vi "SISE-Analyser100.vi"() -> ()   [LabVIEW 2024]
uses:
  <vilib>/Analysis/NI_AALPro.lvlib
panel:
  out "Buffer Mobilty ch2":dbl
  out "pKs ch2":dbl
  in  "Main Tab Control":T1(tab)
  out "Event marks":string
  in  "Raw data file in":path
  out "Trace length":dbl
  out "# of traces":dbl
  out "Trace #":dbl
  in  "Scroll back":bool
  in  "Step back":bool
  in  "Step forward":bool
  in  "Scroll forward":bool
  in  "Module selection view data":enum16{"Load data", "Scroll data"}(ring)
  out "Load data":bool
  in  "Scroll speed":dbl(slide)=10.000000000000002 scale=1.0..100.0
  out "Scroll data":bool
  out "SISE 1 channel":bool
  out "Voltage 2 channel":bool
  out "Voltage 1 channel":bool
  out "SISE 2 channel":bool
  out "Scan distance, µm":dbl
  out "Scan angle, degrees":dbl
  out "Record period (single track), s s):":dbl
  out "Position probe":cluster{dbl[], dbl[]}[](graph)
  in  "?":T2(tab)
  out "Vprobe SISE 1":cluster{dbl[], dbl[]}[](graph)
  out "Vprobe SISE 2":cluster{dbl[], dbl[]}[](graph)
  out "Vprobe V 1":cluster{dbl[], dbl[]}[](graph)
  out "Vprobe V 2":cluster{dbl[], dbl[]}[](graph)
  in  "?":enum32{"dV SISE 1", "dV SISE 2"}(tab)
  out "deltaV SISE 1":cluster{dbl[], "Best Linear Fit":dbl[]}[](graph)
  out "deltaV SISE 2":cluster{dbl[], "Best Linear Fit":dbl[]}[](graph)
  in  "Start fit (% of rec. period)":dbl(slide)=50.0 scale=0.0..100.0
  in  "TC 3":T3(tab)
  in  "Range limit\nS1.1 (mV)":dbl(slide)=200.0 min=0.0 max=600.0 scale=0.2..600.0
  in  "Base line\nS1.1 (mV)":dbl(slide) scale=-300.0..300.0
  in  "Range limit\nS1.2 mV":dbl(slide)=30.0 scale=0.03..200.0
  in  "Base line \nS1.2 (mV)":dbl(slide) scale=-15.0..15.0
  out "dV-SISE channel 1":cluster{dbl[], dbl[]}[](graph)
  out "V-SISE channel 1":cluster{dbl[], dbl[]}[](graph)
  out "V-SISE channel 2":cluster{dbl[], dbl[]}[](graph)
  out "dV-SISE channel 2":cluster{dbl[], dbl[]}[](graph)
  in  "Range limit\nS2.1 (mV)":dbl(slide)=200.0 min=0.0 max=600.0 scale=0.2..600.0
  in  "Base line\nS2.1 (mV)":dbl(slide) scale=-300.0..300.0
  in  "Base line \nS2.2 (mV)":dbl(slide) scale=-15.0..15.0
  in  "Range limit\nS2.2 (mV)":dbl(slide)=30.0 scale=0.0..30.0
  out "Voltage channel 1":cluster{dbl[], dbl[]}[](graph)
  in  "Base line\nV1 (V)":dbl(slide) scale=-300.0..300.0
  in  "Range limit\nV1 (V)":dbl(slide)=200.0 min=0.0 max=600.0 scale=0.2..600.0
  in  "Base line\nV2 (V)":dbl(slide) scale=-300.0..300.0
  in  "Range limit\nV2 (V)":dbl(slide)=200.0 min=0.0 max=600.0 scale=0.2..600.0
  out "Voltage channel 2":cluster{dbl[], dbl[]}[](graph)
  in  "Zoom from end":dbl(slide)=100.0 scale=0.0..100.0
  in  "Zoom from start":dbl(slide) scale=0.0..100.0
  in  "Calibration-channel SISE1/2":enum32{"SISE channel 1", "SISE channel 2"}(tab)
  out "Update graphs ch1":bool
  in  "Module selection (Calibration window channel 1)":T4(ring)
  in  "Ion conc. ch1 (mM)":dbl
  out "Valency ch1":dbl
  out "Ion species ch1":bool
  out "Ion mobilty ch1":dbl
  in  "Ion Species ch1":u16(ring) items=["none", "H+", "K+", "NH4+", "Na+", "Cl-", "NO3-", "Ca2+", "Mg2+"]
  out "Calibration ch1":bool
  out "Slope ch1":dbl
  out "Intercept ch1":dbl
  out "?":cluster{dbl[], dbl[]}[](graph)
  out "Point #":dbl[](array[numeric])=[1.0, 2.0, 3.0, 4.0, 5.0]
  in  "Array in":dbl[][](array[numeric])
  out "Geometry ch1":bool caption="Geometry"
  out "Corrected \ndistance ch1":dbl caption="Corrected \ndistance"
  in  "Tab Control Geo 1":enum32{"flat surface", "cylinder", "sphere"}(tab)
  in  "Scan Distance  Flat (µm) 1":dbl
  in  "Scan distance cyl. (µm) 1":dbl caption="Scan distance cyl. (µm)"
  in  "Radius of object cyl. (µm) 1":dbl caption="Radius of object cyl. (µm)"
  in  "Minimum distance to object cyl. (µm) 1":dbl caption="Minimum distance to object cyl. (µm)"
  in  "Minimum distance to object sphere (µm) 1":dbl caption="Minimum distance to object sphere (µm)"
  in  "Radius of object sphere (µm) 1":dbl caption="Radius of object sphere (µm)"
  in  "Scan distance sphere (µm) 1":dbl caption="Scan distance sphere (µm)"
  out "Ion conc. SISE channel 1":cluster{dbl[], dbl[]}[](graph)
  in  "Range limit\nS1.3 (mM)":dbl(slide)=200.0 min=0.0 max=600.0 scale=1e-09..100.0
  in  "Base line\nS1.3 (mM)":dbl(slide) scale=-100.0..100.0
  out "Ion flux SISE channel 1":cluster{dbl[], dbl[]}[](graph)
  in  "Base line \nS1.4":dbl(slide) scale=-15.0..15.0
  in  "Range limit\nS1.4":dbl(slide)=1080.8651170969697 scale=0.03..3000.0
  out "?":string
  in  "Bildlaufleiste":i32(c297)
  in  "Zoom from end (Cal. modul) ch1":dbl(slide)=100.0 caption="Zoom from end" scale=0.0..100.0
  in  "Zoom from start (Cal. modul) ch1":dbl(slide) caption="Zoom from start" scale=0.0..100.0
  out "Update graphs ch2":bool
  in  "Ion conc. ch2 (mM)":dbl
  out "Valency ch2":dbl
  out "Ion species ch2":bool
  out "Ion mobilty ch2":dbl
  in  "Ion Species ch2":u16(ring) items=["none", "H+", "K+", "NH4+", "Na+", "Cl-", "NO3-", "Ca2+", "Mg2+"]
  out "Calibration ch2":bool
  out "Slope ch2":dbl
  out "Intercept ch2":dbl
  out "?":cluster{dbl[], dbl[]}[](graph)
  out "Point # 2":dbl[](array[numeric])=[1.0, 2.0, 3.0, 4.0, 5.0]
  in  "Array in 2":dbl[][](array[numeric])
  out "Geometry 2":bool caption="Geometry"
  out "Corrected \ndistance ch2":dbl caption="Corrected\ndistance"
  in  "Tab Control Geo 2":enum32{"flat surface", "cylinder", "sphere"}(tab)
  in  "Scan Distance  Flat (µm) 2":dbl caption="Scan Distance  Flat (µm)"
  in  "Scan distance cyl. (µm) 2":dbl caption="Scan distance cyl. (µm)"
  in  "Radius of object cyl. (µm) 2":dbl caption="Radius of object cyl. (µm)"
  in  "Minimum distance to object cyl. (µm) 2":dbl caption="Minimum distance to object cyl. (µm)"
  in  "Minimum distance to object sphere (µm) 2":dbl caption="Minimum distance to object sphere (µm)"
  in  "Radius of object sphere (µm) 2":dbl caption="Radius of object sphere (µm)"
  in  "Scan distance sphere (µm) 2":dbl caption="Scan distance sphere (µm)"
  in  "Bildlaufleiste 2":i32(c297)
  out "?":string
  out "Ion conc. SISE channel 2":cluster{dbl[], dbl[]}[](graph)
  in  "Range limit\nS2.3 (mM)":dbl(slide)=200.0 min=0.0 max=600.0 scale=1e-09..600.0
  in  "Base line\nS2.3 (mM)":dbl(slide) scale=-100.0..100.0
  out "Ion flux SISE channel 2":cluster{dbl[], dbl[]}[](graph)
  in  "Base line \nS2.4":dbl(slide) scale=-15.0..15.0
  in  "Range limit\nS2.4":dbl(slide)=1021.2709042717592 scale=0.03..3000.0
  in  "Module selection (Calibration window channel 2)":T4(ring)
  in  "Zoom from end (Cal. modul) 2":dbl(slide)=100.0 caption="Zoom from end" scale=0.0..100.0
  in  "Zoom from start (Cal. modul) 2":dbl(slide) caption="Zoom from start" scale=0.0..100.0
  in  "SISE channel selection (buffer corr.)":T5(tab)
  in  "Module selection ch1 (buffer corr.)":T6(ring)
  out "Buffer species ch1":bool
  out "Buffer conc. ch1":bool
  in  "Select buffer ch1":T7(ring)
  out "Buffer Mobilty ch1":dbl
  out "pKs ch1":dbl
  in  "Buffer conc. ch1 (mM)":dbl
  out "?":string
  in  "Bildlaufleiste 3":i32(c297)
  out "Ion flux (buffer corr.) SISE channel 1":cluster{dbl[], dbl[]}[](graph)
  in  "Base line \nS2.4 3":dbl(slide) scale=-15.0..15.0
  in  "Range limit\nS2.4 3":dbl(slide)=30.0 scale=0.03..5000.0
  out "Update graphs (buffer corr.) ch1":bool
  in  "Zoom from end (Buffer corr. modul) ch1":dbl(slide)=100.0 caption="Zoom from end" scale=0.0..100.0
  in  "Zoom from start (Buffer corr. modul) ch1":dbl(slide) caption="Zoom from start" scale=0.0..100.0
  in  "Module selection ch2 (buffer corr.)":T6(ring)
  out "Buffer species ch2":bool
  out "Buffer conc. ch2":bool
  in  "Buffer conc. ch2 (mM)":dbl
  in  "Range limit\nS2.4 2":dbl(slide)=30.0 scale=0.03..300.0
  in  "Base line \nS2.4 2":dbl(slide) scale=-15.0..15.0
  out "Ion flux (buffer corr.) SISE channel 2":cluster{dbl[], dbl[]}[](graph)
  out "Update graphs (buffer corr.) ch2":bool
  out "?":string
  in  "Bildlaufleiste 4":i32(c297)
  in  "Zoom from start (Buffer corr. modul) ch2":dbl(slide) caption="Zoom from start" scale=0.0..100.0
  in  "Zoom from end (Buffer corr. modul) ch2":dbl(slide)=100.0 caption="Zoom from end" scale=0.0..100.0
  in  "Select buffer ch 2":T7(ring)
  out "Next data file/exit program":bool
  in  "Exit program":bool
  out "Create analysis file":bool
  out "Indicate output":bool[](array[boolean])
  in  "Select output":bool[](array[boolean])=[TRUE, TRUE, TRUE, TRUE, TRUE, TRUE, TRUE, TRUE, TRUE, TRUE, TRUE, TRUE, TRUE, TRUE]
  in  "Analysis output file":path
  out "Raw data file":path
  out "Cluster 3":cluster{string[], bool[]}
  in  "Next data file":bool
  in  "Save data":bool
  out "Save analyses file":bool
  in  "Module selection Save Data":T8(ring)
  # "Event marks"
  # "Point (#)       Conc. (mM )      Vm (mV)"
  # "Event marks"
  # "Point (#)       Conc. (mM )      Vm (mV)"
  # "Event marks"
  # "Event marks"
  # "Output signals available                                                               Select output signals"
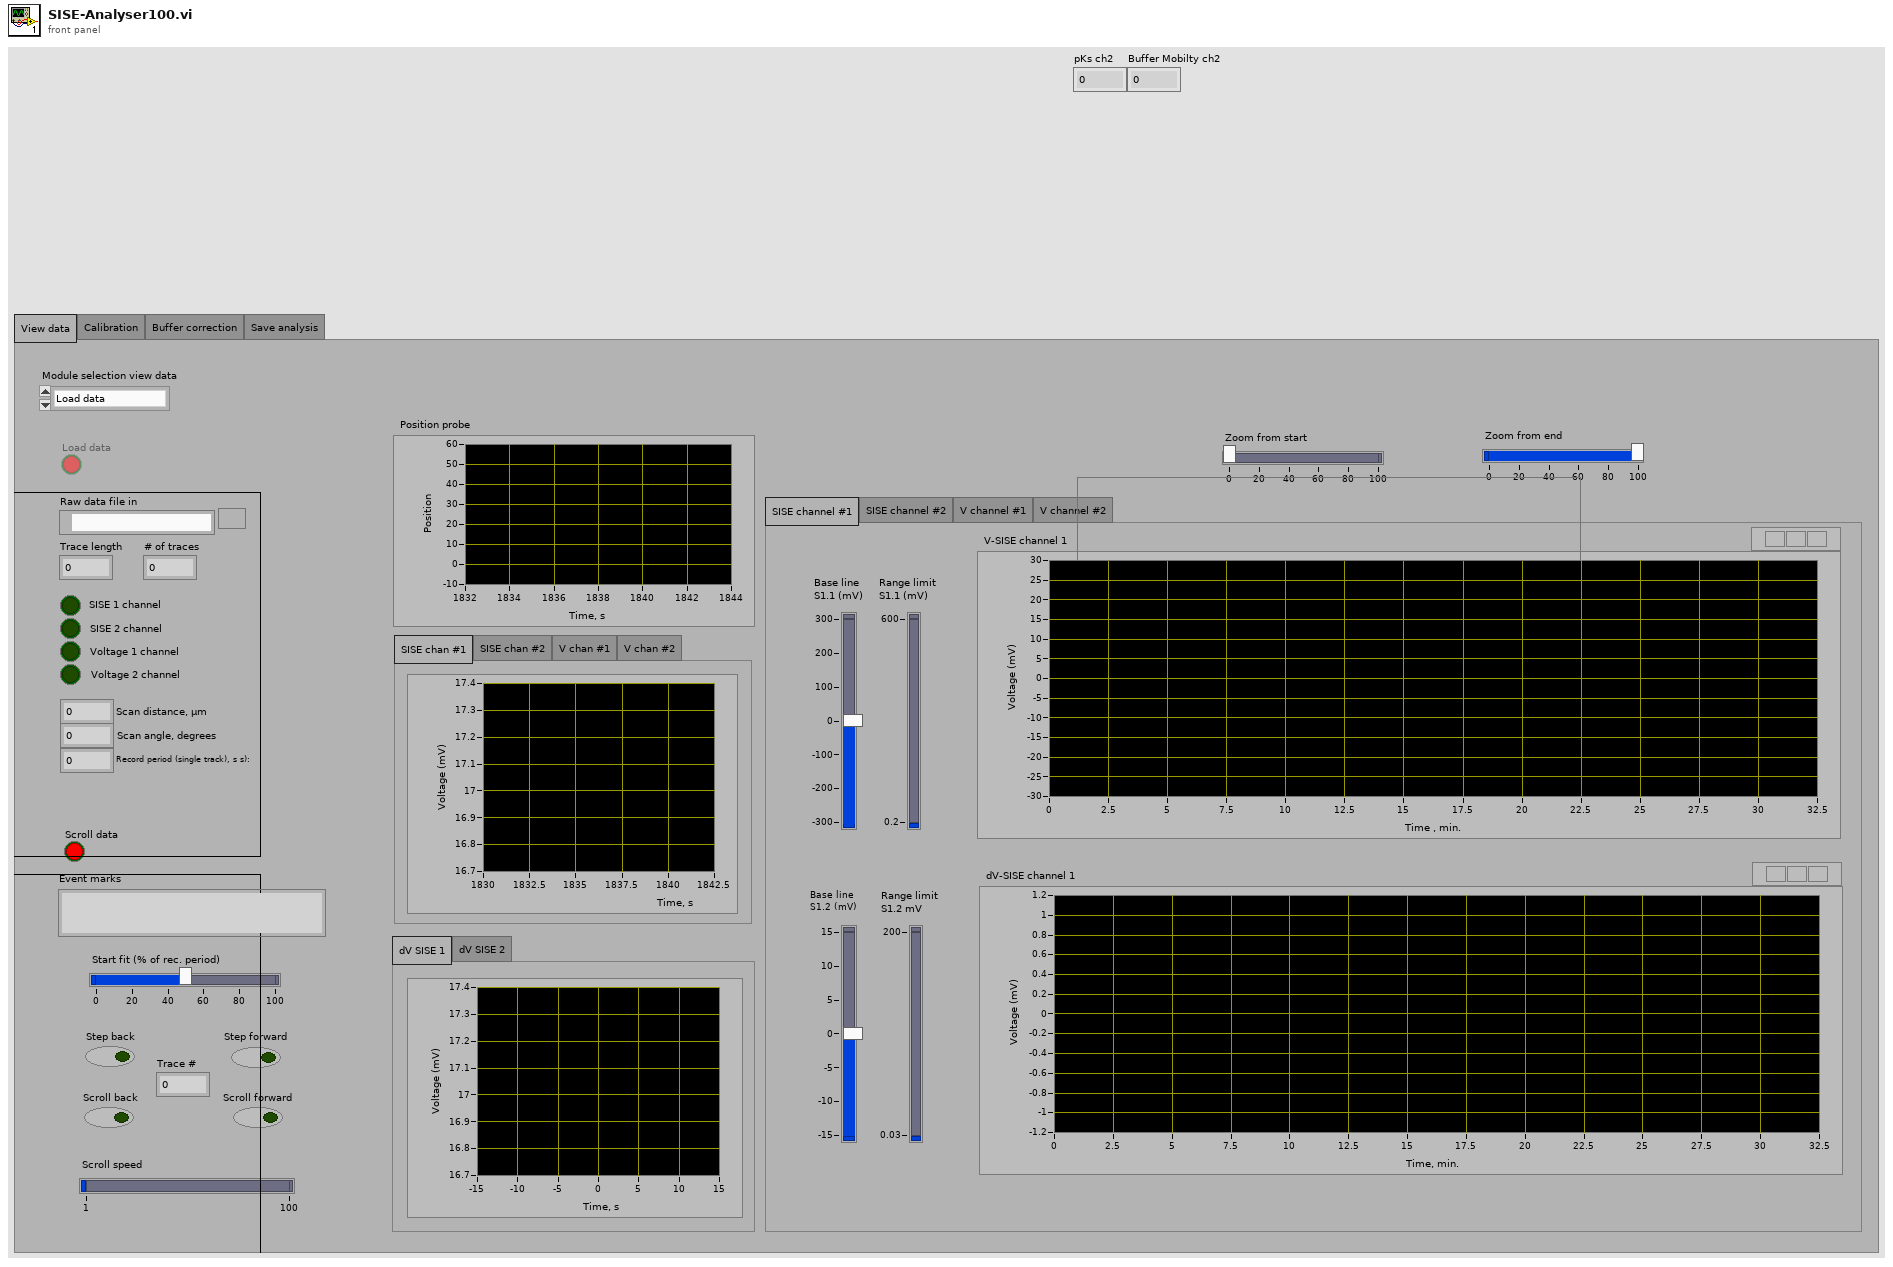
[diagram p1: front panel]
types:
  T1 = enum32{"View data", "Calibration", "Buffer correction", "Save analysis"}
  T2 = enum32{"SISE chan #1", "SISE chan #2", "V chan #1", "V chan #2"}
  T3 = enum32{"SISE channel #1", "SISE channel #2", "V channel #1", "V channel #2"}
  T4 = enum16{"Ion species", "Calibrate", "Geometry", "Update graphs"}
  T5 = enum32{"SISE channel 1, buffer corr.", "SISE channel 2, buffer corr."}
  T6 = enum16{"Buffer species", "Buffer conc.", "Update graphs"}
  T7 = enum16{"none", "Mes", "Malate (pH 5)", "Citrate (pH 5)", "TRIS", "HEPES"}
  T8 = enum16{"Create analysis file", "Save data", "New/stop analysis"}
  T9 = enum8{"Enabled", "Disabled", "Disabled and Grayed Out"}
  T10 = enum16{"open", "replace", "create", "open or create", "replace or create", "replace or create with confirmation"}
  T11 = cluster{path, "Referenz (Ausgang)":refnum<file>, bool, i32, string}
  T12 = cluster{path, "Referenz (Ausgang)":refnum<file>, bool, i32, string}[]
  T13 = cluster{"Raw data file in":path, "refnum out":refnum<file>, "status":bool, "code":i32, "source":string}
  T14 = cluster{dbl[][], dbl[], cluster{string[], bool[]}, dbl[][], cluster{dbl, string}[]}
  T15 = cluster{dbl[], dbl[], "Best Linear Fit":dbl[], dbl[], dbl[]}
  T16 = cluster{"Array (Ausgang)":dbl[], "Array (Ausgang)":dbl[]}
  T17 = cluster{"Array (Ausgang)":dbl[], "Array (Ausgang)":dbl[]}[]
  T18 = cluster{"dup path":path, "refnum":refnum<file>, "status":bool, "code":i32, "source":string}
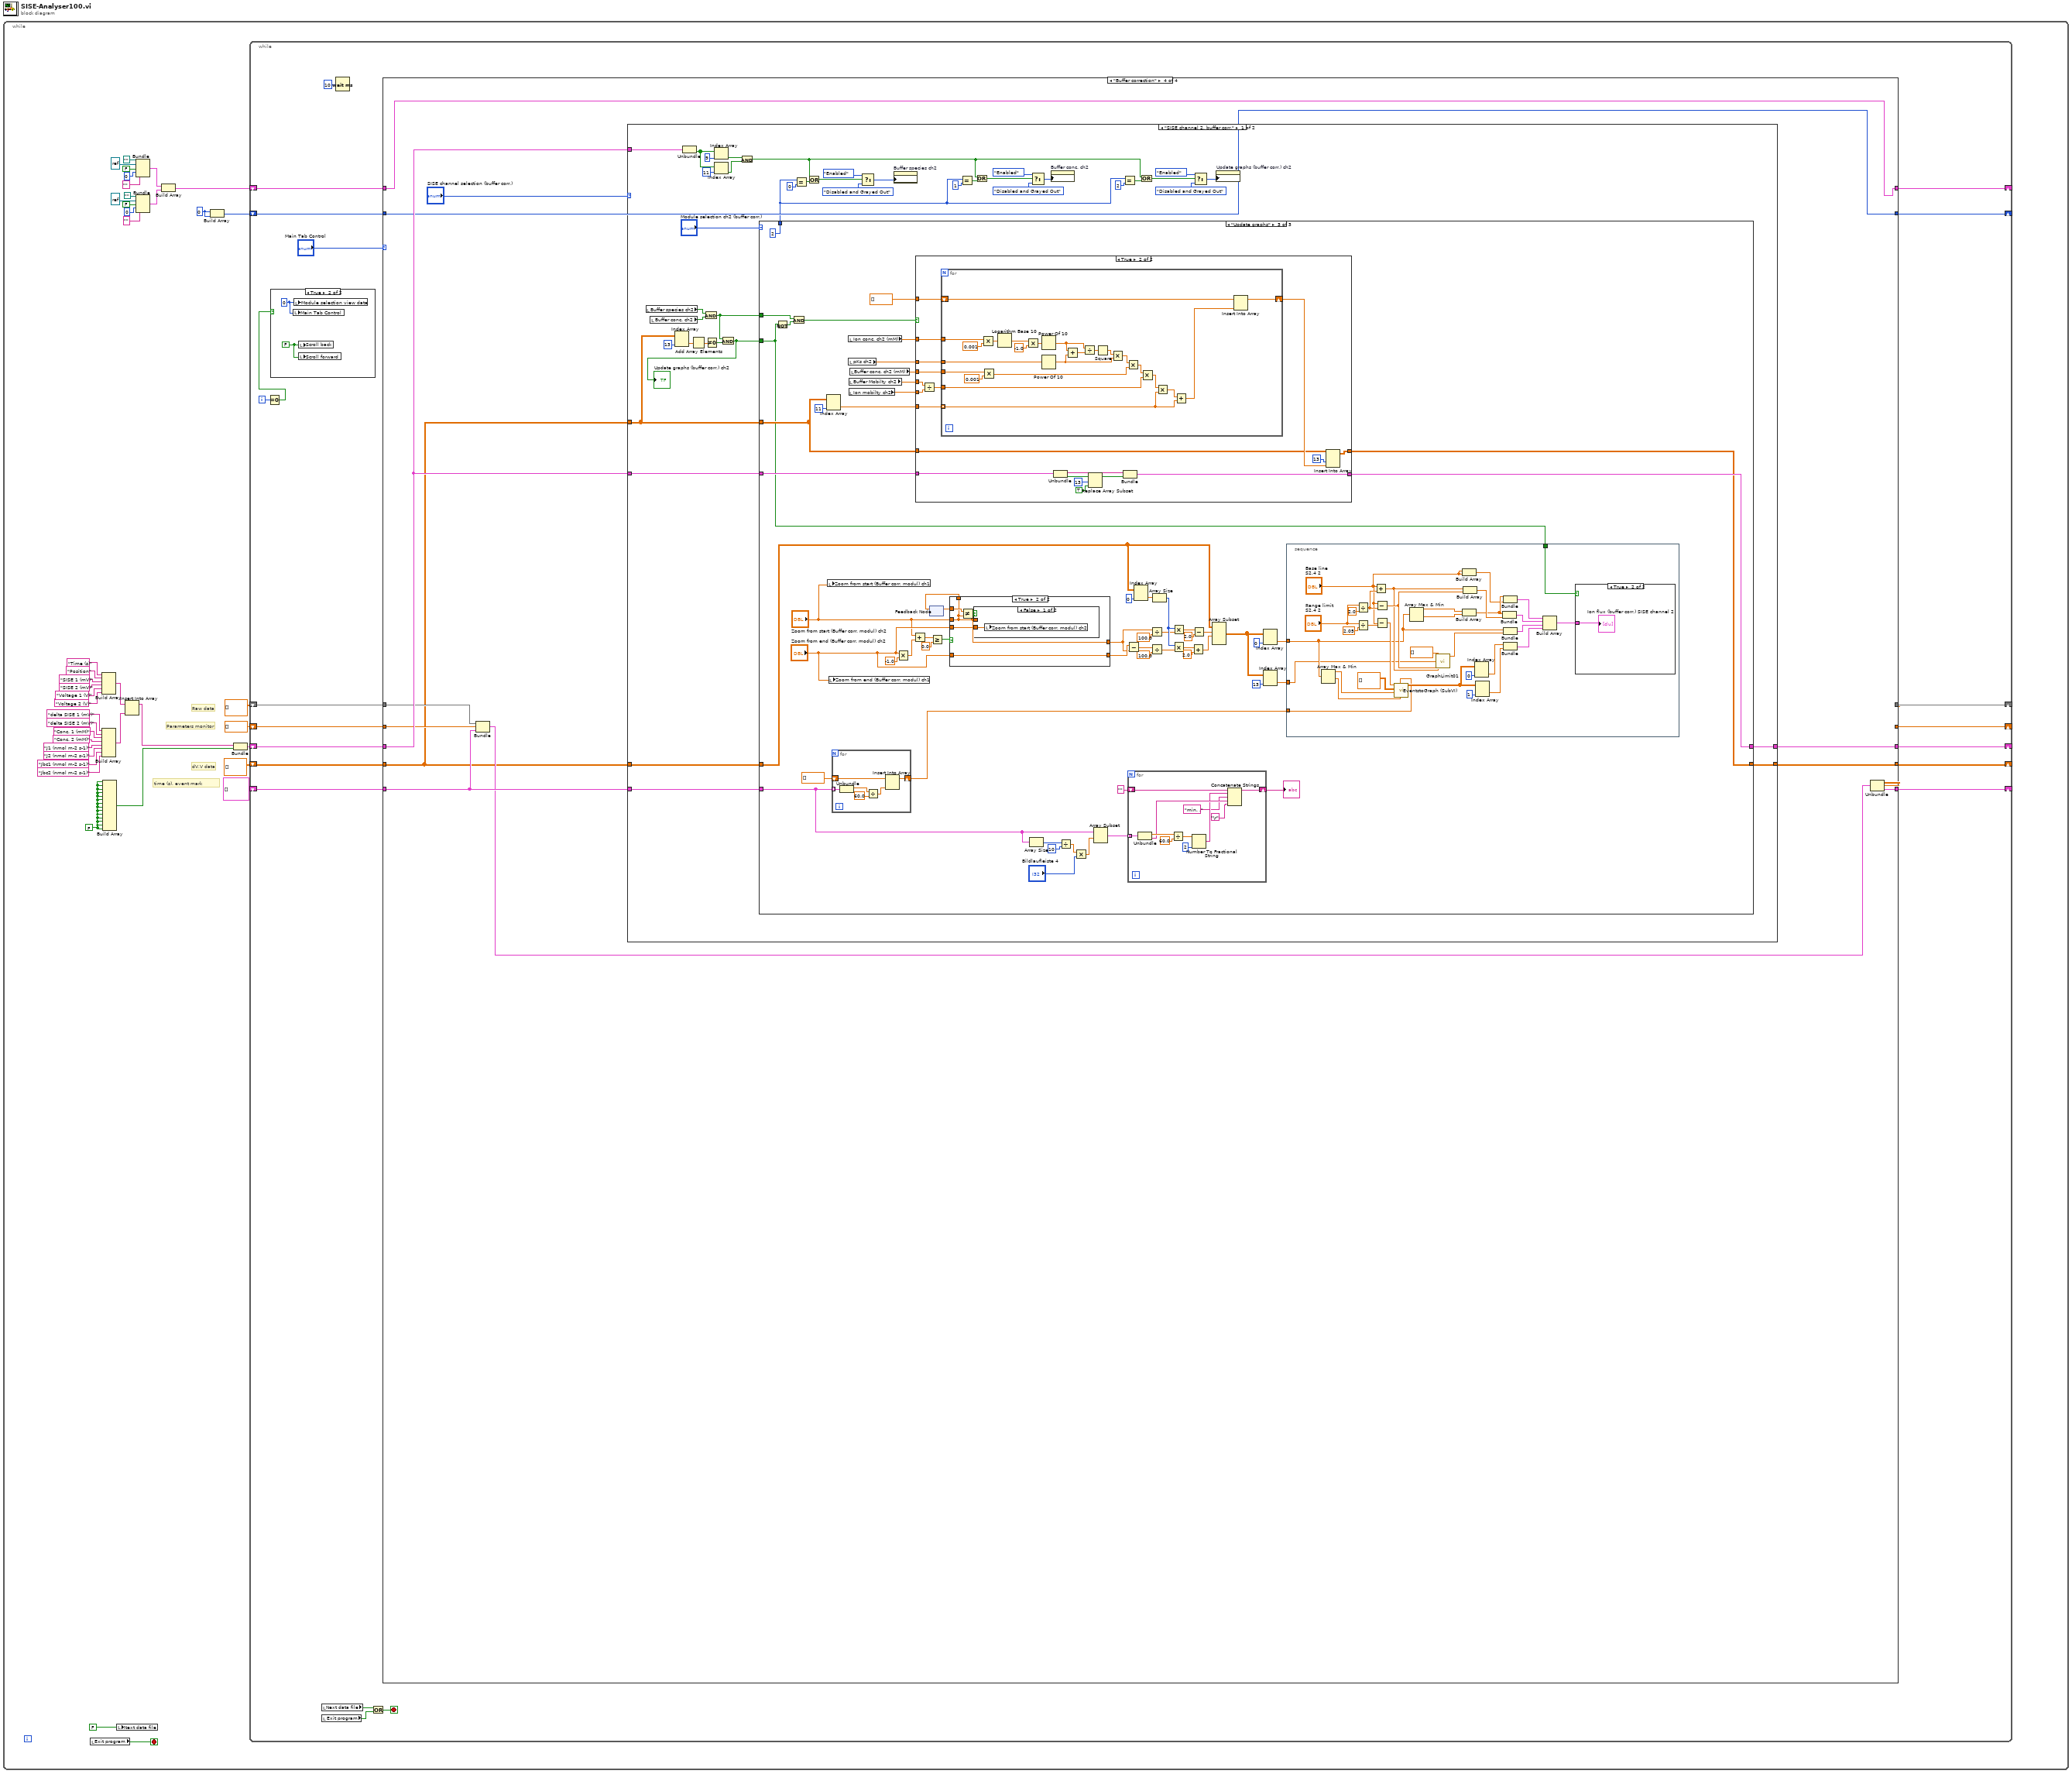
[diagram p0: block diagram]
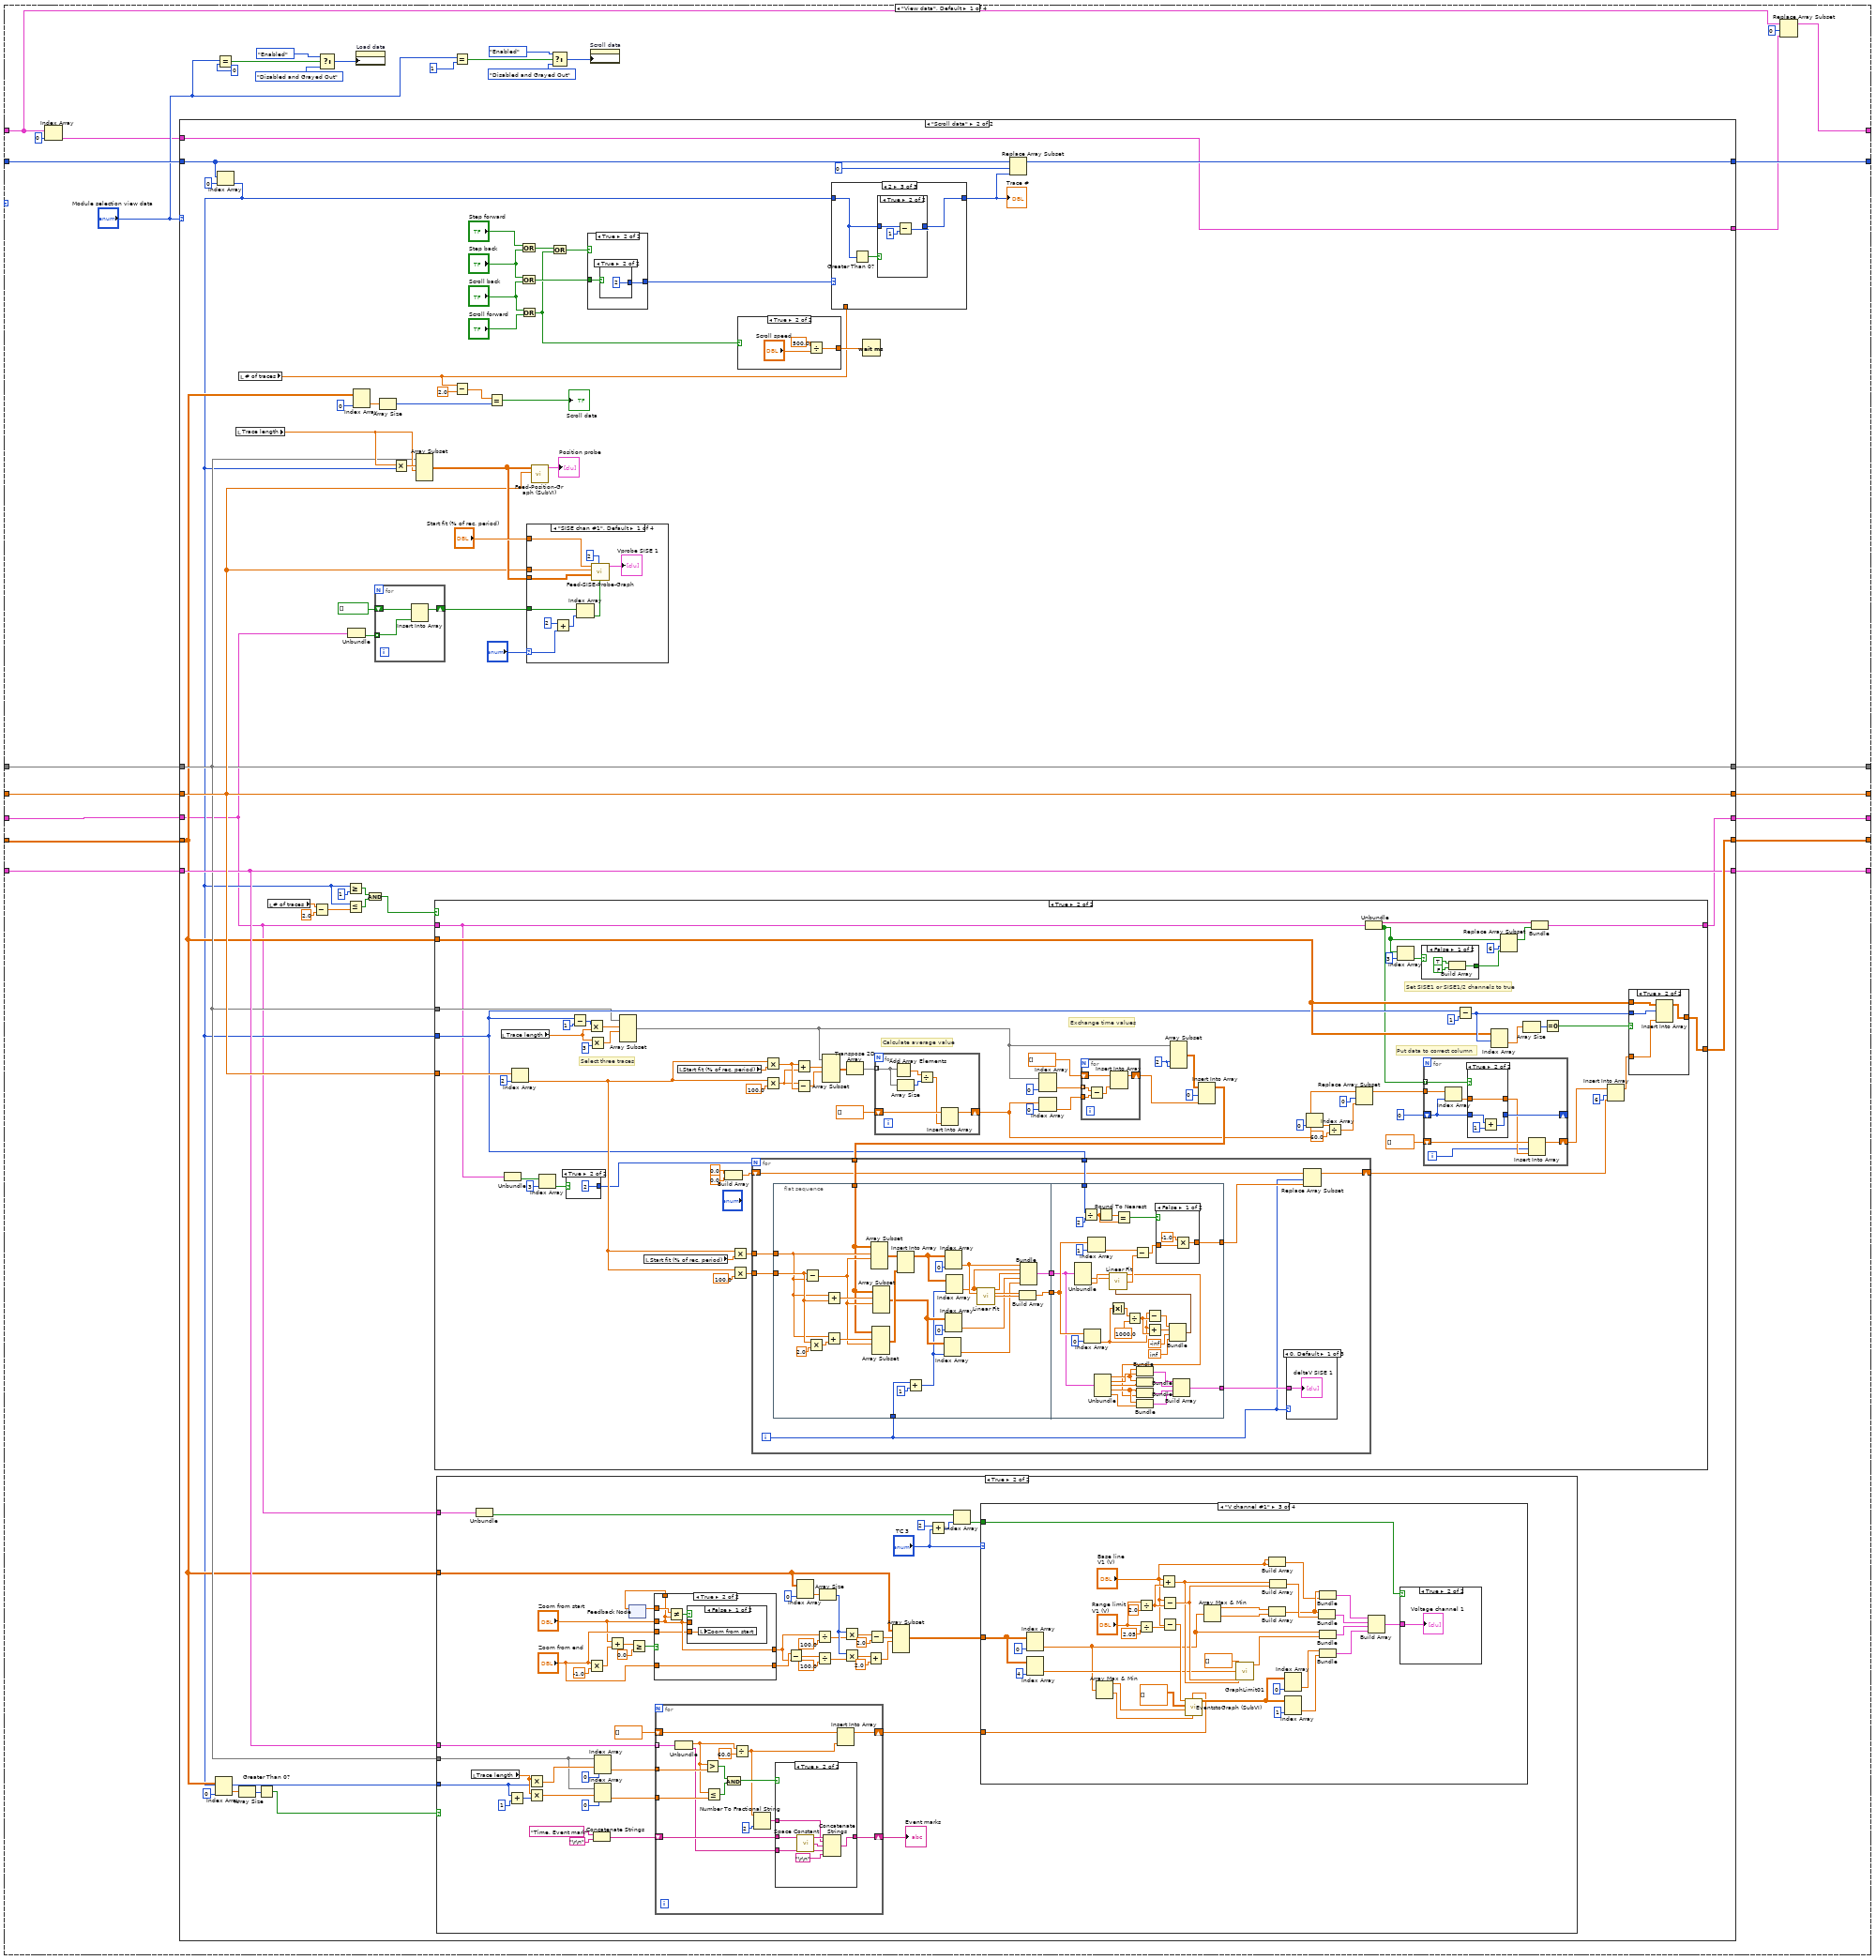
[diagram p3: hidden frame]
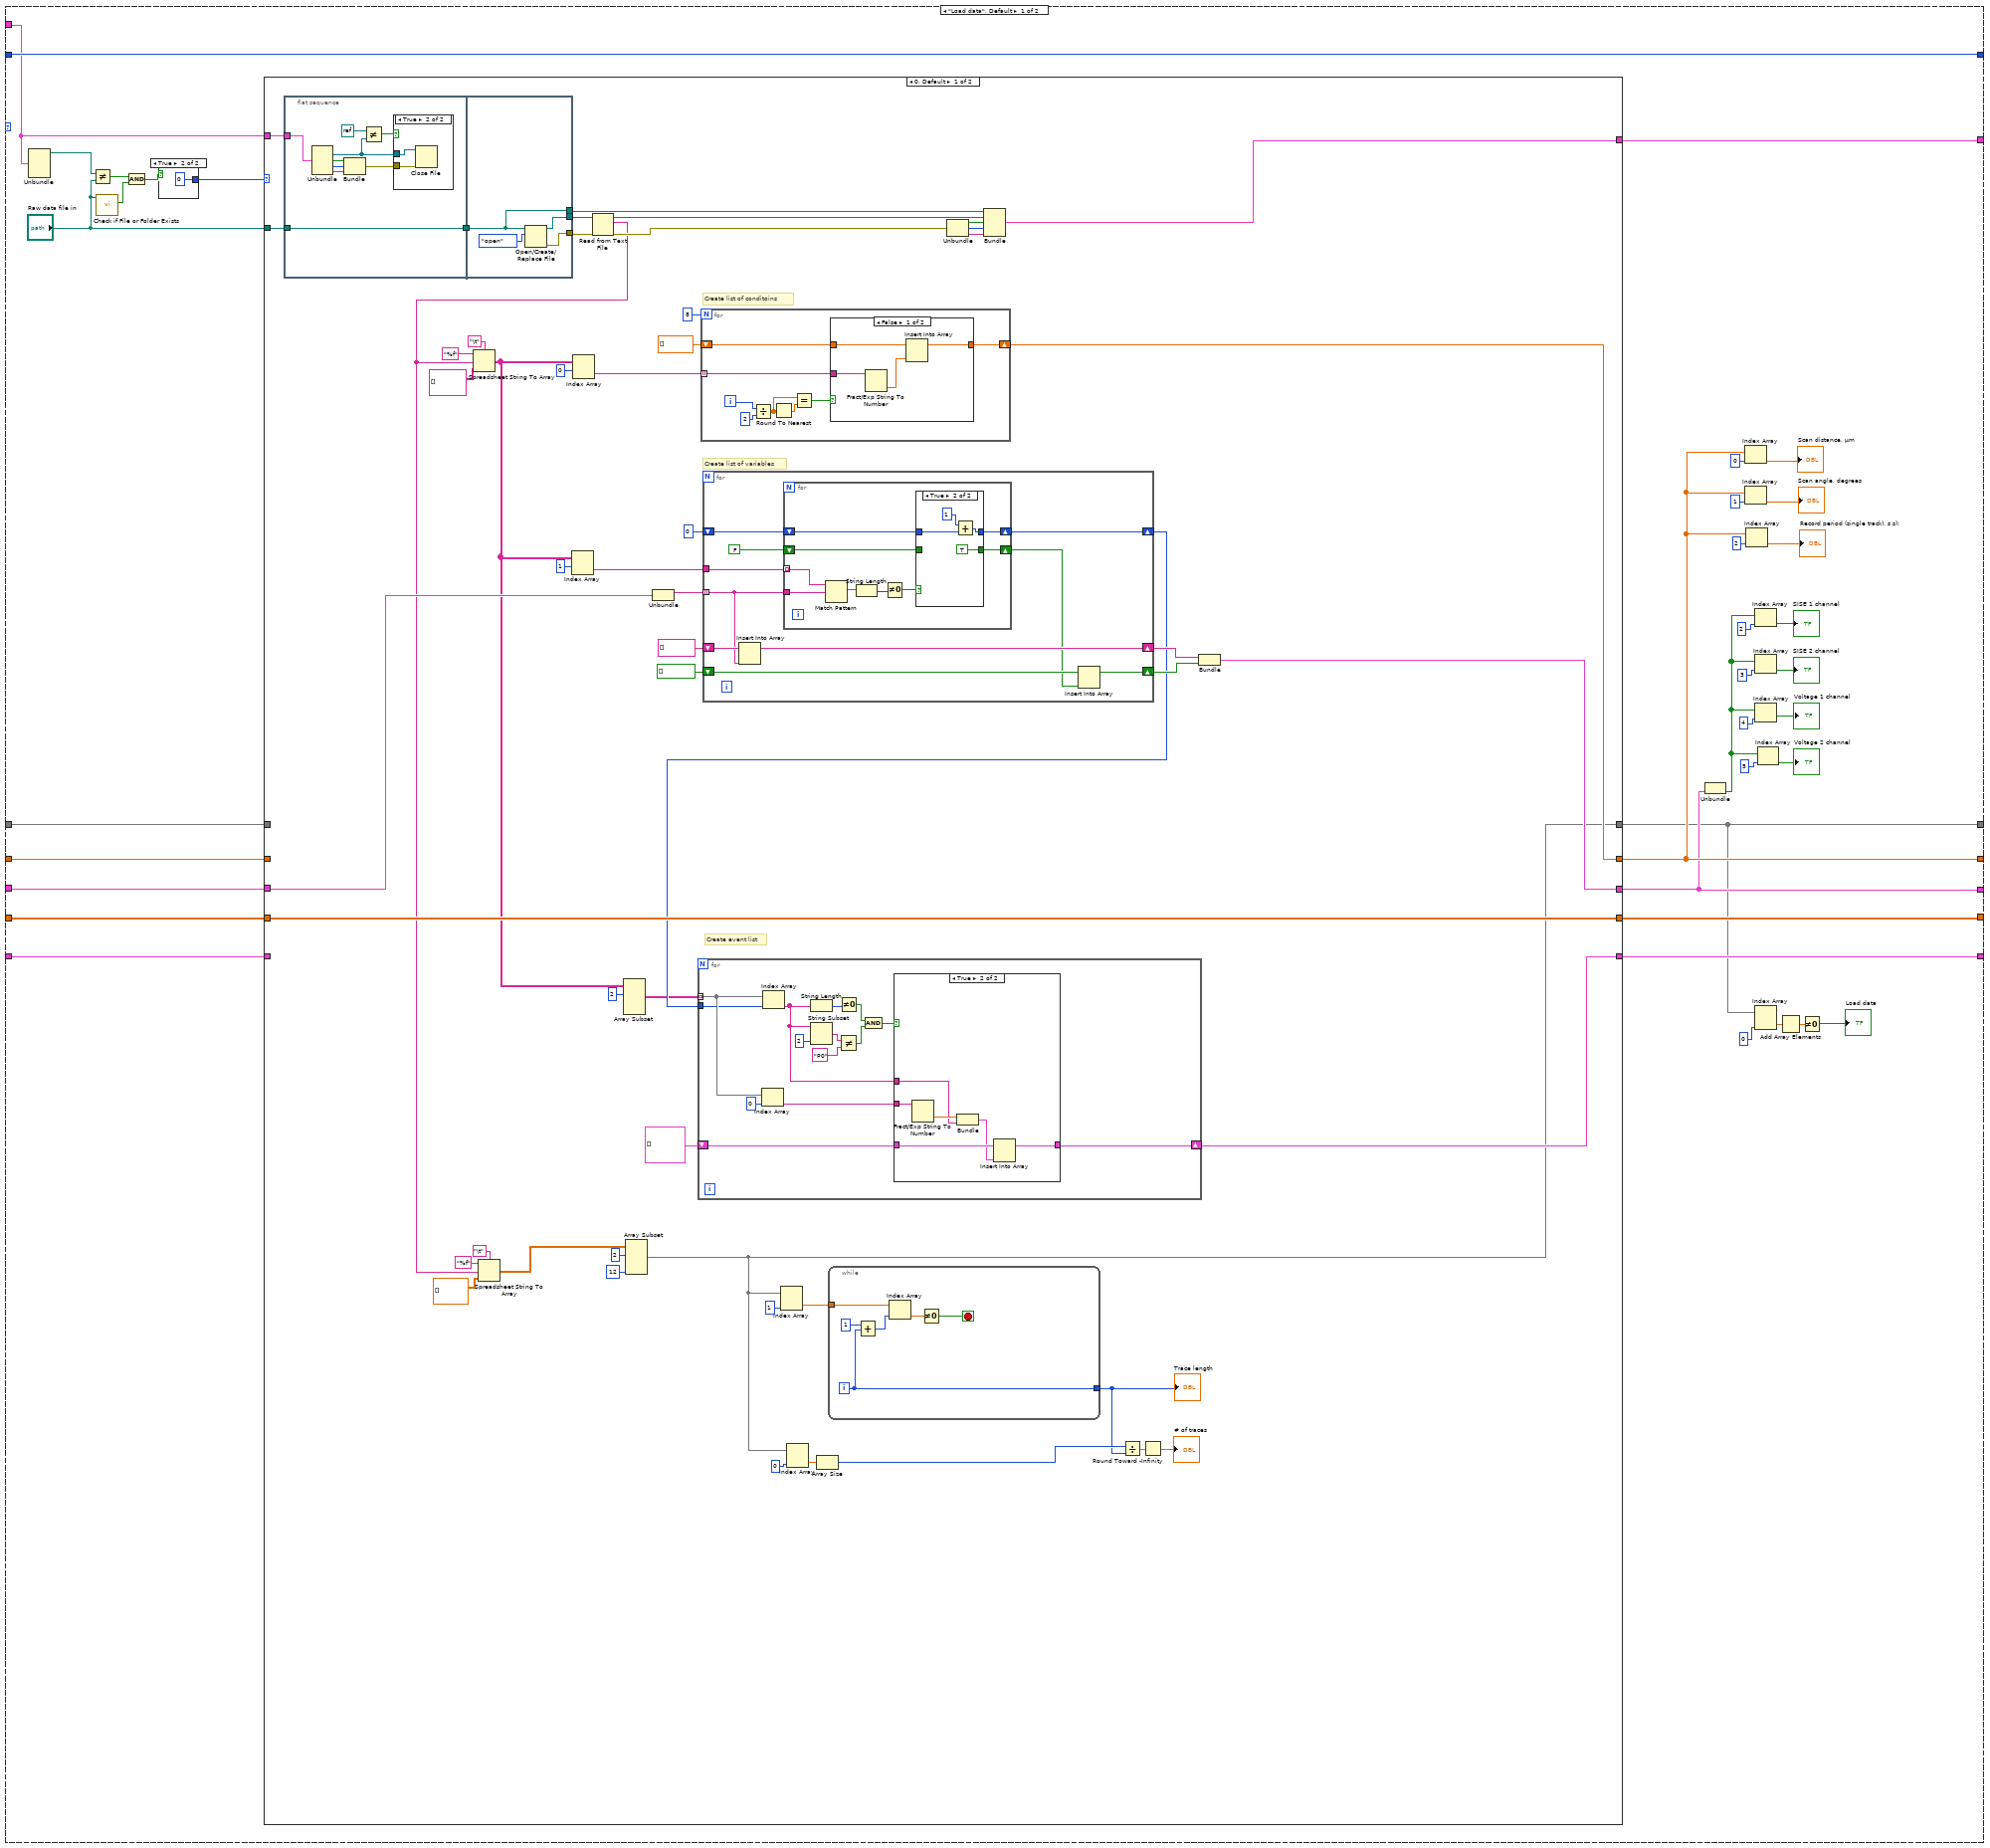
[diagram p4: hidden frame]
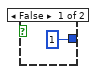
[diagram p5: hidden frame]
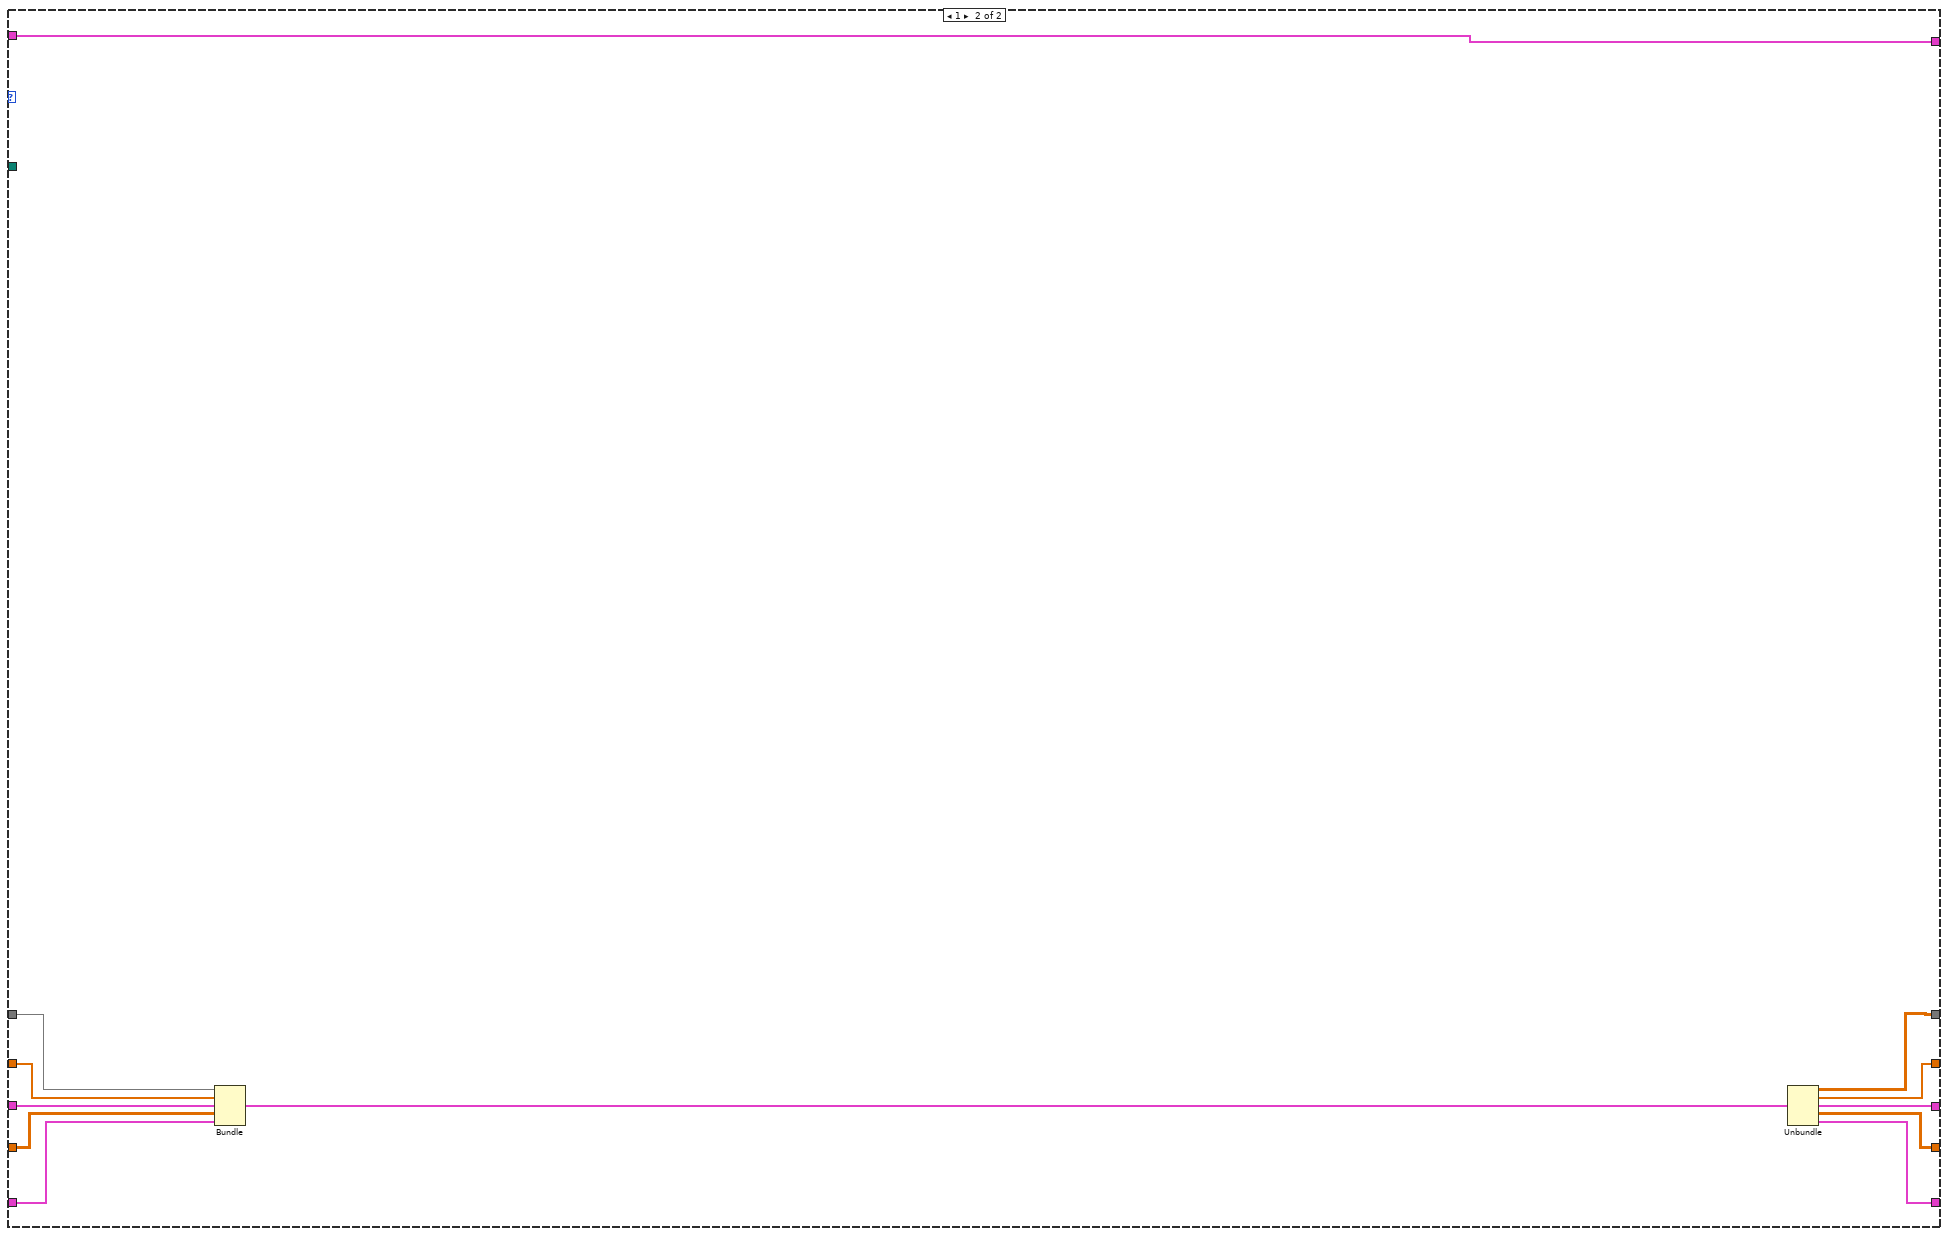
[diagram p10: hidden frame]
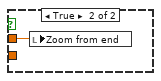
[diagram p13: hidden frame]
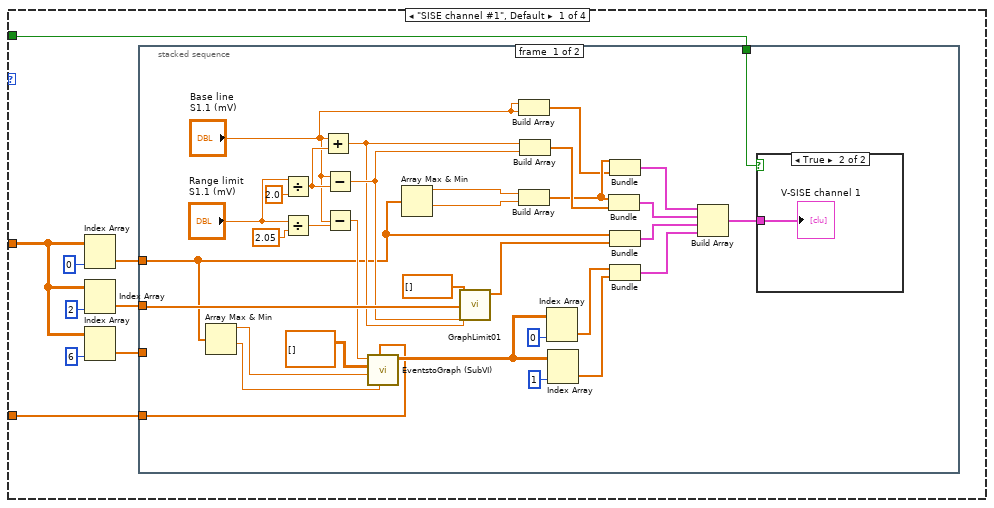
[diagram p14: hidden frame]
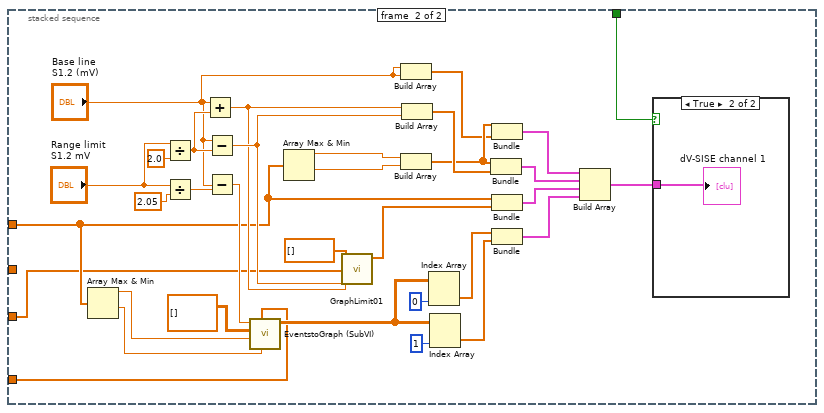
[diagram p16: hidden frame]
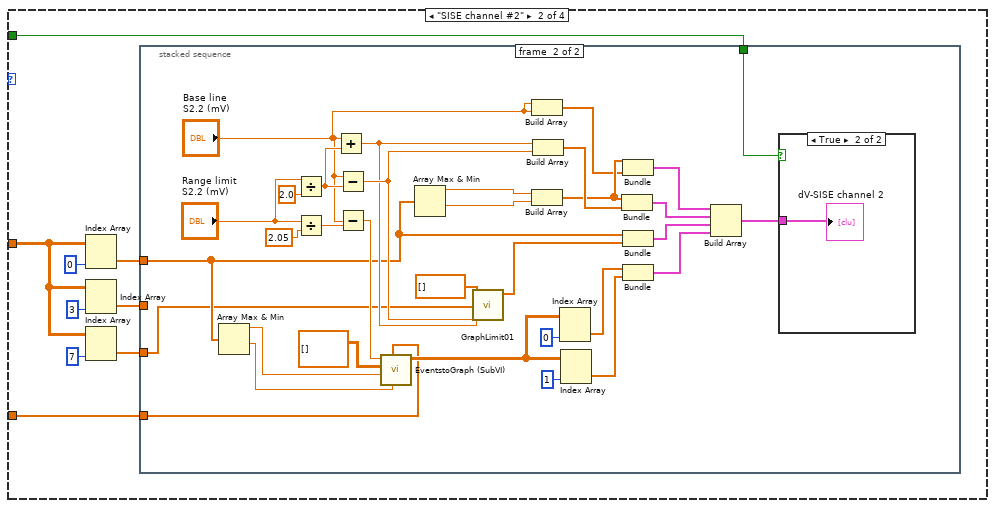
[diagram p18: hidden frame]
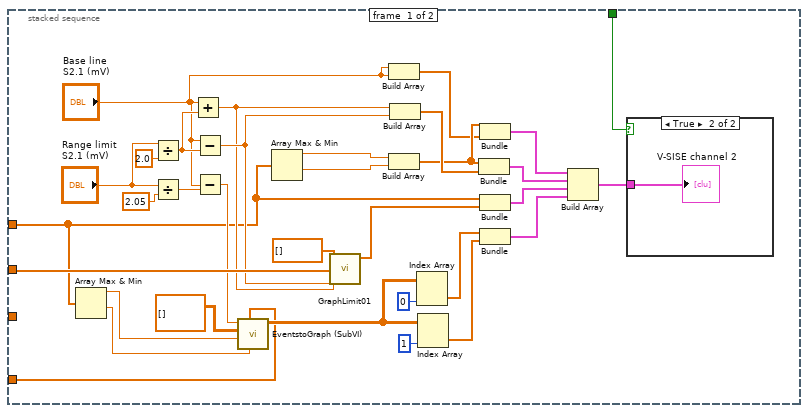
[diagram p19: hidden frame]
diagram:
  n1 = while {
    stop <- w17 stop-if-true
    w19 = FALSE
    w16 = 0
    # "time (s), event mark"
    # "Parameters monitor"
    # "dV,V data"
    # "Raw data"
    n2 = local read "Exit program"() -> (w17:bool)
    n3 = Build Array("Time (s)", "Position", "SISE 1 (mV)", "SISE 2 (mV)", "Voltage 1 (V)", "Voltage 2 (V)") -> (w26:string[])
    n4 = Build Array("delta SISE 1 (mV)", "delta SISE 2 (mV)", "Conc. 1 (mM)", "Conc. 2 (mM)", "J1 (nmol m-2 s-1)", "J2 (nmol m-2 s-1)", "Jbc1 (nmol m-2 s-1)", "Jbc2 (nmol m-2 s-1)") -> (w25:string[])
    n5 = Build Array(w19, w19, w19, w19, w19, w19, w19, w19, w19, w19, w19, w19, w19, w19) -> (w18:bool[])
    n6 = local write "Next data file"(FALSE) -> ()
    n7 = Insert Into Array(array=w26, new element=w25) -> (w20:string[])  [unwired: 1 in]
    n8 = Bundle(path "", "Referenz (Ausgang)"=refnum<file> refnum, FALSE, 0, "") -> (w4:T11)  [unwired: 1 in]
    n9 = Bundle(path "", "Referenz (Ausgang)"=refnum<file> refnum, FALSE, 0, "") -> (w3:T11)  [unwired: 1 in]
    n10 = Build Array(w4, w3) -> (w2:T12)
    n11 = Build Array(w16, w16) -> (w15:i32[])
    n12 = Bundle(w20, w18) -> (w37:cluster{string[], bool[]})  [unwired: 1 in]
    n13 = while {
      shift-right: [w62] -> _
      shift-left: dbl[][] [] -> [w61]
      shift-right: [w58] -> _
      shift-left: dbl[][] [] -> [w59]
      shift-right: [w57] -> _
      shift-left: w37 -> [w42]
      shift-right: [w56] -> _
      shift-left: dbl[] [] -> [w55]
      shift-right: [w51] -> _
      shift-left: w15 -> [w46]
      shift-right: [w54] -> _
      shift-left: cluster{dbl, string}[] [] -> [w53]
      shift-right: [w43] -> _
      shift-left: w2 -> [w52]
      i -> [w45]
      stop <- w50 stop-if-true
      n14 = Equal To 0?(x=w45) -> (x = 0?=w44:bool)
      n15 = case shown="True" w44 {
        frame False {
        }
        frame True {
          w63 = FALSE
          w64 = 0
          n16 = local write "Main Tab Control"(w64) -> ()
          n17 = local write "Module selection view data"(w64) -> ()
          n18 = local write "Scroll back"(w63) -> ()
          n19 = local write "Scroll forward"(w63) -> ()
        }
      }
      n20 = local read "Next data file"() -> (w49:bool)
      n21 = local read "Exit program"() -> (w48:bool)
      n22 = Wait (ms)(milliseconds to wait=u32 10) -> ()  [unwired: 1 out]
      n23 = Or(x=w49, y=w48) -> (x .or. y?=w50:bool)
      n24 = case shown="\"Buffer correction\"" "Main Tab Control" {
        tunnel: w61 -> [w93 w930 w1129 w1813]
        tunnel: [w92 w925 w1135 w1825] -> w62
        tunnel: w59 -> [w73 w933 w1134 w1822]
        tunnel: [w81 w923 w1131 w1817] -> w58
        tunnel: w42 -> [w80 w931 w1124 w1824]
        tunnel: [w79 w927 w1125 w1823] -> w57
        tunnel: w55 -> [w78 w932 w1128 w1821]
        tunnel: [w77 w926 w1130 w1818] -> w56
        tunnel: w46 -> [w72 w916 w1122 w1815]
        tunnel: w53 -> [w76 w929 w1127 w1820]
        tunnel: [w75 w924 w1126 w1816] -> w54
        tunnel: w52 -> [w68 w902 w1123 w1814]
        tunnel: [w66 w900 w1123 w1814] -> w43
        tunnel: [w74 w916 w1122 w1815] -> w51
        frame "View data", Default {
          n25 = Index Array(array=w68, index=0 ("Index")) -> (element=w69:T11)
          n26 = case shown="\"Scroll data\"" "Module selection view data" {
            tunnel: w93 -> [w104 w288]
            tunnel: [w103 w306] -> w92
            tunnel: w73 -> [w127 w300]
            tunnel: [w102 w300] -> w81
            tunnel: w80 -> [w126 w279]
            tunnel: [w110 w287] -> w79
            tunnel: w78 -> [w121 w307]
            tunnel: [w117 w307] -> w77
            tunnel: w72 -> [w113 w283]
            tunnel: [w113 w284] -> w74
            tunnel: w76 -> [w112 w301]
            tunnel: [w111 w301] -> w75
            tunnel: w69 -> [w98 w280]
            tunnel: [w99 w280] -> w65
            frame "Load data", Default {
              n27 = Unbundle(w98) -> (w96:path)  [unwired: 4 out]
              n28 = Not Equal?(x=w96, y="Raw data file in") -> (x != y?=w101:bool)
              n29 = call <vilib>:"Check if File or Folder Exists.vi"("path"="Raw data file in") -> ("file or folder exists?"=w100:bool)  [unwired: 8 in, 2 out]
              n30 = And(x=w101, y=w100) -> (x .and. y?=w94:bool)
              n31 = case shown="True" w94 {
                tunnel: [1 0] -> w95
                frame False {
                }
                frame True {
                }
              }
              n32 = case shown="0, Default" w95 {
                tunnel: w127 -> [_ w276]
                tunnel: [w136 w268] -> w102
                tunnel: w126 -> [w159 w278]
                tunnel: [w158 w272] -> w110
                tunnel: w121 -> [_ w277]
                tunnel: [w167 w271] -> w117
                tunnel: w112 -> [_ w274]
                tunnel: [w155 w269] -> w111
                tunnel: w104 -> [w186 w275]
                tunnel: [w186 w270] -> w103
                tunnel: "Raw data file in" -> [w183 _]
                tunnel: [w179 w267] -> w99
                tunnel: w98 -> [w185 w267]
                frame 0, Default {
                  # "Create list of variables"
                  # "Create list of conditoins"
                  # "Create event list"
                  n33 = flat-sequence {
                    tunnel: w185 -> [w260]
                    tunnel: [w252] -> w184
                    tunnel: w183 -> [w252]
                    tunnel: [w264] -> w176
                    tunnel: [w265] -> w177
                    tunnel: w184 -> [w263]
                    tunnel: [w263] -> w178
                    frame #0 {
                      n34 = Unbundle(w260) -> ("Referenz (Ausgang)"=w253:refnum<file>, w257:bool, w258:i32, w259:string)  [unwired: 1 out]
                      n35 = Bundle(w257, w258, w259) -> (w256:errorcluster)  [unwired: 1 in]
                      n36 = Not Equal?(x=refnum<k0> refnum, y=w253) -> (x != y?=w254:bool)
                      n37 = case shown="True" w254 {
                        tunnel: w256 -> [_ w262]
                        tunnel: w253 -> [_ w261]
                        frame False {
                        }
                        frame True {
                          n38 = Close File(refnum=w261, error in=w262) -> ()  [unwired: 2 out]
                        }
                      }
                    }
                    frame #1 {
                      n39 = Open/Create/Replace File(file path (use dialog)=w263, operation (0:open)=T10."open") -> (refnum out=w265:refnum<file>, error out=w264:errorcluster)  [unwired: 4 in, 1 out]
                    }
                  }
                  n40 = Read from Text File(file (use dialog)=w177, error in=w176) -> (refnum out=w174:refnum<file>, text=w154:string, error out=w175:errorcluster)  [unwired: 2 in, 1 out]
                  n41 = Spreadsheet String To Array(delimiter (Tab)="\t", format string="%f", spreadsheet string=w154, array type (2D Dbl)=string[][] []) -> (array=w156:string[][])
                  n42 = Spreadsheet String To Array(delimiter (Tab)="\t", format string="%f", spreadsheet string=w154, array type (2D Dbl)=dbl[][] []) -> (array=w146:dbl[][])
                  n43 = Index Array(array=w156, index (row)=1 ("Index")) -> (element=w134:string[])  [unwired: 1 in]
                  n44 = Index Array(array=w156, index (row)=0 ("Index")) -> (element=w135:string[])  [unwired: 1 in]
                  n45 = Array Subset(array=w156, index (row)=2 ("Index")) -> (w152:string[][])  [unwired: 3 in]
                  n46 = Array Subset(array=w146, index (row)=2 ("index"), length (col)=12 ("Länge")) -> (w136:dbl[][])  [unwired: 2 in]
                  n47 = Unbundle(w159) -> (w164:string[])  [unwired: 1 out]
                  n48 = for {
                    N: 8 -> [_]
                    tunnel: w135 -> [w241] mode=indexing
                    shift-right: [w239] -> w167
                    shift-left: dbl[] [] -> [w240]
                    i -> [w246]
                    n49 = Divide(x=w246, y=2) -> (x/y=w243:dbl)
                    n50 = Round To Nearest(number=w243) -> (nearest integer value=w244:dbl)
                    n51 = Equal?(x=w243, y=w244) -> (x = y?=w242:bool)
                    n52 = case shown="False" w242 {
                      tunnel: w241 -> [w248 _]
                      tunnel: w240 -> [w250 w251]
                      tunnel: [w249 w251] -> w239
                      frame False {
                        n53 = Fract/Exp String To Number(string=w248) -> (number=w247:dbl)  [unwired: 3 in, 1 out]
                        n54 = Insert Into Array(array=w250, new element=w247) -> (w249:dbl[])  [unwired: 1 in]
                      }
                      frame True {
                      }
                    }
                  }
                  n55 = for {
                    tunnel: w164 -> [w217] mode=indexing
                    tunnel: w134 -> [w223]
                    shift-right: [w216] -> w160
                    shift-left: bool[] [] -> [w215]
                    shift-right: [w220] -> w157
                    shift-left: 0 -> [w221]
                    shift-right: [w219] -> w161
                    shift-left: string[] [] -> [w218]
                    n56 = Insert Into Array(array=w218, new element=w217) -> (w219:string[])  [unwired: 1 in]
                    n57 = for {
                      tunnel: w223 -> [w232] mode=indexing
                      tunnel: w217 -> [w231]
                      shift-right: [w226] -> w214
                      shift-left: FALSE -> [w228]
                      shift-right: [w224] -> w220
                      shift-left: w221 -> [w225]
                      n58 = Match Pattern(string=w232, regular expression=w231) -> (match substring=w230:string)  [unwired: 1 in, 3 out]
                      n59 = String Length(string=w230) -> (length=w229:i32)
                      n60 = Not Equal To 0?(x=w229) -> (x != 0?=w227:bool)
                      n61 = case shown="True" w227 {
                        tunnel: w228 -> [w234 _]
                        tunnel: [w234 TRUE] -> w226
                        tunnel: w225 -> [w233 w235]
                        tunnel: [w233 w237] -> w224
                        frame False {
                        }
                        frame True {
                          n62 = Add(x=1 ("y"), y=w235) -> (x+y=w237:i32)
                        }
                      }
                    }
                    n63 = Insert Into Array(array=w215, new element=w214) -> (w216:bool[])  [unwired: 1 in]
                  }
                  n64 = for {
                    tunnel: w152 -> [w197] mode=indexing
                    tunnel: w157 -> [w193]
                    shift-right: [w194] -> w155
                    shift-left: cluster{dbl, string}[] [] -> [w195]
                    n65 = Index Array(array=w197, index=0 ("Index")) -> (element=w196:string)
                    n66 = Index Array(array=w197, index=w193) -> (element=w199:string)
                    n67 = String Subset(string=w199, length (rest)=2 ("Länge (Rest)")) -> (substring=w204:string)  [unwired: 1 in]
                    n68 = String Length(string=w199) -> (length=w206:i32)
                    n69 = Not Equal?(x=w204, y="P0") -> (x != y?=w200:bool)
                    n70 = Not Equal To 0?(x=w206) -> (x != 0?=w202:bool)
                    n71 = And(x=w202, y=w200) -> (x .and. y?=w201:bool)
                    n72 = case shown="True" w201 {
                      tunnel: w199 -> [_ w211]
                      tunnel: w196 -> [_ w213]
                      tunnel: [w207 w210] -> w194
                      tunnel: w195 -> [w207 w209]
                      frame False {
                      }
                      frame True {
                        n73 = Fract/Exp String To Number(string=w213) -> (number=w212:dbl)  [unwired: 3 in, 1 out]
                        n74 = Bundle(w212, w211) -> (w208:cluster{dbl, string})  [unwired: 1 in]
                        n75 = Insert Into Array(array=w209, new element=w208) -> (w210:cluster{dbl, string}[])  [unwired: 1 in]
                      }
                    }
                  }
                  n76 = Index Array(array=w136, index (col)=1 ("disabled index (col)")) -> (element=w143:dbl[])  [unwired: 1 in]
                  n77 = Index Array(array=w136, index (col)=0 ("disabled index (col)")) -> (element=w141:dbl[])  [unwired: 1 in]
                  n78 = Array Size(array=w141) -> (size(s)=w140:i32)
                  n79 = while {
                    tunnel: w143 -> [w192]
                    tunnel: [w187] -> w138
                    i -> [w187]
                    stop <- w188 stop-if-true
                    n80 = Add(x=1, y=w187) -> (x+y=w191:i32)
                    n81 = Index Array(array=w192, index=w191) -> (element=w189:dbl)
                    n82 = Not Equal To 0?(x=w189) -> (x != 0?=w188:bool)
                  }
                  "Trace length" <- w138
                  n83 = Unbundle(w175) -> ("status"=w180:bool, "code"=w181:i32, "source"=w182:string)
                  n84 = Bundle("Raw data file in"=w178, "refnum out"=w174, "status"=w180, "code"=w181, "source"=w182) -> (w179:T13)  [unwired: 1 in]
                  n85 = Divide(x=w140, y=w138) -> (x/y=w139:dbl)
                  n86 = Round Toward -Infinity(1:w139) -> (0:→"# of traces":dbl)
                  n87 = Bundle(w161, w160) -> (w158:cluster{string[], bool[]})  [unwired: 1 in]
                }
                frame 1 {
                  n88 = Bundle(w276, w277, w278, w275, w274) -> (w273:T14)  [unwired: 1 in]
                  n89 = Unbundle(w273) -> (w268:dbl[][], w271:dbl[], w272:cluster{string[], bool[]}, w270:dbl[][], w269:cluster{dbl, string}[])
                }
              }
              n90 = Unbundle(w110) -> (w109:bool[])  [unwired: 1 out]
              n91 = Index Array(array=w117, index=0) -> (element=→"Scan distance, µm":dbl)
              n92 = Index Array(array=w117, index=1) -> (element=→"Scan angle, degrees":dbl)
              n93 = Index Array(array=w117, index=2) -> (element=→"Record period (single track), s s):":dbl)
              n94 = Index Array(array=w109, index=2) -> (element=→"SISE 1 channel":bool)
              n95 = Index Array(array=w102, index (col)=0 ("disabled index (col)")) -> (element=w130:dbl[])  [unwired: 1 in]
              n96 = Index Array(array=w109, index=3) -> (element=→"SISE 2 channel":bool)
              n97 = Index Array(array=w109, index=4) -> (element=→"Voltage 1 channel":bool)
              n98 = Index Array(array=w109, index=5) -> (element=→"Voltage 2 channel":bool)
              n99 = Add Array Elements(numeric array=w130) -> (sum=w129:dbl)
              n100 = Not Equal To 0?(x=w129) -> (x != 0?=→"Load data":bool)
            }
            frame "Scroll data" {
              n101 = Index Array(array=w288, index (col)=0 ("Deaktivierter Index (Spalte)")) -> (element=w298:dbl[])  [unwired: 1 in]
              n102 = Index Array(array=w283, index=0 ("Index")) -> (element=w285:i32)
              n103 = local read "Trace length"() -> (w315:dbl)
              n104 = Array Size(array=w298) -> (size(s)=w297:i32)
              n105 = local read "# of traces"() -> (w305:dbl)
              n106 = Greater Than 0?(x=w297) -> (x > 0?=w296:bool)
              n107 = local read "# of traces"() -> (w289:dbl)
              n108 = Subtract(x=w289, y=2.0) -> (x-y=w293:dbl)
              n109 = Greater Or Equal?(x=w285, y=1) -> (x >= y?=w292:bool)
              n110 = Less Or Equal?(x=w285, y=w293) -> (x <= y?=w291:bool)
              n111 = Unbundle(w279) -> (w295:bool[])  [unwired: 1 out]
              n112 = Index Array(array=w288, index (col)=0 ("Deaktivierter Index (Spalte)")) -> (element=w320:dbl[])  [unwired: 1 in]
              n113 = And(x=w292, y=w291) -> (x .and. y?=w290:bool)
              n114 = for {
                shift-right: [w837] -> w309
                shift-left: bool[] [] -> [w836]
                tunnel: w295 -> [w835] mode=indexing
                n115 = Insert Into Array(array=w836, new element=w835) -> (w837:bool[])  [unwired: 1 in]
              }
              n116 = Array Size(array=w320) -> (size(s)=w303:i32)
              n117 = Multiply(x=w315, y=w285) -> (x*y=w316:dbl)
              n118 = Array Subset(array=w300, index (row)=w316, length (row)=w315) -> (w311:dbl[][])  [unwired: 2 in]
              n119 = case shown="True" w290 {
                tunnel: w300 -> [_ w662]
                tunnel: w285 -> [_ w663]
                tunnel: w307 -> [_ w703]
                tunnel: w288 -> [w643 w667]
                tunnel: [w643 w677] -> w306
                tunnel: w279 -> [w642 w655]
                tunnel: [w642 w651] -> w287
                frame False {
                }
                frame True {
                  w689 = 2 ("Index")
                  # "Put data to correct column"
                  # "Set SISE1 or SISE1/2 channels to true"
                  # "Exchange time values"
                  # "Calculate average value"
                  # "Select three traces"
                  n120 = local read "Trace length"() -> (w674:dbl)
                  n121 = Unbundle(w655) -> (w661:bool[])  [unwired: 1 out]
                  n122 = Index Array(array=w703, index=2 ("Index")) -> (element=w690:dbl)
                  n123 = Index Array(array=w661, index=3 ("Index")) -> (element=w660:bool)
                  n124 = case shown="True" w660 {
                    tunnel: [1 2] -> w672
                    frame False {
                    }
                    frame True {
                    }
                  }
                  n125 = Subtract(x=w663, y=1) -> (x-y=w713:i32)
                  n126 = Multiply(x=w713, y=w674) -> (x*y=w712:dbl)
                  n127 = Multiply(x=w674, y=3) -> (x*y=w710:dbl)
                  n128 = Array Subset(array=w662, index (row)=w712, length (row)=w710) -> (w669:dbl[][])  [unwired: 2 in]
                  n129 = local read "Start fit (% of rec. period)"() -> (w694:dbl)
                  n130 = local read "Start fit (% of rec. period)"() -> (w701:dbl)
                  n131 = Build Array(0.0 ("Element"), 0.0 ("Element")) -> (w664:dbl[])
                  n132 = Multiply(x=w690, y=w694) -> (x*y=w692:dbl)
                  n133 = Multiply(x=w690, y=100.0) -> (x*y=w691:dbl)
                  n134 = Multiply(x=w690, y=w701) -> (x*y=w708:dbl)
                  n135 = Multiply(x=w690, y=100.0) -> (x*y=w707:dbl)
                  n136 = Add(x=w708, y=w707) -> (x+y=w709:dbl)
                  n137 = Subtract(x=w707, y=w708) -> (x-y=w705:dbl)
                  n138 = Array Subset(array=w669, index (row)=w709, length (row)=w705) -> (w704:dbl[][])  [unwired: 2 in]
                  n139 = Transpose 2D Array(2D array=w704) -> (transposed array=w649:dbl[][])
                  n140 = for {
                    tunnel: w649 -> [w832] mode=indexing
                    shift-right: [w831] -> w659
                    shift-left: dbl[] [] -> [w830]
                    n141 = Add Array Elements(numeric array=w832) -> (sum=w833:dbl)
                    n142 = Array Size(array=w832) -> (size(s)=w834:i32)
                    n143 = Divide(x=w833, y=w834) -> (x/y=w829:dbl)
                    n144 = Insert Into Array(array=w830, new element=w829) -> (w831:dbl[])  [unwired: 1 in]
                  }
                  n145 = Index Array(array=w669, index (col)=0 ("Deaktivierter Index (Spalte)")) -> (element=w697:dbl[])  [unwired: 1 in]
                  n146 = Index Array(array=w659, index=0 ("Index (Spalte)")) -> (element=w695:dbl)
                  n147 = for {
                    tunnel: w695 -> [w825]
                    shift-right: [w828] -> w686
                    shift-left: dbl[] [] -> [w827]
                    tunnel: w697 -> [w824] mode=indexing
                    n148 = Subtract(x=w824, y=w825) -> (x-y=w826:dbl)
                    n149 = Insert Into Array(array=w827, new element=w826) -> (w828:dbl[])  [unwired: 1 in]
                  }
                  n150 = Array Subset(array=w669, index (col)=w689, length (col)=w689) -> (w688:dbl[][])  [unwired: 2 in]
                  n151 = Insert Into Array(array=w688, index (col)=0 ("Index"), new element=w686) -> (w685:dbl[][])  [unwired: 1 in]
                  n152 = for {
                    N: w672 -> [_]
                    tunnel: w685 -> [w754]
                    tunnel: w691 -> [w753]
                    tunnel: w692 -> [w752]
                    tunnel: w663 -> [w750]
                    shift-right: [w749] -> w668
                    shift-left: w664 -> [w748]
                    i -> [w746]
                    n153 = flat-sequence {
                      tunnel: w754 -> [w765]
                      tunnel: w752 -> [w766]
                      tunnel: w753 -> [w773]
                      tunnel: [w770] -> w756
                      tunnel: [w767] -> w755
                      tunnel: w746 -> [w760]
                      tunnel: w756 -> [w797]
                      tunnel: w755 -> [w803]
                      tunnel: w750 -> [w798]
                      tunnel: [w786] -> w747
                      tunnel: [w785] -> w751
                      frame #0 {
                        n154 = Subtract(x=w773, y=w766) -> (x-y=w779:dbl)
                        n155 = Multiply(x=w773, y=2.0) -> (x*y=w776:dbl)
                        n156 = Add(x=w766, y=w776) -> (x+y=w784:dbl)
                        n157 = Add(x=w766, y=w773) -> (x+y=w783:dbl)
                        n158 = Array Subset(array=w765, index (row)=w766, length (row)=w779) -> (w781:dbl[][])  [unwired: 2 in]
                        n159 = Array Subset(array=w765, index (row)=w784, length (row)=w779) -> (w782:dbl[][])  [unwired: 2 in]
                        n160 = Array Subset(array=w765, index (row)=w783, length (row)=w779) -> (w774:dbl[][])  [unwired: 2 in]
                        n161 = Insert Into Array(array=w781, new element=w782) -> (w777:dbl[][])  [unwired: 2 in]
                        n162 = Add(x=w760, y=1) -> (x+y=w761:i32)
                        n163 = Index Array(array=w774, index (col)=w761) -> (element=w764:dbl[])  [unwired: 1 in]
                        n164 = Index Array(array=w777, index (col)=0 ("disabled index (col)")) -> (element=w772:dbl[])  [unwired: 1 in]
                        n165 = Index Array(array=w774, index (col)=0 ("disabled index (col)")) -> (element=w763:dbl[])  [unwired: 1 in]
                        n166 = Index Array(array=w777, index (col)=w761) -> (element=w771:dbl[])  [unwired: 1 in]
                        n167 = call <vilib>:"Linear Fit.vi"("Y"=w771, "X"=w772) -> ("Best Linear Fit"=w762:dbl[], "slope"=w769:dbl, "intercept"=w768:dbl)  [unwired: 9 in, 2 out]
                        n168 = Build Array(w769, w768) -> (w767:dbl[])
                        n169 = Bundle(w772, w771, "Best Linear Fit"=w762, w763, w764) -> (w770:T15)  [unwired: 1 in]
                      }
                      frame #1 {
                        n170 = Unbundle(w797) -> (w808:dbl[], w809:dbl[])  [unwired: 3 out]
                        n171 = Divide(x=w798, y=2 ("x")) -> (x/y=w799:dbl)
                        n172 = Index Array(array=w803, index=0 ("Index")) -> (element=w810:dbl)
                        n173 = Index Array(array=w803, index=1 ("Index")) -> (element=w802:dbl)
                        n174 = Unbundle(w797) -> (w794:dbl[], w796:dbl[], "Best Linear Fit"=w793:dbl[], w792:dbl[], w790:dbl[])
                        n175 = Round To Nearest(number=w799) -> (nearest integer value=w800:dbl)
                        n176 = Absolute Value(x=w810) -> (abs(x)=w815:dbl)
                        n177 = Equal?(x=w800, y=w799) -> (x = y?=w805:bool)
                        n178 = Divide(x=w815, y=1000.0) -> (x/y=w817:dbl)
                        n179 = Bundle(w794, w796) -> (w795:cluster{dbl[], dbl[]})  [unwired: 1 in]
                        n180 = Bundle(w794, "Best Linear Fit"=w793) -> (w789:cluster{dbl[], "Best Linear Fit":dbl[]})  [unwired: 1 in]
                        n181 = Bundle(w792, w790) -> (w787:cluster{dbl[], dbl[]})  [unwired: 1 in]
                        n182 = Subtract(x=w810, y=w817) -> (x-y=w814:dbl)
                        n183 = Add(x=w810, y=w817) -> (x+y=w813:dbl)
                        n184 = Bundle(w814, w813, -inf, inf) -> (w812:cluster{dbl, dbl, dbl, dbl})  [unwired: 1 in]
                        n185 = call <vilib>:"Linear Fit.vi"("Y"=w809, "X"=w808, "parameter bounds"=w812) -> ("Best Linear Fit"=w791:dbl[], "intercept"=w801:dbl)  [unwired: 8 in, 3 out]
                        n186 = Subtract(x=w802, y=w801) -> (x-y=w806:dbl)
                        n187 = Bundle(w792, "Best Linear Fit"=w791) -> (w788:cluster{dbl[], "Best Linear Fit":dbl[]})  [unwired: 1 in]
                        n188 = case shown="False" w805 {
                          tunnel: w806 -> [w821 w823]
                          tunnel: [w822 w823] -> w786
                          frame False {
                            n189 = Multiply(x=-1.0, y=w821) -> (x*y=w822:dbl)
                          }
                          frame True {
                          }
                        }
                        n190 = Build Array(w795, w789, w788, w787) -> (w785:cluster{dbl[], "Best Linear Fit":dbl[]}[])
                      }
                    }
                    n191 = case shown="0, Default" w746 {
                      tunnel: w751 -> [w757 w758 _]
                      frame 0, Default {
                        "deltaV SISE 1" <- w757
                      }
                      frame 1 {
                        "deltaV SISE 2" <- w758
                      }
                      frame 2 {
                      }
                    }
                    n192 = Replace Array Subset(array=w748, new element=w747, index=w746) -> (w749:dbl[])
                  }
                  n193 = Index Array(array=w659, index=0 ("Index")) -> (element=w681:dbl)
                  n194 = Divide(x=w681, y=60.0) -> (x/y=w670:dbl)
                  n195 = Replace Array Subset(array=w659, new element=w670, index=0 ("Index")) -> (w647:dbl[])
                  n196 = Unbundle(w655) -> (w652:string[], w648:bool[])
                  n197 = Index Array(array=w648, index=3 ("Index")) -> (element=w656:bool)
                  n198 = case shown="False" w656 {
                    tunnel: [w730 w733] -> w653
                    frame False {
                      n199 = Build Array(TRUE, FALSE) -> (w730:bool[])
                    }
                    frame True {
                      n200 = Build Array(TRUE, TRUE) -> (w733:bool[])
                    }
                  }
                  n201 = for {
                    tunnel: w648 -> [w723] mode=indexing
                    tunnel: w647 -> [w722]
                    shift-right: [w721] -> _
                    shift-left: 0 -> [w720]
                    shift-right: [w718] -> w644
                    shift-left: dbl[] [] -> [w717]
                    i -> [w715]
                    n202 = Index Array(array=w722, index=w720) -> (element=w719:dbl)
                    n203 = case shown="True" w723 {
                      tunnel: w720 -> [w725 w729]
                      tunnel: [w725 w727] -> w721
                      tunnel: w719 -> [_ w726]
                      tunnel: [0.0 w726] -> w716
                      frame False {
                      }
                      frame True {
                        n204 = Add(x=w729, y=1) -> (x+y=w727:i32)
                      }
                    }
                    n205 = Insert Into Array(array=w717, index=w715, new element=w716) -> (w718:dbl[])
                  }
                  n206 = Subtract(x=w663, y=1) -> (x-y=w675:i32)
                  n207 = Index Array(array=w667, index (row)=w675) -> (element=w680:dbl[])  [unwired: 1 in]
                  n208 = Replace Array Subset(array=w648, new element=w653, index=6 ("Index")) -> (w650:bool[])
                  n209 = Array Size(array=w680) -> (size(s)=w679:i32)
                  n210 = Bundle(w652, w650) -> (w651:cluster{string[], bool[]})  [unwired: 1 in]
                  n211 = Equal To 0?(x=w679) -> (x = 0?=w678:bool)
                  n212 = Insert Into Array(array=w644, index=6 ("Index"), new element=w668) -> (w658:dbl[])
                  n213 = case shown="True" w678 {
                    tunnel: w667 -> [w741 w745]
                    tunnel: [w738 w744] -> w677
                    tunnel: w658 -> [w740 w742]
                    tunnel: w675 -> [w739 w743]
                    frame False {
                      n214 = Replace Array Subset(array=w741, new element=w740, index (row)=w739) -> (w738:dbl[][])  [unwired: 1 in]
                    }
                    frame True {
                      n215 = Insert Into Array(array=w745, index (row)=w743, new element=w742) -> (w744:dbl[][])  [unwired: 1 in]
                    }
                  }
                }
              }
              n216 = case shown="True" w296 {
                tunnel: w279 -> [_ w334]
                tunnel: w288 -> [_ w337]
                tunnel: w301 -> [_ w340]
                tunnel: w300 -> [_ w336]
                tunnel: w285 -> [_ w335]
                frame False {
                }
                frame True {
                  n217 = local read "Trace length"() -> (w380:dbl)
                  n218 = Unbundle(w334) -> (w333:bool[])  [unwired: 1 out]
                  n219 = Add(x=w335, y=1) -> (x+y=w377:i32)
                  n220 = Multiply(x=w380, y=w335) -> (x*y=w378:dbl)
                  n221 = Multiply(x=w380, y=w377) -> (x*y=w379:dbl)
                  n222 = Multiply(x="Zoom from end", y=-1.0) -> (x*y=w358:dbl)
                  n223 = Concatenate Strings("Time, Event mark", "\r\n") -> (w375:string)
                  n224 = Index Array(array=w336, index (row)=w378, index (col)=0 ("Deaktivierter Index (Spalte)")) -> (element=w373:dbl)
                  n225 = Index Array(array=w336, index (row)=w379, index (col)=0 ("Deaktivierter Index (Spalte)")) -> (element=w374:dbl)
                  n226 = Add(x="Zoom from start", y=w358) -> (x+y=w351:dbl)
                  n227 = feedback #1() -> (w354:dbl)  [unwired: 1 in]
                  n228 = Greater Or Equal?(x=w351, y=0.0) -> (x >= y?=w352:bool)
                  n229 = case shown="True" w352 {
                    tunnel: "Zoom from start" -> [w383 w386]
                    tunnel: [w382 w386] -> w338
                    tunnel: w354 -> [w382 w388]
                    tunnel: "Zoom from end" -> [_ w385]
                    tunnel: [w383 w386] -> w359
                    tunnel: [w381 w384] -> w360
                    tunnel: "Zoom from end" -> [w381 w384]
                    frame False {
                    }
                    frame True {
                      n230 = Not Equal?(x=w388, y=w386) -> (x != y?=w387:bool)
                      n231 = case shown="False" w387 {
                        tunnel: w386 -> [_ w390]
                        tunnel: w385 -> [w389 _]
                        frame False {
                          n232 = local write "Zoom from start"(w389) -> ()
                        }
                        frame True {
                          n233 = local write "Zoom from end"(w390) -> ()
                        }
                      }
                    }
                  }
                  n234 = feedback-in #1(w338) -> ()
                  n235 = for {
                    tunnel: w340 -> [w632] mode=indexing
                    shift-right: [w634] -> w339
                    shift-left: dbl[] [] -> [w633]
                    tunnel: w373 -> [w631]
                    tunnel: w374 -> [w630]
                    shift-right: [w624] -> w376
                    shift-left: w375 -> [w627]
                    n236 = Unbundle(w632) -> (w619:dbl, w626:string)
                    n237 = Greater?(x=w619, y=w631) -> (0:w628:bool)
                    n238 = Less Or Equal?(x=w619, y=w630) -> (x <= y?=w629:bool)
                    n239 = And(x=w628, y=w629) -> (x .and. y?=w625:bool)
                    n240 = Divide(x=w619, y=60.0) -> (x/y=w620:dbl)
                    n241 = Number To Fractional String(number=w620, precision (6)=i16 2 ("Genauigkeit (6)")) -> (F-format string=w622:string)  [unwired: 2 in]
                    n242 = case shown="True" w625 {
                      tunnel: w627 -> [w635 w638]
                      tunnel: w626 -> [_ w641]
                      tunnel: [w635 w639] -> w624
                      tunnel: w622 -> [_ w636]
                      frame False {
                      }
                      frame True {
                        n243 = call <vilib>:"Space Constant.vi"() -> ("String"=w637:string)
                        n244 = Concatenate Strings(w638, w636, w637, w641, "\r\n") -> (w639:string)
                      }
                    }
                    n245 = Insert Into Array(array=w633, new element=w620) -> (w634:dbl[])  [unwired: 1 in]
                  }
                  "Event marks" <- w376
                  n246 = Subtract(x=w360, y=w359) -> (x-y=w355:dbl)
                  n247 = Index Array(array=w337, index (col)=0 ("Deaktivierter Index (Spalte)")) -> (element=w350:dbl[])  [unwired: 1 in]
                  n248 = Divide(x=w359, y=100.0) -> (x/y=w357:dbl)
                  n249 = Divide(x=w355, y=100.0) -> (x/y=w356:dbl)
                  n250 = Array Size(array=w350) -> (size(s)=w362:i32)
                  n251 = Multiply(x=w362, y=w357) -> (x*y=w365:dbl)
                  n252 = Multiply(x=w362, y=w356) -> (x*y=w363:dbl)
                  n253 = Add(x=w363, y=2.0) -> (x+y=w364:dbl)
                  n254 = Subtract(x=w365, y=2.0) -> (x-y=w366:dbl)
                  n255 = Array Subset(array=w337, index (row)=w366, length (row)=w364) -> (w341:dbl[][])  [unwired: 2 in]
                  n256 = Add(x=2, y="TC 3") -> (x+y=w332:u32)
                  n257 = Index Array(array=w333, index=w332) -> (element=w342:bool)
                  n258 = case shown="\"V channel #1\"" "TC 3" {
                    tunnel: w341 -> [w394 w470 w578 w585]
                    tunnel: w339 -> [w392 w469 w546 w588]
                    tunnel: w342 -> [w391 w468 w545 w582]
                    frame "SISE channel #1", Default {
                      n259 = Index Array(array=w394, index (col)=0 ("disabled index (col)")) -> (element=w397:dbl[])  [unwired: 1 in]
                      n260 = Index Array(array=w394, index (col)=2 ("disabled index (col)")) -> (element=w396:dbl[])  [unwired: 1 in]
                      n261 = Index Array(array=w394, index (col)=6 ("disabled index (col)")) -> (element=w393:dbl[])  [unwired: 1 in]
                      n262 = stacked-sequence {
                        tunnel: w397 -> [w401 w440]
                        tunnel: w396 -> [w420 _]
                        tunnel: w392 -> [w402 w434]
                        tunnel: w393 -> [_ w439]
                        tunnel: w391 -> [w400 w435]
                        frame #0 {
                          n263 = Array Max & Min(array=w401) -> (max value=w412:dbl, min value=w411:dbl)  [unwired: 2 out]
                          n264 = Divide(x="Range limit\nS1.1 (mV)", y=2.0) -> (x/y=w430:dbl)
                          n265 = Divide(x="Range limit\nS1.1 (mV)", y=2.05) -> (x/y=w431:dbl)
                          n266 = Add(x="Base line\nS1.1 (mV)", y=w430) -> (x+y=w403:dbl)
                          n267 = Subtract(x="Base line\nS1.1 (mV)", y=w430) -> (x-y=w404:dbl)
                          n268 = Subtract(x="Base line\nS1.1 (mV)", y=w431) -> (x-y=w410:dbl)
                          n269 = call "EventstoGraph (SubVI).vi"("Numerisch 2"=w411, "Array 3"=w402, "Numerisch"=w412, "Array (Eingang)"=dbl[][] [], "Numerisch 3"=w410) -> ("Array (Ausgang)"=w414:dbl[][])  [unwired: 6 in]
                          n270 = Array Max & Min(array=w401) -> (max value=w426:dbl, min value=w427:dbl)  [unwired: 2 out]
                          n271 = call "GraphLimit01.vi"("Numeric 2"=w404, "Numeric"=w403, "Array in"=w420, "Array 3"=dbl[] []) -> ("Array out"=w419:dbl[])  [unwired: 7 in]
                          n272 = Build Array("Base line\nS1.1 (mV)", "Base line\nS1.1 (mV)") -> (w423:dbl[])
                          n273 = Build Array(w426, w427) -> (w424:dbl[])
                          n274 = Build Array(w403, w404) -> (w425:dbl[])
                          n275 = Index Array(array=w414, index (col)=0 ("Index (Zeile)")) -> (element=w415:dbl[])  [unwired: 1 in]
                          n276 = Index Array(array=w414, index (col)=1 ("Index (Zeile)")) -> (element=w413:dbl[])  [unwired: 1 in]
                          n277 = Bundle(w424, w425) -> (w407:cluster{dbl[], dbl[]})  [unwired: 1 in]
                          n278 = Bundle(w424, w423) -> (w408:cluster{dbl[], dbl[]})  [unwired: 1 in]
                          n279 = Bundle(w401, "Array out"=w419) -> (w406:cluster{dbl[], "Array out":dbl[]})  [unwired: 1 in]
                          n280 = Bundle("Array (Ausgang)"=w415, "Array (Ausgang)"=w413) -> (w405:T16)  [unwired: 1 in]
                          n281 = Build Array(w408, w407, w406, w405) -> (w409:T17)
                          n282 = case shown="True" w400 {
                            tunnel: w409 -> [_ w433]
                            frame False {
                            }
                            frame True {
                              "V-SISE channel 1" <- w433
                            }
                          }
                        }
                        frame #1 {
                          n283 = Array Max & Min(array=w440) -> (max value=w449:dbl, min value=w448:dbl)  [unwired: 2 out]
                          n284 = Divide(x="Range limit\nS1.2 mV", y=2.0) -> (x/y=w465:dbl)
                          n285 = Divide(x="Range limit\nS1.2 mV", y=2.05) -> (x/y=w466:dbl)
                          n286 = Add(x="Base line \nS1.2 (mV)", y=w465) -> (x+y=w441:dbl)
                          n287 = Subtract(x="Base line \nS1.2 (mV)", y=w465) -> (x-y=w442:dbl)
                          n288 = Subtract(x="Base line \nS1.2 (mV)", y=w466) -> (x-y=w447:dbl)
                          n289 = call "EventstoGraph (SubVI).vi"("Numerisch 2"=w448, "Array 3"=w434, "Numerisch"=w449, "Array (Eingang)"=dbl[][] [], "Numerisch 3"=w447) -> ("Array (Ausgang)"=w451:dbl[][])  [unwired: 6 in]
                          n290 = Array Max & Min(array=w440) -> (max value=w461:dbl, min value=w462:dbl)  [unwired: 2 out]
                          n291 = call "GraphLimit01.vi"("Numeric 2"=w442, "Numeric"=w441, "Array in"=w439, "Array 3"=dbl[] []) -> ("Array out"=w456:dbl[])  [unwired: 7 in]
                          n292 = Build Array("Base line \nS1.2 (mV)", "Base line \nS1.2 (mV)") -> (w458:dbl[])
                          n293 = Build Array(w461, w462) -> (w459:dbl[])
                          n294 = Build Array(w441, w442) -> (w460:dbl[])
                          n295 = Index Array(array=w451, index (col)=0 ("Index (Zeile)")) -> (element=w452:dbl[])  [unwired: 1 in]
                          n296 = Index Array(array=w451, index (col)=1 ("Index (Zeile)")) -> (element=w450:dbl[])  [unwired: 1 in]
                          n297 = Bundle(w459, w460) -> (w445:cluster{dbl[], dbl[]})  [unwired: 1 in]
                          n298 = Bundle(w459, w458) -> (w446:cluster{dbl[], dbl[]})  [unwired: 1 in]
                          n299 = Bundle(w440, "Array out"=w456) -> (w444:cluster{dbl[], "Array out":dbl[]})  [unwired: 1 in]
                          n300 = Bundle("Array (Ausgang)"=w452, "Array (Ausgang)"=w450) -> (w443:T16)  [unwired: 1 in]
                          n301 = Build Array(w446, w445, w444, w443) -> (w436:T17)
                          n302 = case shown="True" w435 {
                            tunnel: w436 -> [_ w467]
                            frame False {
                            }
                            frame True {
                              "dV-SISE channel 1" <- w467
                            }
                          }
                        }
                      }
                    }
                    frame "SISE channel #2" {
                      n303 = Index Array(array=w470, index (col)=0 ("disabled index (col)")) -> (element=w474:dbl[])  [unwired: 1 in]
                      n304 = Index Array(array=w470, index (col)=3 ("disabled index (col)")) -> (element=w475:dbl[])  [unwired: 1 in]
                      n305 = Index Array(array=w470, index (col)=7 ("disabled index (col)")) -> (element=w476:dbl[])  [unwired: 1 in]
                      n306 = stacked-sequence {
                        tunnel: w474 -> [w478 w517]
                        tunnel: w475 -> [w497 _]
                        tunnel: w469 -> [w479 w516]
                        tunnel: w476 -> [_ w515]
                        tunnel: w468 -> [w477 w511]
                        frame #0 {
                          n307 = Array Max & Min(array=w478) -> (max value=w489:dbl, min value=w488:dbl)  [unwired: 2 out]
                          n308 = Divide(x="Range limit\nS2.1 (mV)", y=2.0) -> (x/y=w507:dbl)
                          n309 = Divide(x="Range limit\nS2.1 (mV)", y=2.05) -> (x/y=w508:dbl)
                          n310 = Add(x="Base line\nS2.1 (mV)", y=w507) -> (x+y=w480:dbl)
                          n311 = Subtract(x="Base line\nS2.1 (mV)", y=w507) -> (x-y=w481:dbl)
                          n312 = Subtract(x="Base line\nS2.1 (mV)", y=w508) -> (x-y=w487:dbl)
                          n313 = call "EventstoGraph (SubVI).vi"("Numerisch 2"=w488, "Array 3"=w479, "Numerisch"=w489, "Array (Eingang)"=dbl[][] [], "Numerisch 3"=w487) -> ("Array (Ausgang)"=w491:dbl[][])  [unwired: 6 in]
                          n314 = Array Max & Min(array=w478) -> (max value=w503:dbl, min value=w504:dbl)  [unwired: 2 out]
                          n315 = call "GraphLimit01.vi"("Numeric 2"=w481, "Numeric"=w480, "Array in"=w497, "Array 3"=dbl[] []) -> ("Array out"=w496:dbl[])  [unwired: 7 in]
                          n316 = Build Array("Base line\nS2.1 (mV)", "Base line\nS2.1 (mV)") -> (w500:dbl[])
                          n317 = Build Array(w503, w504) -> (w501:dbl[])
                          n318 = Build Array(w480, w481) -> (w502:dbl[])
                          n319 = Index Array(array=w491, index (col)=0 ("Index (Zeile)")) -> (element=w492:dbl[])  [unwired: 1 in]
                          n320 = Index Array(array=w491, index (col)=1 ("Index (Zeile)")) -> (element=w490:dbl[])  [unwired: 1 in]
                          n321 = Bundle(w501, w502) -> (w484:cluster{dbl[], dbl[]})  [unwired: 1 in]
                          n322 = Bundle(w501, w500) -> (w485:cluster{dbl[], dbl[]})  [unwired: 1 in]
                          n323 = Bundle(w478, "Array out"=w496) -> (w483:cluster{dbl[], "Array out":dbl[]})  [unwired: 1 in]
                          n324 = Bundle("Array (Ausgang)"=w492, "Array (Ausgang)"=w490) -> (w482:T16)  [unwired: 1 in]
                          n325 = Build Array(w485, w484, w483, w482) -> (w486:T17)
                          n326 = case shown="True" w477 {
                            tunnel: w486 -> [_ w510]
                            frame False {
                            }
                            frame True {
                              "V-SISE channel 2" <- w510
                            }
                          }
                        }
                        frame #1 {
                          n327 = Array Max & Min(array=w517) -> (max value=w526:dbl, min value=w525:dbl)  [unwired: 2 out]
                          n328 = Divide(x="Range limit\nS2.2 (mV)", y=2.0) -> (x/y=w542:dbl)
                          n329 = Divide(x="Range limit\nS2.2 (mV)", y=2.05) -> (x/y=w543:dbl)
                          n330 = Add(x="Base line \nS2.2 (mV)", y=w542) -> (x+y=w518:dbl)
                          n331 = Subtract(x="Base line \nS2.2 (mV)", y=w542) -> (x-y=w519:dbl)
                          n332 = Subtract(x="Base line \nS2.2 (mV)", y=w543) -> (x-y=w524:dbl)
                          n333 = call "EventstoGraph (SubVI).vi"("Numerisch 2"=w525, "Array 3"=w516, "Numerisch"=w526, "Array (Eingang)"=dbl[][] [], "Numerisch 3"=w524) -> ("Array (Ausgang)"=w528:dbl[][])  [unwired: 6 in]
                          n334 = Array Max & Min(array=w517) -> (max value=w538:dbl, min value=w539:dbl)  [unwired: 2 out]
                          n335 = call "GraphLimit01.vi"("Numeric 2"=w519, "Numeric"=w518, "Array in"=w515, "Array 3"=dbl[] []) -> ("Array out"=w533:dbl[])  [unwired: 7 in]
                          n336 = Build Array("Base line \nS2.2 (mV)", "Base line \nS2.2 (mV)") -> (w535:dbl[])
                          n337 = Build Array(w538, w539) -> (w536:dbl[])
                          n338 = Build Array(w518, w519) -> (w537:dbl[])
                          n339 = Index Array(array=w528, index (col)=0 ("Index (Zeile)")) -> (element=w529:dbl[])  [unwired: 1 in]
                          n340 = Index Array(array=w528, index (col)=1 ("Index (Zeile)")) -> (element=w527:dbl[])  [unwired: 1 in]
                          n341 = Bundle(w536, w537) -> (w522:cluster{dbl[], dbl[]})  [unwired: 1 in]
                          n342 = Bundle(w536, w535) -> (w523:cluster{dbl[], dbl[]})  [unwired: 1 in]
                          n343 = Bundle(w517, "Array out"=w533) -> (w521:cluster{dbl[], "Array out":dbl[]})  [unwired: 1 in]
                          n344 = Bundle("Array (Ausgang)"=w529, "Array (Ausgang)"=w527) -> (w520:T16)  [unwired: 1 in]
                          n345 = Build Array(w523, w522, w521, w520) -> (w512:T17)
                          n346 = case shown="True" w511 {
                            tunnel: w512 -> [_ w544]
                            frame False {
                            }
                            frame True {
                              "dV-SISE channel 2" <- w544
                            }
                          }
                        }
                      }
                    }
                    frame "V channel #1" {
                      n347 = Index Array(array=w578, index (col)=0 ("disabled index (col)")) -> (element=w547:dbl[])  [unwired: 1 in]
                      n348 = Index Array(array=w578, index (col)=4 ("disabled index (col)")) -> (element=w548:dbl[])  [unwired: 1 in]
                      n349 = Array Max & Min(array=w547) -> (max value=w558:dbl, min value=w557:dbl)  [unwired: 2 out]
                      n350 = Divide(x="Range limit\nV1 (V)", y=2.0) -> (x/y=w575:dbl)
                      n351 = Divide(x="Range limit\nV1 (V)", y=2.05) -> (x/y=w576:dbl)
                      n352 = Add(x="Base line\nV1 (V)", y=w575) -> (x+y=w549:dbl)
                      n353 = Subtract(x="Base line\nV1 (V)", y=w575) -> (x-y=w550:dbl)
                      n354 = Subtract(x="Base line\nV1 (V)", y=w576) -> (x-y=w556:dbl)
                      n355 = call "EventstoGraph (SubVI).vi"("Numerisch 2"=w557, "Array 3"=w546, "Numerisch"=w558, "Array (Eingang)"=dbl[][] [], "Numerisch 3"=w556) -> ("Array (Ausgang)"=w560:dbl[][])  [unwired: 6 in]
                      n356 = Array Max & Min(array=w547) -> (max value=w571:dbl, min value=w572:dbl)  [unwired: 2 out]
                      n357 = call "GraphLimit01.vi"("Numeric 2"=w550, "Numeric"=w549, "Array in"=w548, "Array 3"=dbl[] []) -> ("Array out"=w565:dbl[])  [unwired: 7 in]
                      n358 = Build Array("Base line\nV1 (V)", "Base line\nV1 (V)") -> (w568:dbl[])
                      n359 = Build Array(w571, w572) -> (w569:dbl[])
                      n360 = Build Array(w549, w550) -> (w570:dbl[])
                      n361 = Index Array(array=w560, index (col)=0 ("Index (Zeile)")) -> (element=w561:dbl[])  [unwired: 1 in]
                      n362 = Index Array(array=w560, index (col)=1 ("Index (Zeile)")) -> (element=w559:dbl[])  [unwired: 1 in]
                      n363 = Bundle(w569, w570) -> (w553:cluster{dbl[], dbl[]})  [unwired: 1 in]
                      n364 = Bundle(w569, w568) -> (w554:cluster{dbl[], dbl[]})  [unwired: 1 in]
                      n365 = Bundle(w547, "Array out"=w565) -> (w552:cluster{dbl[], "Array out":dbl[]})  [unwired: 1 in]
                      n366 = Bundle("Array (Ausgang)"=w561, "Array (Ausgang)"=w559) -> (w551:T16)  [unwired: 1 in]
                      n367 = Build Array(w554, w553, w552, w551) -> (w555:T17)
                      n368 = case shown="True" w545 {
                        tunnel: w555 -> [_ w581]
                        frame False {
                        }
                        frame True {
                          "Voltage channel 1" <- w581
                        }
                      }
                    }
                    frame "V channel #2" {
                      n369 = Index Array(array=w585, index (col)=0 ("disabled index (col)")) -> (element=w583:dbl[])  [unwired: 1 in]
                      n370 = Index Array(array=w585, index (col)=5 ("disabled index (col)")) -> (element=w584:dbl[])  [unwired: 1 in]
                      n371 = Array Max & Min(array=w583) -> (max value=w598:dbl, min value=w597:dbl)  [unwired: 2 out]
                      n372 = Divide(x="Range limit\nV2 (V)", y=2.0) -> (x/y=w615:dbl)
                      n373 = Divide(x="Range limit\nV2 (V)", y=2.05) -> (x/y=w616:dbl)
                      n374 = Add(x="Base line\nV2 (V)", y=w615) -> (x+y=w589:dbl)
                      n375 = Subtract(x="Base line\nV2 (V)", y=w615) -> (x-y=w590:dbl)
                      n376 = Subtract(x="Base line\nV2 (V)", y=w616) -> (x-y=w596:dbl)
                      n377 = call "EventstoGraph (SubVI).vi"("Numerisch 2"=w597, "Array 3"=w588, "Numerisch"=w598, "Array (Eingang)"=dbl[][] [], "Numerisch 3"=w596) -> ("Array (Ausgang)"=w600:dbl[][])  [unwired: 6 in]
                      n378 = Array Max & Min(array=w583) -> (max value=w611:dbl, min value=w612:dbl)  [unwired: 2 out]
                      n379 = call "GraphLimit01.vi"("Numeric 2"=w590, "Numeric"=w589, "Array in"=w584, "Array 3"=dbl[] []) -> ("Array out"=w605:dbl[])  [unwired: 7 in]
                      n380 = Build Array("Base line\nV2 (V)", "Base line\nV2 (V)") -> (w608:dbl[])
                      n381 = Build Array(w611, w612) -> (w609:dbl[])
                      n382 = Build Array(w589, w590) -> (w610:dbl[])
                      n383 = Index Array(array=w600, index (col)=0 ("Index (Zeile)")) -> (element=w601:dbl[])  [unwired: 1 in]
                      n384 = Index Array(array=w600, index (col)=1 ("Index (Zeile)")) -> (element=w599:dbl[])  [unwired: 1 in]
                      n385 = Bundle(w609, w610) -> (w593:cluster{dbl[], dbl[]})  [unwired: 1 in]
                      n386 = Bundle(w609, w608) -> (w594:cluster{dbl[], dbl[]})  [unwired: 1 in]
                      n387 = Bundle(w583, "Array out"=w605) -> (w592:cluster{dbl[], "Array out":dbl[]})  [unwired: 1 in]
                      n388 = Bundle("Array (Ausgang)"=w601, "Array (Ausgang)"=w599) -> (w591:T16)  [unwired: 1 in]
                      n389 = Build Array(w594, w593, w592, w591) -> (w595:T17)
                      n390 = case shown="True" w582 {
                        tunnel: w595 -> [_ w618]
                        frame False {
                        }
                        frame True {
                          "Voltage channel 2" <- w618
                        }
                      }
                    }
                  }
                }
              }
              n391 = Subtract(x=w305, y=2.0) -> (x-y=w302:dbl)
              n392 = Equal?(x=w302, y=w303) -> (x = y?=→"Scroll data":bool)
              n393 = Or(x="Step forward", y="Step back") -> (x .or. y?=w325:bool)
              n394 = Or(x="Step back", y="Scroll back") -> (x .or. y?=w323:bool)
              n395 = Or(x="Scroll back", y="Scroll forward") -> (x .or. y?=w319:bool)
              n396 = case shown="\"SISE chan #1\", Default" "?" {
                selector: "?" -> [w839 w851 w859 w867]
                tunnel: w307 -> [w846 w853 w863 w870]
                tunnel: w311 -> [w847 w854 w862 w871]
                tunnel: w309 -> [w843 w850 w857 w866]
                tunnel: "Start fit (% of rec. period)" -> [w845 w852 w861 w869]
                frame "SISE chan #1", Default {
                  n397 = Add(x=2, y=w839) -> (x+y=w840:u32)
                  n398 = Index Array(array=w843, index=w840) -> (element=w842:bool)
                  n399 = call "Feed-SISE-Probe-Graph.vi"("Boolesch"=w842, "Numerisch"=2, "Array 2"=w847, "Array"=w846, "Start fit (% of rec. period)"=w845) -> ("Array 3"=→"Vprobe SISE 1":cluster{dbl[], dbl[]}[])  [unwired: 6 in]
                }
                frame "SISE chan #2" {
                  n400 = Index Array(array=w850, index=w851) -> (element=w849:bool)
                  n401 = call "Feed-SISE-Probe-Graph.vi"("Boolesch"=w849, "Numerisch"=3, "Array 2"=w854, "Array"=w853, "Start fit (% of rec. period)"=w852) -> ("Array 3"=→"Vprobe SISE 2":cluster{dbl[], dbl[]}[])  [unwired: 6 in]
                }
                frame "V chan #1" {
                  n402 = Index Array(array=w857, index=w859) -> (element=w858:bool)
                  n403 = call "Feed-V-Probe-Graph.vi"("Boolesch"=w858, "Numerisch"=4, "Array 2"=w862, "Array"=w863, "Start fit (% of rec. period)"=w861) -> ("Array 3"=→"Vprobe V 1":cluster{dbl[], dbl[]}[])  [unwired: 6 in]
                }
                frame "V chan #2" {
                  n404 = Index Array(array=w866, index=w867) -> (element=w865:bool)
                  n405 = call "Feed-V-Probe-Graph.vi"("Boolesch"=w865, "Numerisch"=5, "Array 2"=w871, "Array"=w870, "Start fit (% of rec. period)"=w869) -> ("Array 3"=→"Vprobe V 2":cluster{dbl[], dbl[]}[])  [unwired: 6 in]
                }
              }
              n406 = call "Feed-Position-Graph (SubVI).vi"("Array 2"=w307, "Array"=w311) -> ("Array 3"=→"Position probe":cluster{dbl[], dbl[]}[])  [unwired: 9 in]
              n407 = Or(x=w325, y=w319) -> (x .or. y?=w324:bool)
              n408 = case shown="True" w324 {
                tunnel: [0 w896] -> w322
                tunnel: w323 -> [_ w895]
                frame False {
                }
                frame True {
                  n409 = case shown="True" w895 {
                    tunnel: [1 2] -> w896
                    frame False {
                    }
                    frame True {
                    }
                  }
                }
              }
              n410 = case shown="True" w319 {
                tunnel: [200 w873] -> w318
                frame False {
                }
                frame True {
                  n411 = Divide(x=500.0, y="Scroll speed") -> (x/y=w873:dbl)
                }
              }
              n412 = case shown="2" w322 {
                tunnel: w285 -> [w876 w882 w889]
                tunnel: w305 -> [_ w877 _]
                tunnel: [w876 w881 w888] -> w282
                frame 0, Default {
                }
                frame 1 {
                  n413 = Subtract(x=w877, y=1) -> (x-y=w879:dbl)
                  n414 = Less?(x=w882, y=w879) -> (x < y?=w880:bool)
                  n415 = case shown="False" w880 {
                    tunnel: w882 -> [w883 w886]
                    tunnel: [w883 w884] -> w881
                    frame False {
                    }
                    frame True {
                      n416 = Add(x=w886, y=1) -> (x+y=w884:i32)
                    }
                  }
                }
                frame 2 {
                  n417 = Greater Than 0?(x=w889) -> (x > 0?=w887:bool)
                  n418 = case shown="True" w887 {
                    tunnel: w889 -> [w890 w893]
                    tunnel: [w890 w891] -> w888
                    frame False {
                    }
                    frame True {
                      n419 = Subtract(x=w893, y=1) -> (x-y=w891:i32)
                    }
                  }
                }
              }
              "Trace #" <- w282
              n420 = Wait (ms)(milliseconds to wait=w318) -> ()  [unwired: 1 out]
              n421 = Replace Array Subset(array=w283, new element=w282, index=0 ("Index")) -> (w284:i32[])
            }
          }
          n422 = Equal?(x="Module selection view data", y=u16 0) -> (x = y?=w90:bool)
          n423 = Select(t=T9."Enabled" ("Disabled"), s=w90, f=T9."Disabled and Grayed Out") -> (s? t:f=w87:T9)
          n424 = property on="Load data" class="Bool (strict)"("DisabledEnum"=w87) -> ()  [unwired: 2 in, 2 out]
          n425 = Equal?(x="Module selection view data", y=u16 1) -> (x = y?=w85:bool)
          n426 = Select(t=T9."Enabled" ("Disabled"), s=w85, f=T9."Disabled and Grayed Out") -> (s? t:f=w82:T9)
          n427 = property on="Scroll data" class="Bool (strict)"("DisabledEnum"=w82) -> ()  [unwired: 2 in, 2 out]
          n428 = Replace Array Subset(array=w68, new element=w65, index=0 ("Index")) -> (w66:T12)
        }
        frame "Save analysis" {
          n429 = Index Array(array=w902, index=1 ("Index")) -> (element=w903:T11)
          n430 = case shown="\"New/stop analysis\"" "Module selection Save Data" {
            tunnel: w903 -> [w954 w984 w996]
            tunnel: [w949 w984 w996] -> w901
            tunnel: w933 -> [w944 w988 w1004]
            tunnel: w932 -> [w945 w989 w1003]
            tunnel: w931 -> [w946 w990 w1002]
            tunnel: w930 -> [w947 w987 w1001]
            tunnel: w929 -> [w948 w986 w1000]
            tunnel: [w943 w985 w999] -> w928
            tunnel: [0 2 1] -> w906
            frame "Create analysis file", Default {
              n431 = local read "Raw data file in"() -> (→"Raw data file":path)
              n432 = call <vilib>:"Check if File or Folder Exists.vi"("path"="Analysis output file") -> ("file or folder exists?"=w934:bool, "dup path"=w938:path)  [unwired: 8 in, 1 out]
              n433 = Unbundle(w954) -> (w952:path, "Referenz (Ausgang)"=w940:refnum<file>, w950:bool, w951:i32, w942:string)
              n434 = Bundle(w944, w945, w946, w947, w948) -> (w943:T14)  [unwired: 1 in]
              n435 = Not(x=w934) -> (.not. x?=w935:bool)
              n436 = Bundle(w950, w951, w942) -> (w941:errorcluster)  [unwired: 1 in]
              n437 = Not Equal?(x=w938, y=w952) -> (x != y?=w937:bool)
              n438 = And(x=w935, y=w937) -> (x .and. y?=w936:bool)
              n439 = feedback #2(FALSE) -> (w958:bool)
              n440 = case shown="True" w936 {
                tunnel: w938 -> [_ w969]
                tunnel: [w967 w972] -> w957
                tunnel: w958 -> [w967 _]
                tunnel: [w960 w974] -> w949
                tunnel: [w967 w972] -> w959
                tunnel: w952 -> [w965 _]
                tunnel: w941 -> [w966 w970]
                tunnel: w940 -> [w961 _]
                frame False {
                  n441 = Unbundle(w966) -> (w962:bool, w963:i32, w964:string)
                  n442 = Bundle(w965, "Referenz (Ausgang)"=w961, w962, w963, w964) -> (w960:T11)  [unwired: 1 in]
                }
                frame True {
                  n443 = Open/Create/Replace File(file path (use dialog)=w969, error in=w970, operation (0:open)=T10."create") -> (refnum out=w980:refnum<file>, error out=w979:errorcluster)  [unwired: 3 in, 1 out]
                  n444 = Set File Position(offset (in bytes) (0)=i64 0, refnum=w980, from (0:start)=enum16{"start", "end", "current"}."end", error in=w979) -> (refnum out=w968:refnum<file>, error out=w973:errorcluster)
                  n445 = Unbundle By Name(w973) -> ("status"=w971:bool)
                  n446 = Not(x=w971) -> (.not. x?=w972:bool)
                  n447 = Unbundle(w973) -> ("status"=w977:bool, "code"=w976:i32, "source"=w975:string)
                  n448 = Bundle("dup path"=w969, "refnum"=w968, "status"=w977, "code"=w976, "source"=w975) -> (w974:T18)  [unwired: 1 in]
                }
              }
              "Create analysis file" <- w957
              n449 = feedback-in #2(w959) -> ()
            }
            frame "New/stop analysis" {
              n450 = Bundle(w988, w989, w990, w987, w986) -> (w985:T14)  [unwired: 1 in]
              n451 = local read "Save analyses file"() -> (w983:bool)
              "Next data file/exit program" <- w983
              n452 = case shown="True" w983 {
                frame False {
                }
                frame True {
                  n453 = Or(x="Exit program", y="Next data file") -> (x .or. y?=w994:bool)
                  n454 = case shown="True" w994 {
                    frame False {
                    }
                    frame True {
                      n455 = local write "Main Tab Control"(0) -> ()
                    }
                  }
                }
              }
            }
            frame "Save data" {
              n456 = Unbundle(w1002) -> (w1008:string[], w1010:bool[])
              n457 = for {
                tunnel: "Select output" -> [w1024] mode=indexing
                tunnel: w1010 -> [w1025] mode=indexing
                shift-right: [w1021] -> w1007
                shift-left: bool[] [] -> [w1022]
                n458 = And(x=w1025, y=w1024) -> (x .and. y?=w1023:bool)
                n459 = case shown="True" w1023 {
                  tunnel: w1022 -> [w1027 w1030]
                  tunnel: [w1026 w1031] -> w1021
                  frame False {
                    n460 = Insert Into Array(array=w1027, new element=FALSE) -> (w1026:bool[])  [unwired: 1 in]
                  }
                  frame True {
                    n461 = Insert Into Array(array=w1030, new element=TRUE) -> (w1031:bool[])  [unwired: 1 in]
                  }
                }
              }
              "Indicate output" <- w1007
              n462 = Bundle(w1004, w1003, w1002, w1001, w1000) -> (w999:T14)  [unwired: 1 in]
              n463 = local read "Create analysis file"() -> (w997:bool)
              n464 = And(x=w997, y="Save data") -> (x .and. y?=w1006:bool)
              n465 = case shown="True" w1006 {
                tunnel: w1008 -> [_ w1043]
                tunnel: w1007 -> [_ w1036]
                tunnel: w1001 -> [_ w1040]
                tunnel: w996 -> [_ w1048]
                frame False {
                }
                frame True {
                  n466 = Index Array(array=w1040, index (col)=0 ("Index (Zeile)")) -> (element=w1049:dbl[])  [unwired: 1 in]
                  n467 = for {
                    tunnel: w1036 -> [w1053] mode=indexing
                    shift-right: [w1050] -> w1035
                    shift-left: 0 -> [w1051]
                    i -> [w1052]
                    n468 = case shown="False" w1053 {
                      tunnel: w1052 -> [_ w1055]
                      tunnel: w1051 -> [w1054 _]
                      tunnel: [w1054 w1055] -> w1050
                      frame False {
                      }
                      frame True {
                      }
                    }
                  }
                  n469 = Unbundle(w1048) -> ("Referenz (Ausgang)"=w1044:refnum<file>, w1045:bool, w1046:i32, w1047:string)  [unwired: 1 out]
                  n470 = Array Size(array=w1049) -> (size(s)=w1042:i32)
                  n471 = Bundle(w1045, w1046, w1047) -> (w1034:errorcluster)  [unwired: 1 in]
                  n472 = Add(x=w1042, y=2) -> (x+y=w1038:i32)
                  n473 = for {
                    N: w1038 -> [_]
                    tunnel: w1043 -> [w1065]
                    tunnel: w1044 -> [w1068]
                    tunnel: w1036 -> [w1066]
                    tunnel: w1040 -> [w1064]
                    tunnel: w1035 -> [w1060]
                    tunnel: w1034 -> [w1058]
                    tunnel: [w1057] -> w1033
                    tunnel: [w1056] -> w1032
                    i -> [w1059]
                    n474 = Greater Or Equal?(x=w1059, y=2) -> (x >= y?=w1063:bool)
                    n475 = case shown="True" w1063 {
                      tunnel: [w1069 2] -> w1061
                      tunnel: w1059 -> [w1069 _]
                      frame False {
                      }
                      frame True {
                      }
                    }
                    n476 = case shown="2" w1061 {
                      tunnel: [w1075 w1078 w1099] -> w1067
                      tunnel: w1066 -> [_ w1077 w1101]
                      tunnel: w1065 -> [_ w1080 _]
                      tunnel: w1064 -> [_ _ w1104]
                      tunnel: w1060 -> [_ w1076 w1097]
                      tunnel: w1059 -> [_ _ w1096]
                      frame 0, Default {
                        n477 = local read "Raw data file in"() -> (w1072:path)
                        n478 = Path To String(path=w1072) -> (string=w1074:string)
                        n479 = Concatenate Strings("Datafile in: ", w1074, "\r\n") -> (w1075:string)
                      }
                      frame 1 {
                        n480 = for {
                          tunnel: w1076 -> [w1085]
                          tunnel: w1077 -> [w1088] mode=indexing
                          tunnel: w1080 -> [w1087] mode=indexing
                          shift-right: [w1083] -> w1078
                          shift-left: "" -> [w1082]
                          i -> [w1086]
                          n481 = Equal?(x=w1085, y=w1086) -> (x = y?=w1084:bool)
                          n482 = case shown="False" w1088 {
                            tunnel: w1087 -> [_ w1093]
                            tunnel: w1084 -> [_ w1092]
                            tunnel: ["" w1090] -> w1081
                            frame False {
                            }
                            frame True {
                              n483 = case shown="True" w1092 {
                                tunnel: ["\t" "\r\n"] -> w1091
                                frame False {
                                }
                                frame True {
                                }
                              }
                              n484 = Concatenate Strings(w1093, w1091) -> (w1090:string)
                            }
                          }
                          n485 = Concatenate Strings(w1082, w1081) -> (w1083:string)
                        }
                      }
                      frame 2 {
                        n486 = Subtract(x=w1096, y=2 ("x")) -> (x-y=w1102:i32)
                        n487 = Index Array(array=w1104, index (row)=w1102) -> (element=w1100:dbl[])  [unwired: 1 in]
                        n488 = for {
                          tunnel: w1101 -> [w1112] mode=indexing
                          tunnel: w1100 -> [w1111] mode=indexing
                          shift-right: [w1107] -> w1099
                          shift-left: "" -> [w1106]
                          tunnel: w1097 -> [w1109]
                          i -> [w1108]
                          n489 = Equal?(x=w1109, y=w1108) -> (x = y?=w1110:bool)
                          n490 = case shown="False" w1112 {
                            tunnel: w1111 -> [_ w1118]
                            tunnel: ["" w1119] -> w1105
                            tunnel: w1110 -> [_ w1115]
                            frame False {
                            }
                            frame True {
                              n491 = Number To Exponential String(number=w1118, precision (6)=i16 6 ("Genauigkeit (6)")) -> (E-format string=w1116:string)  [unwired: 2 in]
                              n492 = case shown="False" w1115 {
                                tunnel: ["\t" "\r\n"] -> w1114
                                frame False {
                                }
                                frame True {
                                }
                              }
                              n493 = Concatenate Strings(w1116, w1114) -> (w1119:string)
                            }
                          }
                          n494 = Concatenate Strings(w1106, w1105) -> (w1107:string)
                        }
                      }
                    }
                    n495 = Write to Text File(file (use dialog)=w1068, text=w1067, error in=w1058) -> (refnum out=w1057:refnum<file>, error out=w1056:errorcluster)  [unwired: 1 in, 1 out]
                  }
                  n496 = Close File(refnum=w1033, error in=w1032) -> ()  [unwired: 2 out]
                }
              }
              n497 = case shown="True" w997 {
                tunnel: w996 -> [_ w1017]
                frame False {
                }
                frame True {
                  n498 = Unbundle(w1017) -> (w1012:path, w1014:bool, w1015:i32, w1016:string)  [unwired: 1 out]
                  n499 = Bundle(w1014, w1015, w1016) -> (w1013:errorcluster)  [unwired: 1 in]
                  n500 = Read from Text File(file (use dialog)=w1012, error in=w1013) -> (text=w1020:string)  [unwired: 2 in, 3 out]
                  n501 = String Length(string=w1020) -> (length=w1019:i32)
                  n502 = Not Equal To 0?(x=w1019) -> (x != 0?=→"Save analyses file":bool)
                }
              }
              "Cluster 3" <- w1002
            }
          }
          n503 = Equal?(x=w906, y=u16 0) -> (x = y?=w920:bool)
          n504 = Select(t=T9."Enabled" ("Disabled"), s=w920, f=T9."Disabled and Grayed Out") -> (s? t:f=w917:T9)
          n505 = property on="Create analysis file" class="Bool (strict)"("DisabledEnum"=w917) -> ()  [unwired: 2 in, 2 out]
          n506 = Equal?(x=w906, y=u16 1) -> (x = y?=w914:bool)
          n507 = Select(t=T9."Enabled" ("Disabled"), s=w914, f=T9."Disabled and Grayed Out") -> (s? t:f=w911:T9)
          n508 = property on="Save analyses file" class="Bool (strict)"("DisabledEnum"=w911) -> ()  [unwired: 2 in, 2 out]
          n509 = Equal?(x=w906, y=u16 2) -> (x = y?=w909:bool)
          n510 = Select(t=T9."Enabled" ("Disabled"), s=w909, f=T9."Disabled and Grayed Out") -> (s? t:f=w905:T9)
          n511 = property on="Next data file/exit program" class="Bool (strict)"("DisabledEnum"=w905) -> ()  [unwired: 2 in, 2 out]
          n512 = Replace Array Subset(array=w902, new element=w901, index=1 ("Index")) -> (w900:T12)
          n513 = Unbundle(w928) -> (w923:dbl[][], w926:dbl[], w927:cluster{string[], bool[]}, w925:dbl[][], w924:cluster{dbl, string}[])
        }
        frame "Calibration" {
          n514 = Bundle(w1134, w1128, w1127) -> (w1133:cluster{dbl[][], dbl[], cluster{dbl, string}[]})  [unwired: 1 in]
          n515 = case shown="\"SISE channel 1\", Default" "Calibration-channel SISE1/2" {
            tunnel: w1129 -> [w1150 w1488]
            tunnel: [w1153 w1489] -> w1135
            tunnel: w1133 -> [w1155 w1495]
            tunnel: [w1152 w1493] -> w1132
            tunnel: w1127 -> [w1154 w1492]
            tunnel: [w1137 w1475] -> w1125
            tunnel: w1124 -> [w1149 w1487]
            frame "SISE channel 1", Default {
              n516 = Unbundle(w1149) -> (w1148:bool[])  [unwired: 1 out]
              n517 = local read "Ion species ch1"() -> (w1161:bool)
              n518 = local read "Calibration ch1"() -> (w1162:bool)
              n519 = local read "Geometry ch1"() -> (w1163:bool)
              n520 = Index Array(array=w1148, index=8 ("Index")) -> (element=w1138:bool)
              n521 = Index Array(array=w1150, index (col)=8 ("disabled index (col)")) -> (element=w1171:dbl[])  [unwired: 1 in]
              n522 = Add Array Elements(numeric array=w1171) -> (sum=w1170:dbl)
              n523 = And(x=w1161, y=w1162) -> (x .and. y?=w1173:bool)
              n524 = Not Equal To 0?(x=w1170) -> (x != 0?=w1169:bool)
              n525 = And(x=w1173, y=w1163) -> (x .and. y?=w1156:bool)
              n526 = And(x=w1156, y=w1169) -> (x .and. y?=w1157:bool)
              "Update graphs ch1" <- w1157
              n527 = Index Array(array=w1150, index (col)=6 ("Deaktivierter Index (Spalte)")) -> (element=w1158:dbl[])  [unwired: 1 in]
              n528 = Index Array(array=w1150, index (col)=2 ("Deaktivierter Index (Spalte)")) -> (element=w1159:dbl[])  [unwired: 1 in]
              n529 = case shown="\"Ion species\", Default" "Module selection (Calibration window channel 1)" {
                tunnel: w1159 -> [_ _ _ w1313]
                tunnel: dbl[][] [] -> [_ _ _ w1312]
                tunnel: w1157 -> [_ _ _ w1291]
                tunnel: [0 1 2 3] -> w1165
                tunnel: w1150 -> [_ _ _ w1292]
                tunnel: [w1189 w1223 w1232 w1289] -> w1153
                tunnel: w1158 -> [_ _ _ w1310]
                tunnel: [w1190 w1224 w1233 w1286] -> w1152
                tunnel: w1155 -> [w1190 w1224 w1233 w1286]
                tunnel: w1154 -> [_ _ _ w1293]
                tunnel: w1156 -> [_ _ _ w1290]
                tunnel: w1150 -> [w1189 w1223 w1232 w1270]
                tunnel: w1149 -> [w1188 w1222 w1231 w1288]
                tunnel: [w1188 w1222 w1231 w1287] -> w1137
                frame "Ion species", Default {
                  n530 = case shown="8" "Ion Species ch1" {
                    tunnel: [0.0 37.6 7.9 7.9 5.4 8.2 7.7 3.2 2.8] -> w1197
                    tunnel: [0.0 1.0 1.0 1.0 1.0 1.0 1.0 2.0 2.0] -> w1198
                    frame 0, Default {
                    }
                    frame 1 {
                    }
                    frame 2 {
                    }
                    frame 3 {
                    }
                    frame 4 {
                    }
                    frame 5 {
                    }
                    frame 6 {
                    }
                    frame 7 {
                    }
                    frame 8 {
                    }
                  }
                  "Ion mobilty ch1" <- w1197
                  "Valency ch1" <- w1198
                  n531 = Not Equal?(x="Ion Species ch1", y=u16 0) -> (x != y?=w1195:bool)
                  n532 = Not Equal?(x="Ion conc. ch1 (mM)", y=u16 0) -> (x != y?=w1193:bool)
                  n533 = And(x=w1195, y=w1193) -> (x .and. y?=→"Ion species ch1":bool)
                }
                frame "Calibrate" {
                  n534 = call "Calibration-Fit-(SubVI).vi"("Array in"="Array in") -> ("intercept"=→"Intercept ch1":dbl, "slope"=w1221:dbl, "Array out"=→"?":cluster{dbl[], "Best Linear Fit":dbl[]}[], "Array 3"=→"Point #":dbl[])  [unwired: 7 in]
                  "Slope ch1" <- w1221
                  n535 = Not A Number/Path/Refnum?(number/path/refnum=w1221) -> (NaN/Path/Refnum?=w1220:bool)
                  n536 = Not(x=w1220) -> (.not. x?=→"Calibration ch1":bool)
                }
                frame "Geometry" {
                  n537 = local write "Tab Control Geo 2"("Tab Control Geo 1") -> ()
                  n538 = case shown="\"sphere\"" "Tab Control Geo 1" {
                    tunnel: ["Scan Distance  Flat (µm) 1" w1242 w1257] -> w1236
                    frame "flat surface", Default {
                      n539 = local write "Scan Distance  Flat (µm) 2"("Scan Distance  Flat (µm) 1") -> ()
                    }
                    frame "cylinder" {
                      n540 = local write "Scan distance cyl. (µm) 2"("Scan distance cyl. (µm) 1") -> ()
                      n541 = local write "Radius of object cyl. (µm) 2"("Radius of object cyl. (µm) 1") -> ()
                      n542 = local write "Minimum distance to object cyl. (µm) 2"("Minimum distance to object cyl. (µm) 1") -> ()
                      n543 = Add(x="Minimum distance to object cyl. (µm) 1", y="Radius of object cyl. (µm) 1") -> (x+y=w1245:dbl)
                      n544 = Add(x=w1245, y="Scan distance cyl. (µm) 1") -> (x+y=w1246:dbl)
                      n545 = Divide(x=w1246, y=w1245) -> (x/y=w1244:dbl)
                      n546 = Natural Logarithm(1:w1244) -> (0:w1243:dbl)
                      n547 = Multiply(x=w1243, y="Radius of object cyl. (µm) 1") -> (x*y=w1242:dbl)
                    }
                    frame "sphere" {
                      n548 = local write "Scan distance sphere (µm) 2"("Scan distance sphere (µm) 1") -> ()
                      n549 = local write "Radius of object sphere (µm) 2"("Radius of object sphere (µm) 1") -> ()
                      n550 = local write "Minimum distance to object sphere (µm) 2"("Minimum distance to object sphere (µm) 1") -> ()
                      n551 = Add(x="Minimum distance to object sphere (µm) 1", y="Radius of object sphere (µm) 1") -> (x+y=w1252:dbl)
                      n552 = Add(x=w1252, y="Scan distance sphere (µm) 1") -> (x+y=w1253:dbl)
                      n553 = Divide(x=1.0, y=w1252) -> (x/y=w1255:dbl)
                      n554 = Square(x="Radius of object sphere (µm) 1") -> (x^2=w1256:dbl)
                      n555 = Divide(x=1.0, y=w1253) -> (x/y=w1251:dbl)
                      n556 = Subtract(x=w1255, y=w1251) -> (x-y=w1250:dbl)
                      n557 = Multiply(x=w1250, y=w1256) -> (x*y=w1257:dbl)
                    }
                  }
                  "Corrected \ndistance ch1" <- w1236
                  n558 = Not Equal?(x=w1236, y=0.0) -> (x != y?=→"Geometry ch1":bool)
                }
                frame "Update graphs" {
                  n559 = case shown="True" w1290 {
                    tunnel: w1313 -> [_ w1441]
                    tunnel: w1312 -> [_ w1438]
                    tunnel: w1310 -> [_ w1430]
                    tunnel: w1292 -> [w1410 w1425]
                    tunnel: [w1410 w1423] -> w1289
                    tunnel: w1288 -> [w1409 w1413]
                    tunnel: [w1409 w1411] -> w1287
                    frame False {
                    }
                    frame True {
                      w1412 = TRUE
                      w1432 = 1000000000.0  # Scaling, nmol m-2 s-1
                      w1434 = -58.0  # Nernst slope
                      w1435 = 96000.0  # Faraday C.
                      n560 = local read "Corrected \ndistance ch1"() -> (w1433:dbl)
                      n561 = local read "Ion conc. ch1 (mM)"() -> (w1431:dbl)
                      n562 = local read "Ion mobilty ch1"() -> (w1437:dbl)
                      n563 = Unbundle(w1413) -> (w1414:string[], w1419:bool[])
                      n564 = local read "Intercept ch1"() -> (w1440:dbl)
                      n565 = local read "Valency ch1"() -> (w1436:dbl)
                      n566 = local read "Slope ch1"() -> (w1439:dbl)
                      n567 = for {
                        tunnel: w1441 -> [w1445] mode=indexing
                        tunnel: w1440 -> [w1465]
                        tunnel: w1439 -> [w1442]
                        shift-right: [w1469] -> w1422
                        shift-left: w1438 -> [w1470]
                        tunnel: w1437 -> [w1464]
                        tunnel: w1436 -> [w1451]
                        tunnel: w1435 -> [w1460]
                        tunnel: w1434 -> [w1459]
                        tunnel: w1433 -> [w1455]
                        tunnel: w1432 -> [w1448]
                        tunnel: w1431 -> [w1446]
                        tunnel: w1430 -> [w1444] mode=indexing
                        n568 = Divide(x=w1459, y=w1451) -> (x/y=w1458:dbl)
                        n569 = Divide(x=w1455, y=1000.0) -> (x/y=w1453:dbl)
                        n570 = Multiply(x=w1464, y=1e-13) -> (x*y=w1447:dbl)
                        n571 = Subtract(x=w1445, y=w1465) -> (x-y=w1473:dbl)
                        n572 = Divide(x=w1473, y=w1442) -> (x/y=w1472:dbl)
                        n573 = Divide(x=w1444, y=w1453) -> (x/y=w1450:dbl)
                        n574 = Multiply(x=w1446, y=w1447) -> (x*y=w1461:dbl)
                        n575 = Divide(x=w1458, y=w1442) -> (x/y=w1456:dbl)
                        n576 = Multiply(x=w1461, y=w1460) -> (x*y=w1457:dbl)
                        n577 = Multiply(x=-1.0, y=w1472) -> (x*y=w1471:dbl)
                        n578 = Multiply(x=w1457, y=w1456) -> (x*y=w1452:dbl)
                        n579 = Power Of 10(x=w1471) -> (10^x=w1466:dbl)
                        n580 = Multiply(x=w1452, y=w1450) -> (x*y=w1449:dbl)
                        n581 = Multiply(x=w1449, y=w1448) -> (x*y=w1443:dbl)
                        n582 = Multiply(x=w1466, y=1000.0) -> (x*y=w1462:dbl)
                        n583 = Build Array(w1462, w1443) -> (w1468:dbl[])
                        n584 = Insert Into Array(array=w1470, new element=w1468) -> (w1469:dbl[][])  [unwired: 2 in]
                      }
                      n585 = Replace Array Subset(array=w1419, new element=w1412, index=8 ("Index")) -> (w1416:bool[])
                      n586 = Replace Array Subset(array=w1416, new element=w1412, index=10 ("Index")) -> (w1415:bool[])
                      n587 = Bundle(w1414, w1415) -> (w1411:cluster{string[], bool[]})  [unwired: 1 in]
                      n588 = Index Array(array=w1422, index (col)=0 ("Deaktivierter Index (Spalte)")) -> (element=w1429:dbl[])  [unwired: 1 in]
                      n589 = Replace Array Subset(array=w1425, new element=w1429, index (col)=8 ("Deaktivierter Index (Spalte)")) -> (w1424:dbl[][])  [unwired: 1 in]
                      n590 = Index Array(array=w1422, index (col)=1 ("Deaktivierter Index (Spalte)")) -> (element=w1428:dbl[])  [unwired: 1 in]
                      n591 = Replace Array Subset(array=w1424, new element=w1428, index (col)=10 ("Deaktivierter Index (Spalte)")) -> (w1423:dbl[][])  [unwired: 1 in]
                    }
                  }
                  n592 = for {
                    tunnel: w1293 -> [w1406] mode=indexing
                    shift-right: [w1408] -> w1308
                    shift-left: dbl[] [] -> [w1407]
                    n593 = Unbundle(w1406) -> (w1403:dbl)  [unwired: 1 out]
                    n594 = Divide(x=w1403, y=60.0) -> (x/y=w1404:dbl)
                    n595 = Insert Into Array(array=w1407, new element=w1404) -> (w1408:dbl[])  [unwired: 1 in]
                  }
                  n596 = local write "Zoom from start (Cal. modul) 2"("Zoom from start (Cal. modul) ch1") -> ()
                  n597 = Multiply(x="Zoom from end (Cal. modul) ch1", y=-1.0) -> (x*y=w1266:dbl)
                  n598 = local write "Zoom from end (Cal. modul) 2"("Zoom from end (Cal. modul) ch1") -> ()
                  n599 = Add(x="Zoom from start (Cal. modul) ch1", y=w1266) -> (x+y=w1269:dbl)
                  n600 = Greater Or Equal?(x=w1269, y=0.0) -> (x >= y?=w1268:bool)
                  n601 = feedback #3() -> (w1267:dbl)  [unwired: 1 in]
                  n602 = case shown="True" w1268 {
                    tunnel: "Zoom from start (Cal. modul) ch1" -> [w1316 w1319]
                    tunnel: [w1315 w1319] -> w1261
                    tunnel: w1267 -> [w1315 w1321]
                    tunnel: "Zoom from end (Cal. modul) ch1" -> [_ w1318]
                    tunnel: [w1316 w1319] -> w1263
                    tunnel: [w1314 w1317] -> w1262
                    tunnel: "Zoom from end (Cal. modul) ch1" -> [w1314 w1317]
                    frame False {
                    }
                    frame True {
                      n603 = Not Equal?(x=w1321, y=w1319) -> (x != y?=w1320:bool)
                      n604 = case shown="False" w1320 {
                        tunnel: w1319 -> [_ w1323]
                        tunnel: w1318 -> [w1322 _]
                        frame False {
                          n605 = local write "Zoom from start (Cal. modul) ch1"(w1322) -> ()
                        }
                        frame True {
                          n606 = local write "Zoom from end (Cal. modul) ch1"(w1323) -> ()
                        }
                      }
                    }
                  }
                  n607 = feedback-in #3(w1261) -> ()
                  n608 = Array Size(array=w1293) -> (size(s)=w1297:i32)
                  n609 = Divide(x=w1297, y=10) -> (x/y=w1298:dbl)
                  n610 = Multiply(x=w1298, y="Bildlaufleiste") -> (x*y=w1300:dbl)
                  n611 = Array Subset(array=w1293, index=w1300) -> (w1301:cluster{dbl, string}[])  [unwired: 1 in]
                  n612 = Subtract(x=w1262, y=w1263) -> (x-y=w1284:dbl)
                  n613 = Index Array(array=w1270, index (col)=0 ("Deaktivierter Index (Spalte)")) -> (element=w1285:dbl[])  [unwired: 1 in]
                  n614 = for {
                    shift-right: [w1333] -> w1296
                    shift-left: "" -> [w1334]
                    tunnel: w1301 -> [w1332] mode=indexing
                    n615 = Unbundle(w1332) -> (w1330:dbl, w1327:string)
                    n616 = Divide(x=w1330, y=60.0) -> (x/y=w1328:dbl)
                    n617 = Number To Fractional String(number=w1328, precision (6)=i16 2 ("Genauigkeit (6)")) -> (F-format string=w1326:string)  [unwired: 2 in]
                    n618 = Concatenate Strings(w1334, w1326, "min. ,", w1327, "\r") -> (w1333:string)
                  }
                  "?" <- w1296
                  n619 = Divide(x=w1263, y=100.0) -> (x/y=w1282:dbl)
                  n620 = Divide(x=w1284, y=100.0) -> (x/y=w1283:dbl)
                  n621 = Array Size(array=w1285) -> (size(s)=w1281:i32)
                  n622 = Multiply(x=w1281, y=w1282) -> (x*y=w1278:dbl)
                  n623 = Multiply(x=w1281, y=w1283) -> (x*y=w1280:dbl)
                  n624 = Subtract(x=w1278, y=2.0) -> (x-y=w1277:dbl)
                  n625 = Add(x=w1280, y=2.0) -> (x+y=w1279:dbl)
                  n626 = Array Subset(array=w1270, index (row)=w1277, length (row)=w1279) -> (w1271:dbl[][])  [unwired: 2 in]
                  n627 = Index Array(array=w1271, index (col)=0 ("disabled index (col)")) -> (element=w1305:dbl[])  [unwired: 1 in]
                  n628 = Index Array(array=w1271, index (col)=8 ("disabled index (col)")) -> (element=w1304:dbl[])  [unwired: 1 in]
                  n629 = Index Array(array=w1271, index (col)=10 ("disabled index (col)")) -> (element=w1302:dbl[])  [unwired: 1 in]
                  n630 = stacked-sequence {
                    tunnel: w1305 -> [w1336 w1375]
                    tunnel: w1304 -> [w1355 _]
                    tunnel: w1308 -> [w1337 w1369]
                    tunnel: w1302 -> [_ w1374]
                    tunnel: w1291 -> [w1335 w1370]
                    frame #0 {
                      n631 = Array Max & Min(array=w1336) -> (max value=w1347:dbl, min value=w1346:dbl)  [unwired: 2 out]
                      n632 = Divide(x="Range limit\nS1.3 (mM)", y=2.0) -> (x/y=w1365:dbl)
                      n633 = Divide(x="Range limit\nS1.3 (mM)", y=2.05) -> (x/y=w1366:dbl)
                      n634 = Add(x="Base line\nS1.3 (mM)", y=w1365) -> (x+y=w1338:dbl)
                      n635 = Subtract(x="Base line\nS1.3 (mM)", y=w1365) -> (x-y=w1339:dbl)
                      n636 = Subtract(x="Base line\nS1.3 (mM)", y=w1366) -> (x-y=w1345:dbl)
                      n637 = call "EventstoGraph (SubVI).vi"("Numerisch 2"=w1346, "Array 3"=w1337, "Numerisch"=w1347, "Array (Eingang)"=dbl[][] [], "Numerisch 3"=w1345) -> ("Array (Ausgang)"=w1349:dbl[][])  [unwired: 6 in]
                      n638 = Array Max & Min(array=w1336) -> (max value=w1361:dbl, min value=w1362:dbl)  [unwired: 2 out]
                      n639 = call "GraphLimit01.vi"("Numeric 2"=w1339, "Numeric"=w1338, "Array in"=w1355, "Array 3"=dbl[] []) -> ("Array out"=w1354:dbl[])  [unwired: 7 in]
                      n640 = Build Array("Base line\nS1.3 (mM)", "Base line\nS1.3 (mM)") -> (w1358:dbl[])
                      n641 = Build Array(w1361, w1362) -> (w1359:dbl[])
                      n642 = Build Array(w1338, w1339) -> (w1360:dbl[])
                      n643 = Index Array(array=w1349, index (col)=0 ("Index (Zeile)")) -> (element=w1350:dbl[])  [unwired: 1 in]
                      n644 = Index Array(array=w1349, index (col)=1 ("Index (Zeile)")) -> (element=w1348:dbl[])  [unwired: 1 in]
                      n645 = Bundle(w1359, w1360) -> (w1342:cluster{dbl[], dbl[]})  [unwired: 1 in]
                      n646 = Bundle(w1359, w1358) -> (w1343:cluster{dbl[], dbl[]})  [unwired: 1 in]
                      n647 = Bundle(w1336, "Array out"=w1354) -> (w1341:cluster{dbl[], "Array out":dbl[]})  [unwired: 1 in]
                      n648 = Bundle("Array (Ausgang)"=w1350, "Array (Ausgang)"=w1348) -> (w1340:T16)  [unwired: 1 in]
                      n649 = Build Array(w1343, w1342, w1341, w1340) -> (w1344:T17)
                      n650 = case shown="True" w1335 {
                        tunnel: w1344 -> [_ w1368]
                        frame False {
                        }
                        frame True {
                          "Ion conc. SISE channel 1" <- w1368
                        }
                      }
                    }
                    frame #1 {
                      n651 = Array Max & Min(array=w1375) -> (max value=w1384:dbl, min value=w1383:dbl)  [unwired: 2 out]
                      n652 = Divide(x="Range limit\nS1.4", y=2.0) -> (x/y=w1400:dbl)
                      n653 = Divide(x="Range limit\nS1.4", y=2.05) -> (x/y=w1401:dbl)
                      n654 = Add(x="Base line \nS1.4", y=w1400) -> (x+y=w1376:dbl)
                      n655 = Subtract(x="Base line \nS1.4", y=w1400) -> (x-y=w1377:dbl)
                      n656 = Subtract(x="Base line \nS1.4", y=w1401) -> (x-y=w1382:dbl)
                      n657 = call "EventstoGraph (SubVI).vi"("Numerisch 2"=w1383, "Array 3"=w1369, "Numerisch"=w1384, "Array (Eingang)"=dbl[][] [], "Numerisch 3"=w1382) -> ("Array (Ausgang)"=w1386:dbl[][])  [unwired: 6 in]
                      n658 = Array Max & Min(array=w1375) -> (max value=w1396:dbl, min value=w1397:dbl)  [unwired: 2 out]
                      n659 = call "GraphLimit01.vi"("Numeric 2"=w1377, "Numeric"=w1376, "Array in"=w1374, "Array 3"=dbl[] []) -> ("Array out"=w1391:dbl[])  [unwired: 7 in]
                      n660 = Build Array("Base line \nS1.4", "Base line \nS1.4") -> (w1393:dbl[])
                      n661 = Build Array(w1396, w1397) -> (w1394:dbl[])
                      n662 = Build Array(w1376, w1377) -> (w1395:dbl[])
                      n663 = Index Array(array=w1386, index (col)=0 ("Index (Zeile)")) -> (element=w1387:dbl[])  [unwired: 1 in]
                      n664 = Index Array(array=w1386, index (col)=1 ("Index (Zeile)")) -> (element=w1385:dbl[])  [unwired: 1 in]
                      n665 = Bundle(w1394, w1395) -> (w1380:cluster{dbl[], dbl[]})  [unwired: 1 in]
                      n666 = Bundle(w1394, w1393) -> (w1381:cluster{dbl[], dbl[]})  [unwired: 1 in]
                      n667 = Bundle(w1375, "Array out"=w1391) -> (w1379:cluster{dbl[], "Array out":dbl[]})  [unwired: 1 in]
                      n668 = Bundle("Array (Ausgang)"=w1387, "Array (Ausgang)"=w1385) -> (w1378:T16)  [unwired: 1 in]
                      n669 = Build Array(w1381, w1380, w1379, w1378) -> (w1371:T17)
                      n670 = case shown="True" w1370 {
                        tunnel: w1371 -> [_ w1402]
                        frame False {
                        }
                        frame True {
                          "Ion flux SISE channel 1" <- w1402
                        }
                      }
                    }
                  }
                }
              }
              n671 = Equal?(x=w1165, y=u16 0) -> (x = y?=w1146:bool)
              n672 = Or(x=w1138, y=w1146) -> (x .or. y?=w1145:bool)
              n673 = Select(t=T9."Enabled" ("Disabled"), s=w1145, f=T9."Disabled and Grayed Out") -> (s? t:f=w1187:T9)
              n674 = property on="Ion species ch1" class="Bool (strict)"("DisabledEnum"=w1187) -> ()  [unwired: 2 in, 2 out]
              n675 = Equal?(x=w1165, y=u16 1) -> (x = y?=w1143:bool)
              n676 = Or(x=w1138, y=w1143) -> (x .or. y?=w1144:bool)
              n677 = Select(t=T9."Enabled" ("Disabled"), s=w1144, f=T9."Disabled and Grayed Out") -> (s? t:f=w1183:T9)
              n678 = property on="Calibration ch1" class="Bool (strict)"("DisabledEnum"=w1183) -> ()  [unwired: 2 in, 2 out]
              n679 = Equal?(x=w1165, y=u16 2) -> (x = y?=w1141:bool)
              n680 = Or(x=w1138, y=w1141) -> (x .or. y?=w1142:bool)
              n681 = Select(t=T9."Enabled" ("Disabled"), s=w1142, f=T9."Disabled and Grayed Out") -> (s? t:f=w1177:T9)
              n682 = property on="Geometry ch1" class="Bool (strict)"("DisabledEnum"=w1177) -> ()  [unwired: 2 in, 2 out]
              n683 = Equal?(x=w1165, y=u16 3) -> (x = y?=w1139:bool)
              n684 = Or(x=w1138, y=w1139) -> (x .or. y?=w1140:bool)
              n685 = Select(t=T9."Enabled" ("Disabled"), s=w1140, f=T9."Disabled and Grayed Out") -> (s? t:f=w1164:T9)
              n686 = property on="Update graphs ch1" class="Bool (strict)"("DisabledEnum"=w1164) -> ()  [unwired: 2 in, 2 out]
            }
            frame "SISE channel 2" {
              n687 = Unbundle(w1487) -> (w1486:bool[])  [unwired: 1 out]
              n688 = local read "Calibration ch2"() -> (w1500:bool)
              n689 = local read "Ion species ch2"() -> (w1499:bool)
              n690 = local read "Geometry 2"() -> (w1498:bool)
              n691 = Index Array(array=w1486, index=7 ("Index")) -> (element=w1476:bool)
              n692 = Index Array(array=w1488, index (col)=9 ("disabled index (col)")) -> (element=w1503:dbl[])  [unwired: 1 in]
              n693 = Add Array Elements(numeric array=w1503) -> (sum=w1502:dbl)
              n694 = And(x=w1499, y=w1500) -> (x .and. y?=w1501:bool)
              n695 = Not Equal To 0?(x=w1502) -> (x != 0?=w1496:bool)
              n696 = And(x=w1501, y=w1498) -> (x .and. y?=w1497:bool)
              n697 = Index Array(array=w1488, index (col)=7 ("Deaktivierter Index (Spalte)")) -> (element=w1507:dbl[])  [unwired: 1 in]
              n698 = Index Array(array=w1488, index (col)=3 ("Deaktivierter Index (Spalte)")) -> (element=w1506:dbl[])  [unwired: 1 in]
              n699 = And(x=w1497, y=w1496) -> (x .and. y?=w1494:bool)
              "Update graphs ch2" <- w1494
              n700 = case shown="\"Ion species\", Default" "Module selection (Calibration window channel 2)" {
                tunnel: w1506 -> [_ _ _ w1651]
                tunnel: dbl[][] [] -> [_ _ _ w1650]
                tunnel: w1494 -> [_ _ _ w1626]
                tunnel: [0 1 2 3] -> w1510
                tunnel: w1488 -> [_ _ _ w1631]
                tunnel: w1507 -> [_ _ _ w1648]
                tunnel: [w1528 w1562 w1571 w1647] -> w1493
                tunnel: w1495 -> [w1528 w1562 w1571 w1647]
                tunnel: w1492 -> [_ _ _ w1625]
                tunnel: w1497 -> [_ _ _ w1630]
                tunnel: [w1527 w1561 w1570 w1629] -> w1489
                tunnel: w1488 -> [w1527 w1561 w1570 w1600]
                tunnel: w1487 -> [w1526 w1560 w1569 w1628]
                tunnel: [w1526 w1560 w1569 w1627] -> w1475
                frame "Ion species", Default {
                  n701 = case shown="8" "Ion Species ch2" {
                    tunnel: [0.0 37.6 7.9 7.9 5.4 8.2 7.7 3.2 2.8] -> w1535
                    tunnel: [0.0 1.0 1.0 1.0 1.0 -1.0 -1.0 2.0 2.0] -> w1536
                    frame 0, Default {
                    }
                    frame 1 {
                    }
                    frame 2 {
                    }
                    frame 3 {
                    }
                    frame 4 {
                    }
                    frame 5 {
                    }
                    frame 6 {
                    }
                    frame 7 {
                    }
                    frame 8 {
                    }
                  }
                  "Ion mobilty ch2" <- w1535
                  "Valency ch2" <- w1536
                  n702 = Not Equal?(x="Ion Species ch2", y=u16 0) -> (x != y?=w1533:bool)
                  n703 = Not Equal?(x="Ion conc. ch2 (mM)", y=u16 0) -> (x != y?=w1531:bool)
                  n704 = And(x=w1533, y=w1531) -> (x .and. y?=→"Ion species ch2":bool)
                }
                frame "Calibrate" {
                  n705 = call "Calibration-Fit-(SubVI).vi"("Array in"="Array in 2") -> ("intercept"=→"Intercept ch2":dbl, "slope"=w1559:dbl, "Array out"=→"?":cluster{dbl[], "Best Linear Fit":dbl[]}[], "Array 3"=→"Point # 2":dbl[])  [unwired: 7 in]
                  "Slope ch2" <- w1559
                  n706 = Not A Number/Path/Refnum?(number/path/refnum=w1559) -> (NaN/Path/Refnum?=w1558:bool)
                  n707 = Not(x=w1558) -> (.not. x?=→"Calibration ch2":bool)
                }
                frame "Geometry" {
                  n708 = local write "Tab Control Geo 1"("Tab Control Geo 2") -> ()
                  n709 = case shown="\"flat surface\", Default" "Tab Control Geo 2" {
                    tunnel: ["Scan Distance  Flat (µm) 2" w1580 w1595] -> w1574
                    frame "flat surface", Default {
                      n710 = local write "Scan Distance  Flat (µm) 1"("Scan Distance  Flat (µm) 2") -> ()
                    }
                    frame "cylinder" {
                      n711 = Add(x="Minimum distance to object cyl. (µm) 2", y="Radius of object cyl. (µm) 2") -> (x+y=w1583:dbl)
                      n712 = local write "Scan distance cyl. (µm) 1"("Scan distance cyl. (µm) 2") -> ()
                      n713 = local write "Radius of object cyl. (µm) 1"("Radius of object cyl. (µm) 2") -> ()
                      n714 = local write "Minimum distance to object cyl. (µm) 1"("Minimum distance to object cyl. (µm) 2") -> ()
                      n715 = Add(x=w1583, y="Scan distance cyl. (µm) 2") -> (x+y=w1584:dbl)
                      n716 = Divide(x=w1584, y=w1583) -> (x/y=w1582:dbl)
                      n717 = Natural Logarithm(1:w1582) -> (0:w1581:dbl)
                      n718 = Multiply(x=w1581, y="Radius of object cyl. (µm) 2") -> (x*y=w1580:dbl)
                    }
                    frame "sphere" {
                      n719 = local write "Scan distance sphere (µm) 1"("Scan distance sphere (µm) 2") -> ()
                      n720 = local write "Radius of object sphere (µm) 1"("Radius of object sphere (µm) 2") -> ()
                      n721 = local write "Minimum distance to object sphere (µm) 1"("Minimum distance to object sphere (µm) 2") -> ()
                      n722 = Add(x="Minimum distance to object sphere (µm) 2", y="Radius of object sphere (µm) 2") -> (x+y=w1590:dbl)
                      n723 = Add(x=w1590, y="Scan distance sphere (µm) 2") -> (x+y=w1591:dbl)
                      n724 = Divide(x=1.0, y=w1590) -> (x/y=w1593:dbl)
                      n725 = Square(x="Radius of object sphere (µm) 2") -> (x^2=w1594:dbl)
                      n726 = Divide(x=1.0, y=w1591) -> (x/y=w1589:dbl)
                      n727 = Subtract(x=w1593, y=w1589) -> (x-y=w1588:dbl)
                      n728 = Multiply(x=w1588, y=w1594) -> (x*y=w1595:dbl)
                    }
                  }
                  "Corrected \ndistance ch2" <- w1574
                  n729 = Not Equal?(x=w1574, y=0.0) -> (x != y?=→"Geometry 2":bool)
                }
                frame "Update graphs" {
                  n730 = case shown="True" w1630 {
                    tunnel: w1651 -> [_ w1779]
                    tunnel: w1650 -> [_ w1776]
                    tunnel: w1648 -> [_ w1768]
                    tunnel: w1631 -> [w1748 w1763]
                    tunnel: [w1748 w1761] -> w1629
                    tunnel: w1628 -> [w1747 w1757]
                    tunnel: [w1747 w1749] -> w1627
                    frame False {
                    }
                    frame True {
                      w1752 = TRUE
                      w1770 = 1000000000.0  # Scaling, nmol m-2 s-1
                      w1772 = -58.0  # Nernst slope
                      w1773 = 96000.0  # Faraday C.
                      n731 = local read "Corrected \ndistance ch2"() -> (w1771:dbl)
                      n732 = local read "Ion conc. ch2 (mM)"() -> (w1769:dbl)
                      n733 = Unbundle(w1757) -> (w1750:string[], w1756:bool[])
                      n734 = local read "Ion mobilty ch2"() -> (w1775:dbl)
                      n735 = local read "Intercept ch2"() -> (w1778:dbl)
                      n736 = local read "Valency ch2"() -> (w1774:dbl)
                      n737 = local read "Slope ch2"() -> (w1777:dbl)
                      n738 = Replace Array Subset(array=w1756, new element=w1752, index=9 ("Index")) -> (w1753:bool[])
                      n739 = for {
                        tunnel: w1779 -> [w1781] mode=indexing
                        tunnel: w1778 -> [w1803]
                        tunnel: w1777 -> [w1796]
                        shift-right: [w1807] -> w1760
                        shift-left: w1776 -> [w1808]
                        tunnel: w1775 -> [w1802]
                        tunnel: w1774 -> [w1788]
                        tunnel: w1773 -> [w1798]
                        tunnel: w1772 -> [w1797]
                        tunnel: w1771 -> [w1792]
                        tunnel: w1770 -> [w1785]
                        tunnel: w1769 -> [w1782]
                        tunnel: w1768 -> [w1780] mode=indexing
                        n740 = Divide(x=w1797, y=w1788) -> (x/y=w1795:dbl)
                        n741 = Divide(x=w1792, y=1000.0) -> (x/y=w1790:dbl)
                        n742 = Multiply(x=w1802, y=1e-13) -> (x*y=w1784:dbl)
                        n743 = Subtract(x=w1781, y=w1803) -> (x-y=w1811:dbl)
                        n744 = Divide(x=w1811, y=w1796) -> (x/y=w1810:dbl)
                        n745 = Divide(x=w1780, y=w1790) -> (x/y=w1787:dbl)
                        n746 = Multiply(x=w1782, y=w1784) -> (x*y=w1799:dbl)
                        n747 = Divide(x=w1795, y=w1796) -> (x/y=w1793:dbl)
                        n748 = Multiply(x=w1799, y=w1798) -> (x*y=w1794:dbl)
                        n749 = Multiply(x=-1.0, y=w1810) -> (x*y=w1809:dbl)
                        n750 = Multiply(x=w1794, y=w1793) -> (x*y=w1789:dbl)
                        n751 = Power Of 10(x=w1809) -> (10^x=w1804:dbl)
                        n752 = Multiply(x=w1789, y=w1787) -> (x*y=w1786:dbl)
                        n753 = Multiply(x=w1786, y=w1785) -> (x*y=w1783:dbl)
                        n754 = Multiply(x=w1804, y=1000.0) -> (x*y=w1800:dbl)
                        n755 = Build Array(w1800, w1783) -> (w1806:dbl[])
                        n756 = Insert Into Array(array=w1808, new element=w1806) -> (w1807:dbl[][])  [unwired: 2 in]
                      }
                      n757 = Replace Array Subset(array=w1753, new element=w1752, index=11 ("Index")) -> (w1751:bool[])
                      n758 = Bundle(w1750, w1751) -> (w1749:cluster{string[], bool[]})  [unwired: 1 in]
                      n759 = Index Array(array=w1760, index (col)=0 ("Deaktivierter Index (Spalte)")) -> (element=w1767:dbl[])  [unwired: 1 in]
                      n760 = Replace Array Subset(array=w1763, new element=w1767, index (col)=9 ("Deaktivierter Index (Spalte)")) -> (w1762:dbl[][])  [unwired: 1 in]
                      n761 = Index Array(array=w1760, index (col)=1 ("Deaktivierter Index (Spalte)")) -> (element=w1766:dbl[])  [unwired: 1 in]
                      n762 = Replace Array Subset(array=w1762, new element=w1766, index (col)=11 ("Deaktivierter Index (Spalte)")) -> (w1761:dbl[][])  [unwired: 1 in]
                    }
                  }
                  n763 = for {
                    tunnel: w1625 -> [w1744] mode=indexing
                    shift-right: [w1746] -> w1624
                    shift-left: dbl[] [] -> [w1745]
                    n764 = Unbundle(w1744) -> (w1741:dbl)  [unwired: 1 out]
                    n765 = Divide(x=w1741, y=60.0) -> (x/y=w1742:dbl)
                    n766 = Insert Into Array(array=w1745, new element=w1742) -> (w1746:dbl[])  [unwired: 1 in]
                  }
                  n767 = local write "Zoom from start (Cal. modul) ch1"("Zoom from start (Cal. modul) 2") -> ()
                  n768 = Multiply(x="Zoom from end (Cal. modul) 2", y=-1.0) -> (x*y=w1606:dbl)
                  n769 = local write "Zoom from end (Cal. modul) ch1"("Zoom from end (Cal. modul) 2") -> ()
                  n770 = Add(x="Zoom from start (Cal. modul) 2", y=w1606) -> (x+y=w1609:dbl)
                  n771 = feedback #4() -> (w1607:dbl)  [unwired: 1 in]
                  n772 = Greater Or Equal?(x=w1609, y=0.0) -> (x >= y?=w1608:bool)
                  n773 = case shown="True" w1608 {
                    tunnel: "Zoom from start (Cal. modul) 2" -> [w1654 w1657]
                    tunnel: [w1653 w1657] -> w1601
                    tunnel: w1607 -> [w1653 w1659]
                    tunnel: "Zoom from end (Cal. modul) 2" -> [_ w1656]
                    tunnel: [w1654 w1657] -> w1603
                    tunnel: [w1652 w1655] -> w1602
                    tunnel: "Zoom from end (Cal. modul) 2" -> [w1652 w1655]
                    frame False {
                    }
                    frame True {
                      n774 = Not Equal?(x=w1659, y=w1657) -> (x != y?=w1658:bool)
                      n775 = case shown="True" w1658 {
                        tunnel: w1657 -> [_ w1661]
                        tunnel: w1656 -> [w1660 _]
                        frame False {
                          n776 = local write "Zoom from start (Cal. modul) 2"(w1660) -> ()
                        }
                        frame True {
                          n777 = local write "Zoom from end (Cal. modul) 2"(w1661) -> ()
                        }
                      }
                    }
                  }
                  n778 = feedback-in #4(w1601) -> ()
                  n779 = Array Size(array=w1625) -> (size(s)=w1635:i32)
                  n780 = Divide(x=w1635, y=10) -> (x/y=w1636:dbl)
                  n781 = Multiply(x=w1636, y="Bildlaufleiste 2") -> (x*y=w1638:dbl)
                  n782 = Array Subset(array=w1625, index=w1638) -> (w1639:cluster{dbl, string}[])  [unwired: 1 in]
                  n783 = Subtract(x=w1602, y=w1603) -> (x-y=w1622:dbl)
                  n784 = Index Array(array=w1600, index (col)=0 ("Deaktivierter Index (Spalte)")) -> (element=w1623:dbl[])  [unwired: 1 in]
                  n785 = for {
                    shift-right: [w1671] -> w1634
                    shift-left: "" -> [w1672]
                    tunnel: w1639 -> [w1670] mode=indexing
                    n786 = Unbundle(w1670) -> (w1668:dbl, w1665:string)
                    n787 = Divide(x=w1668, y=60.0) -> (x/y=w1666:dbl)
                    n788 = Number To Fractional String(number=w1666, precision (6)=i16 2 ("Genauigkeit (6)")) -> (F-format string=w1664:string)  [unwired: 2 in]
                    n789 = Concatenate Strings(w1672, w1664, "min. ,", w1665, "\r") -> (w1671:string)
                  }
                  "?" <- w1634
                  n790 = Divide(x=w1603, y=100.0) -> (x/y=w1620:dbl)
                  n791 = Divide(x=w1622, y=100.0) -> (x/y=w1621:dbl)
                  n792 = Array Size(array=w1623) -> (size(s)=w1619:i32)
                  n793 = Multiply(x=w1619, y=w1620) -> (x*y=w1616:dbl)
                  n794 = Multiply(x=w1619, y=w1621) -> (x*y=w1618:dbl)
                  n795 = Subtract(x=w1616, y=2.0) -> (x-y=w1615:dbl)
                  n796 = Add(x=w1618, y=2.0) -> (x+y=w1617:dbl)
                  n797 = Array Subset(array=w1600, index (row)=w1615, length (row)=w1617) -> (w1599:dbl[][])  [unwired: 2 in]
                  n798 = Index Array(array=w1599, index (col)=0 ("disabled index (col)")) -> (element=w1643:dbl[])  [unwired: 1 in]
                  n799 = Index Array(array=w1599, index (col)=9 ("disabled index (col)")) -> (element=w1642:dbl[])  [unwired: 1 in]
                  n800 = Index Array(array=w1599, index (col)=11 ("disabled index (col)")) -> (element=w1640:dbl[])  [unwired: 1 in]
                  n801 = stacked-sequence {
                    tunnel: w1643 -> [w1674 w1713]
                    tunnel: w1642 -> [w1693 _]
                    tunnel: w1624 -> [w1675 w1707]
                    tunnel: w1640 -> [_ w1712]
                    tunnel: w1626 -> [w1673 w1708]
                    frame #0 {
                      n802 = Array Max & Min(array=w1674) -> (max value=w1685:dbl, min value=w1684:dbl)  [unwired: 2 out]
                      n803 = Divide(x="Range limit\nS2.3 (mM)", y=2.0) -> (x/y=w1703:dbl)
                      n804 = Divide(x="Range limit\nS2.3 (mM)", y=2.05) -> (x/y=w1704:dbl)
                      n805 = Add(x="Base line\nS2.3 (mM)", y=w1703) -> (x+y=w1676:dbl)
                      n806 = Subtract(x="Base line\nS2.3 (mM)", y=w1703) -> (x-y=w1677:dbl)
                      n807 = Subtract(x="Base line\nS2.3 (mM)", y=w1704) -> (x-y=w1683:dbl)
                      n808 = call "EventstoGraph (SubVI).vi"("Numerisch 2"=w1684, "Array 3"=w1675, "Numerisch"=w1685, "Array (Eingang)"=dbl[][] [], "Numerisch 3"=w1683) -> ("Array (Ausgang)"=w1687:dbl[][])  [unwired: 6 in]
                      n809 = Array Max & Min(array=w1674) -> (max value=w1699:dbl, min value=w1700:dbl)  [unwired: 2 out]
                      n810 = call "GraphLimit01.vi"("Numeric 2"=w1677, "Numeric"=w1676, "Array in"=w1693, "Array 3"=dbl[] []) -> ("Array out"=w1692:dbl[])  [unwired: 7 in]
                      n811 = Build Array("Base line\nS2.3 (mM)", "Base line\nS2.3 (mM)") -> (w1696:dbl[])
                      n812 = Build Array(w1699, w1700) -> (w1697:dbl[])
                      n813 = Build Array(w1676, w1677) -> (w1698:dbl[])
                      n814 = Index Array(array=w1687, index (col)=0 ("Index (Zeile)")) -> (element=w1688:dbl[])  [unwired: 1 in]
                      n815 = Index Array(array=w1687, index (col)=1 ("Index (Zeile)")) -> (element=w1686:dbl[])  [unwired: 1 in]
                      n816 = Bundle(w1697, w1698) -> (w1680:cluster{dbl[], dbl[]})  [unwired: 1 in]
                      n817 = Bundle(w1697, w1696) -> (w1681:cluster{dbl[], dbl[]})  [unwired: 1 in]
                      n818 = Bundle(w1674, "Array out"=w1692) -> (w1679:cluster{dbl[], "Array out":dbl[]})  [unwired: 1 in]
                      n819 = Bundle("Array (Ausgang)"=w1688, "Array (Ausgang)"=w1686) -> (w1678:T16)  [unwired: 1 in]
                      n820 = Build Array(w1681, w1680, w1679, w1678) -> (w1682:T17)
                      n821 = case shown="True" w1673 {
                        tunnel: w1682 -> [_ w1706]
                        frame False {
                        }
                        frame True {
                          "Ion conc. SISE channel 2" <- w1706
                        }
                      }
                    }
                    frame #1 {
                      n822 = Array Max & Min(array=w1713) -> (max value=w1722:dbl, min value=w1721:dbl)  [unwired: 2 out]
                      n823 = Divide(x="Range limit\nS2.4", y=2.0) -> (x/y=w1738:dbl)
                      n824 = Divide(x="Range limit\nS2.4", y=2.05) -> (x/y=w1739:dbl)
                      n825 = Add(x="Base line \nS2.4", y=w1738) -> (x+y=w1714:dbl)
                      n826 = Subtract(x="Base line \nS2.4", y=w1738) -> (x-y=w1715:dbl)
                      n827 = Subtract(x="Base line \nS2.4", y=w1739) -> (x-y=w1720:dbl)
                      n828 = call "EventstoGraph (SubVI).vi"("Numerisch 2"=w1721, "Array 3"=w1707, "Numerisch"=w1722, "Array (Eingang)"=dbl[][] [], "Numerisch 3"=w1720) -> ("Array (Ausgang)"=w1724:dbl[][])  [unwired: 6 in]
                      n829 = Array Max & Min(array=w1713) -> (max value=w1734:dbl, min value=w1735:dbl)  [unwired: 2 out]
                      n830 = call "GraphLimit01.vi"("Numeric 2"=w1715, "Numeric"=w1714, "Array in"=w1712, "Array 3"=dbl[] []) -> ("Array out"=w1729:dbl[])  [unwired: 7 in]
                      n831 = Build Array("Base line \nS2.4", "Base line \nS2.4") -> (w1731:dbl[])
                      n832 = Build Array(w1734, w1735) -> (w1732:dbl[])
                      n833 = Build Array(w1714, w1715) -> (w1733:dbl[])
                      n834 = Index Array(array=w1724, index (col)=0 ("Index (Zeile)")) -> (element=w1725:dbl[])  [unwired: 1 in]
                      n835 = Index Array(array=w1724, index (col)=1 ("Index (Zeile)")) -> (element=w1723:dbl[])  [unwired: 1 in]
                      n836 = Bundle(w1732, w1733) -> (w1718:cluster{dbl[], dbl[]})  [unwired: 1 in]
                      n837 = Bundle(w1732, w1731) -> (w1719:cluster{dbl[], dbl[]})  [unwired: 1 in]
                      n838 = Bundle(w1713, "Array out"=w1729) -> (w1717:cluster{dbl[], "Array out":dbl[]})  [unwired: 1 in]
                      n839 = Bundle("Array (Ausgang)"=w1725, "Array (Ausgang)"=w1723) -> (w1716:T16)  [unwired: 1 in]
                      n840 = Build Array(w1719, w1718, w1717, w1716) -> (w1709:T17)
                      n841 = case shown="True" w1708 {
                        tunnel: w1709 -> [_ w1740]
                        frame False {
                        }
                        frame True {
                          "Ion flux SISE channel 2" <- w1740
                        }
                      }
                    }
                  }
                }
              }
              n842 = Equal?(x=w1510, y=u16 0) -> (x = y?=w1484:bool)
              n843 = Or(x=w1476, y=w1484) -> (x .or. y?=w1483:bool)
              n844 = Select(t=T9."Enabled" ("Disabled"), s=w1483, f=T9."Disabled and Grayed Out") -> (s? t:f=w1525:T9)
              n845 = property on="Ion species ch2" class="Bool (strict)"("DisabledEnum"=w1525) -> ()  [unwired: 2 in, 2 out]
              n846 = Equal?(x=w1510, y=u16 1) -> (x = y?=w1481:bool)
              n847 = Or(x=w1476, y=w1481) -> (x .or. y?=w1482:bool)
              n848 = Select(t=T9."Enabled" ("Disabled"), s=w1482, f=T9."Disabled and Grayed Out") -> (s? t:f=w1521:T9)
              n849 = property on="Calibration ch2" class="Bool (strict)"("DisabledEnum"=w1521) -> ()  [unwired: 2 in, 2 out]
              n850 = Equal?(x=w1510, y=u16 2) -> (x = y?=w1479:bool)
              n851 = Or(x=w1476, y=w1479) -> (x .or. y?=w1480:bool)
              n852 = Select(t=T9."Enabled" ("Disabled"), s=w1480, f=T9."Disabled and Grayed Out") -> (s? t:f=w1515:T9)
              n853 = property on="Geometry 2" class="Bool (strict)"("DisabledEnum"=w1515) -> ()  [unwired: 2 in, 2 out]
              n854 = Equal?(x=w1510, y=u16 3) -> (x = y?=w1477:bool)
              n855 = Or(x=w1476, y=w1477) -> (x .or. y?=w1478:bool)
              n856 = Select(t=T9."Enabled" ("Disabled"), s=w1478, f=T9."Disabled and Grayed Out") -> (s? t:f=w1491:T9)
              n857 = property on="Update graphs ch2" class="Bool (strict)"("DisabledEnum"=w1491) -> ()  [unwired: 2 in, 2 out]
            }
          }
          n858 = Unbundle(w1132) -> (w1131:dbl[][], w1130:dbl[], w1126:cluster{dbl, string}[])
        }
        frame "Buffer correction" {
          n859 = Bundle(w1822, w1821, w1820) -> (w1819:cluster{dbl[][], dbl[], cluster{dbl, string}[]})  [unwired: 1 in]
          n860 = case shown="\"SISE channel 2, buffer corr.\"" "SISE channel selection (buffer corr.)" {
            tunnel: w1813 -> [w1833 w2070]
            tunnel: w1824 -> [w1842 w2080]
            tunnel: [w1841 w2079] -> w1825
            tunnel: w1820 -> [w1838 w2078]
            tunnel: w1824 -> [w1840 w2077]
            tunnel: [w1839 w2076] -> w1823
            tunnel: w1813 -> [w1827 w2066]
            frame "SISE channel 2, buffer corr." {
              n861 = local read "Buffer species ch2"() -> (w1831:bool)
              n862 = local read "Buffer conc. ch2"() -> (w1832:bool)
              n863 = Index Array(array=w1833, index (col)=13 ("disabled index (col)")) -> (element=w1836:dbl[])  [unwired: 1 in]
              n864 = Unbundle(w1842) -> (w1852:bool[])  [unwired: 1 out]
              n865 = Add Array Elements(numeric array=w1836) -> (sum=w1835:dbl)
              n866 = And(x=w1831, y=w1832) -> (x .and. y?=w1830:bool)
              n867 = Not Equal To 0?(x=w1835) -> (x != 0?=w1834:bool)
              n868 = Index Array(array=w1852, index=9 ("Index")) -> (element=w1850:bool)
              n869 = Index Array(array=w1852, index=11 ("Index")) -> (element=w1851:bool)
              n870 = And(x=w1830, y=w1834) -> (x .and. y?=w1829:bool)
              "Update graphs (buffer corr.) ch2" <- w1829
              n871 = And(x=w1850, y=w1851) -> (x .and. y?=w1843:bool)
              n872 = case shown="\"Update graphs\"" "Module selection ch2 (buffer corr.)" {
                tunnel: [0 1 2] -> w1855
                tunnel: w1833 -> [w1875 w1896 w1933]
                tunnel: [w1875 w1896 w1932] -> w1841
                tunnel: w1840 -> [w1874 w1895 w1935]
                tunnel: [w1874 w1895 w1934] -> w1839
                tunnel: w1838 -> [_ _ w1936]
                tunnel: w1830 -> [_ _ w1901]
                tunnel: w1829 -> [_ _ w1903]
                tunnel: w1827 -> [_ _ w1907]
                frame "Buffer species", Default {
                  n873 = case shown="\"HEPES\"" "Select buffer ch 2" {
                    tunnel: ["" "Mes" "Malate (pH 5)" "Citrate (pH 5)" "TRIS" "HEPES"] -> w1873
                    tunnel: [0.0 6.2 5.1 4.8 8.2 7.5] -> w1871
                    tunnel: [0.0 2.9 3.2 2.5 3.2 2.4] -> w1872
                    frame "none", Default {
                    }
                    frame "Mes" {
                    }
                    frame "Malate (pH 5)" {
                    }
                    frame "Citrate (pH 5)" {
                    }
                    frame "TRIS" {
                    }
                    frame "HEPES" {
                    }
                  }
                  "pKs ch2" <- w1871
                  "Buffer Mobilty ch2" <- w1872
                  n874 = Not Equal?(x="", y=w1873) -> (x != y?=→"Buffer species ch2":bool)
                }
                frame "Buffer conc." {
                  n875 = Not Equal To 0?(x="Buffer conc. ch2 (mM)") -> (x != 0?=→"Buffer conc. ch2":bool)
                }
                frame "Update graphs" {
                  n876 = Not(x=w1903) -> (.not. x?=w1904:bool)
                  n877 = And(x=w1901, y=w1904) -> (x .and. y?=w1902:bool)
                  n878 = Index Array(array=w1933, index (col)=11 ("Deaktivierter Index (Spalte)")) -> (element=w1952:dbl[])  [unwired: 1 in]
                  n879 = local write "Zoom from start (Buffer corr. modul) ch1"("Zoom from start (Buffer corr. modul) ch2") -> ()
                  n880 = local write "Zoom from end (Buffer corr. modul) ch1"("Zoom from end (Buffer corr. modul) ch2") -> ()
                  n881 = for {
                    tunnel: w1936 -> [w1983] mode=indexing
                    shift-right: [w1985] -> w1945
                    shift-left: dbl[] [] -> [w1984]
                    n882 = Unbundle(w1983) -> (w1980:dbl)  [unwired: 1 out]
                    n883 = Divide(x=w1980, y=60.0) -> (x/y=w1981:dbl)
                    n884 = Insert Into Array(array=w1984, new element=w1981) -> (w1985:dbl[])  [unwired: 1 in]
                  }
                  n885 = local read "Ion conc. ch2 (mM)"() -> (w1900:dbl)
                  n886 = local read "pKs ch2"() -> (w1957:dbl)
                  n887 = local read "Buffer Mobilty ch2"() -> (w1954:dbl)
                  n888 = local read "Ion mobilty ch2"() -> (w1955:dbl)
                  n889 = local read "Buffer conc. ch2 (mM)"() -> (w1956:dbl)
                  n890 = Multiply(x="Zoom from end (Buffer corr. modul) ch2", y=-1.0) -> (x*y=w1924:dbl)
                  n891 = Add(x="Zoom from start (Buffer corr. modul) ch2", y=w1924) -> (x+y=w1918:dbl)
                  n892 = case shown="True" w1902 {
                    tunnel: dbl[] [] -> [_ w2037]
                    tunnel: w1954 -> [_ w2039]
                    tunnel: w1955 -> [_ w2040]
                    tunnel: w1957 -> [_ w2036]
                    tunnel: w1956 -> [_ w2035]
                    tunnel: w1952 -> [_ w2034]
                    tunnel: w1935 -> [w2021 w2028]
                    tunnel: [w2021 w2027] -> w1934
                    tunnel: w1933 -> [w2020 w2025]
                    tunnel: [w2020 w2024] -> w1932
                    tunnel: w1900 -> [_ w2022]
                    frame False {
                    }
                    frame True {
                      n893 = Divide(x=w2039, y=w2040) -> (x/y=w2038:dbl)
                      n894 = for {
                        tunnel: w2038 -> [w2049]
                        tunnel: w2036 -> [w2059]
                        tunnel: w2035 -> [w2053]
                        shift-right: [w2044] -> w2026
                        shift-left: w2037 -> [w2045]
                        tunnel: w2034 -> [w2043] mode=indexing
                        tunnel: w2022 -> [w2041]
                        n895 = Multiply(x=w2041, y=0.001) -> (x*y=w2063:dbl)
                        n896 = Multiply(x=w2053, y=0.001) -> (x*y=w2050:dbl)
                        n897 = Logarithm Base 10(1:w2063) -> (0:w2062:dbl)
                        n898 = Multiply(x=w2062, y=-1.0) -> (x*y=w2060:dbl)
                        n899 = Power Of 10(x=w2060) -> (10^x=w2057:dbl)
                        n900 = Power Of 10(x=w2059) -> (10^x=w2054:dbl)
                        n901 = Add(x=w2057, y=w2054) -> (x+y=w2058:dbl)
                        n902 = Divide(x=w2057, y=w2058) -> (x/y=w2056:dbl)
                        n903 = Square(x=w2056) -> (x^2=w2055:dbl)
                        n904 = Multiply(x=w2055, y=w2054) -> (x*y=w2051:dbl)
                        n905 = Multiply(x=w2051, y=w2050) -> (x*y=w2048:dbl)
                        n906 = Multiply(x=w2048, y=w2049) -> (x*y=w2047:dbl)
                        n907 = Multiply(x=w2047, y=w2043) -> (x*y=w2046:dbl)
                        n908 = Add(x=w2046, y=w2043) -> (x+y=w2042:dbl)
                        n909 = Insert Into Array(array=w2045, new element=w2042) -> (w2044:dbl[])  [unwired: 1 in]
                      }
                      n910 = Unbundle(w2028) -> (w2033:string[], w2031:bool[])
                      n911 = Replace Array Subset(array=w2031, new element=TRUE, index=13 ("Index")) -> (w2032:bool[])
                      n912 = Bundle(w2033, w2032) -> (w2027:cluster{string[], bool[]})  [unwired: 1 in]
                      n913 = Insert Into Array(array=w2025, index (col)=13 ("Deaktivierter Index (Spalte)"), new element=w2026) -> (w2024:dbl[][])  [unwired: 1 in]
                    }
                  }
                  n914 = feedback #5() -> (w1920:dbl)  [unwired: 1 in]
                  n915 = Greater Or Equal?(x=w1918, y=0.0) -> (x >= y?=w1919:bool)
                  n916 = case shown="True" w1919 {
                    tunnel: "Zoom from start (Buffer corr. modul) ch2" -> [w1961 w1964]
                    tunnel: [w1960 w1964] -> w1909
                    tunnel: w1920 -> [w1960 w1966]
                    tunnel: "Zoom from end (Buffer corr. modul) ch2" -> [_ w1963]
                    tunnel: [w1961 w1964] -> w1925
                    tunnel: [w1959 w1962] -> w1926
                    tunnel: "Zoom from end (Buffer corr. modul) ch2" -> [w1959 w1962]
                    frame False {
                    }
                    frame True {
                      n917 = Not Equal?(x=w1966, y=w1964) -> (x != y?=w1965:bool)
                      n918 = case shown="False" w1965 {
                        tunnel: w1964 -> [_ w1968]
                        tunnel: w1963 -> [w1967 _]
                        frame False {
                          n919 = local write "Zoom from start (Buffer corr. modul) ch2"(w1967) -> ()
                        }
                        frame True {
                          n920 = local write "Zoom from end (Buffer corr. modul) ch2"(w1968) -> ()
                        }
                      }
                    }
                  }
                  n921 = feedback-in #5(w1909) -> ()
                  n922 = Array Size(array=w1936) -> (size(s)=w1940:i32)
                  n923 = Divide(x=w1940, y=10) -> (x/y=w1941:dbl)
                  n924 = Multiply(x=w1941, y="Bildlaufleiste 4") -> (x*y=w1943:dbl)
                  n925 = Array Subset(array=w1936, index=w1943) -> (w1944:cluster{dbl, string}[])  [unwired: 1 in]
                  n926 = Subtract(x=w1926, y=w1925) -> (x-y=w1921:dbl)
                  n927 = for {
                    shift-right: [w1978] -> w1939
                    shift-left: "" -> [w1979]
                    tunnel: w1944 -> [w1977] mode=indexing
                    n928 = Unbundle(w1977) -> (w1975:dbl, w1972:string)
                    n929 = Divide(x=w1975, y=60.0) -> (x/y=w1973:dbl)
                    n930 = Number To Fractional String(number=w1973, precision (6)=i16 2 ("Genauigkeit (6)")) -> (F-format string=w1971:string)  [unwired: 2 in]
                    n931 = Concatenate Strings(w1979, w1971, "min. ,", w1972, "\r") -> (w1978:string)
                  }
                  "?" <- w1939
                  n932 = Index Array(array=w1907, index (col)=0 ("Deaktivierter Index (Spalte)")) -> (element=w1917:dbl[])  [unwired: 1 in]
                  n933 = Divide(x=w1925, y=100.0) -> (x/y=w1923:dbl)
                  n934 = Divide(x=w1921, y=100.0) -> (x/y=w1922:dbl)
                  n935 = Array Size(array=w1917) -> (size(s)=w1927:i32)
                  n936 = Multiply(x=w1927, y=w1923) -> (x*y=w1930:dbl)
                  n937 = Multiply(x=w1927, y=w1922) -> (x*y=w1928:dbl)
                  n938 = Add(x=w1928, y=2.0) -> (x+y=w1929:dbl)
                  n939 = Subtract(x=w1930, y=2.0) -> (x-y=w1931:dbl)
                  n940 = Array Subset(array=w1907, index (row)=w1931, length (row)=w1929) -> (w1908:dbl[][])  [unwired: 2 in]
                  n941 = Index Array(array=w1908, index (col)=0 ("disabled index (col)")) -> (element=w1949:dbl[])  [unwired: 1 in]
                  n942 = Index Array(array=w1908, index (col)=13 ("disabled index (col)")) -> (element=w1947:dbl[])  [unwired: 1 in]
                  n943 = stacked-sequence {
                    tunnel: w1949 -> [w1992]
                    tunnel: w1945 -> [w1986]
                    tunnel: w1947 -> [w1991]
                    tunnel: w1903 -> [w1987]
                    frame #0 {
                      n944 = Array Max & Min(array=w1992) -> (max value=w2001:dbl, min value=w2000:dbl)  [unwired: 2 out]
                      n945 = Divide(x="Range limit\nS2.4 2", y=2.0) -> (x/y=w2017:dbl)
                      n946 = Divide(x="Range limit\nS2.4 2", y=2.05) -> (x/y=w2018:dbl)
                      n947 = Add(x="Base line \nS2.4 2", y=w2017) -> (x+y=w1993:dbl)
                      n948 = Subtract(x="Base line \nS2.4 2", y=w2017) -> (x-y=w1994:dbl)
                      n949 = Subtract(x="Base line \nS2.4 2", y=w2018) -> (x-y=w1999:dbl)
                      n950 = call "EventstoGraph (SubVI).vi"("Numerisch 2"=w2000, "Array 3"=w1986, "Numerisch"=w2001, "Array (Eingang)"=dbl[][] [], "Numerisch 3"=w1999) -> ("Array (Ausgang)"=w2003:dbl[][])  [unwired: 6 in]
                      n951 = Array Max & Min(array=w1992) -> (max value=w2013:dbl, min value=w2014:dbl)  [unwired: 2 out]
                      n952 = call "GraphLimit01.vi"("Numeric 2"=w1994, "Numeric"=w1993, "Array in"=w1991, "Array 3"=dbl[] []) -> ("Array out"=w2008:dbl[])  [unwired: 7 in]
                      n953 = Build Array("Base line \nS2.4 2", "Base line \nS2.4 2") -> (w2010:dbl[])
                      n954 = Build Array(w2013, w2014) -> (w2011:dbl[])
                      n955 = Build Array(w1993, w1994) -> (w2012:dbl[])
                      n956 = Index Array(array=w2003, index (col)=0 ("Index (Zeile)")) -> (element=w2004:dbl[])  [unwired: 1 in]
                      n957 = Index Array(array=w2003, index (col)=1 ("Index (Zeile)")) -> (element=w2002:dbl[])  [unwired: 1 in]
                      n958 = Bundle(w2011, w2012) -> (w1997:cluster{dbl[], dbl[]})  [unwired: 1 in]
                      n959 = Bundle(w2011, w2010) -> (w1998:cluster{dbl[], dbl[]})  [unwired: 1 in]
                      n960 = Bundle(w1992, "Array out"=w2008) -> (w1996:cluster{dbl[], "Array out":dbl[]})  [unwired: 1 in]
                      n961 = Bundle("Array (Ausgang)"=w2004, "Array (Ausgang)"=w2002) -> (w1995:T16)  [unwired: 1 in]
                      n962 = Build Array(w1998, w1997, w1996, w1995) -> (w1988:T17)
                      n963 = case shown="True" w1987 {
                        tunnel: w1988 -> [_ w2019]
                        frame False {
                        }
                        frame True {
                          "Ion flux (buffer corr.) SISE channel 2" <- w2019
                        }
                      }
                    }
                  }
                }
              }
              n964 = Equal?(x=w1855, y=u16 0) -> (x = y?=w1849:bool)
              n965 = Or(x=w1843, y=w1849) -> (x .or. y?=w1848:bool)
              n966 = Select(t=T9."Enabled" ("Disabled"), s=w1848, f=T9."Disabled and Grayed Out") -> (s? t:f=w1864:T9)
              n967 = property on="Buffer species ch2" class="Bool (strict)"("DisabledEnum"=w1864) -> ()  [unwired: 2 in, 2 out]
              n968 = Equal?(x=w1855, y=u16 1) -> (x = y?=w1846:bool)
              n969 = Or(x=w1843, y=w1846) -> (x .or. y?=w1847:bool)
              n970 = Select(t=T9."Enabled" ("Disabled"), s=w1847, f=T9."Disabled and Grayed Out") -> (s? t:f=w1860:T9)
              n971 = property on="Buffer conc. ch2" class="Bool (strict)"("DisabledEnum"=w1860) -> ()  [unwired: 2 in, 2 out]
              n972 = Equal?(x=w1855, y=u16 2) -> (x = y?=w1844:bool)
              n973 = Or(x=w1843, y=w1844) -> (x .or. y?=w1845:bool)
              n974 = Select(t=T9."Enabled" ("Disabled"), s=w1845, f=T9."Disabled and Grayed Out") -> (s? t:f=w1828:T9)
              n975 = property on="Update graphs (buffer corr.) ch2" class="Bool (strict)"("DisabledEnum"=w1828) -> ()  [unwired: 2 in, 2 out]
            }
            frame "SISE channel 1, buffer corr." {
              n976 = local read "Buffer species ch1"() -> (w2075:bool)
              n977 = local read "Buffer conc. ch1"() -> (w2074:bool)
              n978 = Index Array(array=w2070, index (col)=12 ("disabled index (col)")) -> (element=w2072:dbl[])  [unwired: 1 in]
              n979 = Unbundle(w2080) -> (w2090:bool[])  [unwired: 1 out]
              n980 = Add Array Elements(numeric array=w2072) -> (sum=w2071:dbl)
              n981 = Not Equal To 0?(x=w2071) -> (x != 0?=w2069:bool)
              n982 = And(x=w2075, y=w2074) -> (x .and. y?=w2065:bool)
              n983 = Index Array(array=w2090, index=8 ("Index")) -> (element=w2088:bool)
              n984 = And(x=w2065, y=w2069) -> (x .and. y?=w2068:bool)
              "Update graphs (buffer corr.) ch1" <- w2068
              n985 = Index Array(array=w2090, index=10 ("Index")) -> (element=w2089:bool)
              n986 = And(x=w2088, y=w2089) -> (x .and. y?=w2081:bool)
              n987 = case shown="\"Update graphs\"" "Module selection ch1 (buffer corr.)" {
                tunnel: [0 1 2] -> w2093
                tunnel: w2070 -> [w2107 w2134 w2172]
                tunnel: [w2107 w2134 w2170] -> w2079
                tunnel: w2078 -> [_ _ w2174]
                tunnel: w2077 -> [w2106 w2133 w2173]
                tunnel: [w2106 w2133 w2171] -> w2076
                tunnel: w2065 -> [_ _ w2140]
                tunnel: w2068 -> [_ _ w2142]
                tunnel: w2066 -> [_ _ w2145]
                frame "Buffer species", Default {
                  n988 = case shown="\"Mes\"" "Select buffer ch1" {
                    tunnel: ["" "Mes" "Malate (pH 5)" "Citrate (pH 5)" "TRIS" "HEPES"] -> w2110
                    tunnel: [0.0 6.2 5.1 4.8 8.2 7.5] -> w2113
                    tunnel: [0.0 2.9 3.2 2.5 3.2 2.4] -> w2112
                    frame "none", Default {
                    }
                    frame "Mes" {
                    }
                    frame "Malate (pH 5)" {
                    }
                    frame "Citrate (pH 5)" {
                    }
                    frame "TRIS" {
                    }
                    frame "HEPES" {
                    }
                  }
                  "pKs ch1" <- w2113
                  "Buffer Mobilty ch1" <- w2112
                  n989 = Not Equal?(x="", y=w2110) -> (x != y?=→"Buffer species ch1":bool)
                }
                frame "Buffer conc." {
                  n990 = Not Equal To 0?(x="Buffer conc. ch1 (mM)") -> (x != 0?=→"Buffer conc. ch1":bool)
                }
                frame "Update graphs" {
                  n991 = Not(x=w2142) -> (.not. x?=w2141:bool)
                  n992 = And(x=w2140, y=w2141) -> (x .and. y?=w2139:bool)
                  n993 = Index Array(array=w2172, index (col)=10 ("Deaktivierter Index (Spalte)")) -> (element=w2190:dbl[])  [unwired: 1 in]
                  n994 = local write "Zoom from start (Buffer corr. modul) ch2"("Zoom from start (Buffer corr. modul) ch1") -> ()
                  n995 = local write "Zoom from end (Buffer corr. modul) ch2"("Zoom from end (Buffer corr. modul) ch1") -> ()
                  n996 = for {
                    tunnel: w2174 -> [w2221] mode=indexing
                    shift-right: [w2223] -> w2175
                    shift-left: dbl[] [] -> [w2222]
                    n997 = Unbundle(w2221) -> (w2218:dbl)  [unwired: 1 out]
                    n998 = Divide(x=w2218, y=60.0) -> (x/y=w2219:dbl)
                    n999 = Insert Into Array(array=w2222, new element=w2219) -> (w2223:dbl[])  [unwired: 1 in]
                  }
                  n1000 = local read "Ion conc. ch1 (mM)"() -> (w2138:dbl)
                  n1001 = local read "pKs ch1"() -> (w2195:dbl)
                  n1002 = local read "Buffer Mobilty ch1"() -> (w2192:dbl)
                  n1003 = local read "Ion mobilty ch1"() -> (w2193:dbl)
                  n1004 = local read "Buffer conc. ch1 (mM)"() -> (w2194:dbl)
                  n1005 = Multiply(x="Zoom from end (Buffer corr. modul) ch1", y=-1.0) -> (x*y=w2162:dbl)
                  n1006 = Add(x="Zoom from start (Buffer corr. modul) ch1", y=w2162) -> (x+y=w2156:dbl)
                  n1007 = feedback #6() -> (w2158:dbl)  [unwired: 1 in]
                  n1008 = Greater Or Equal?(x=w2156, y=0.0) -> (x >= y?=w2157:bool)
                  n1009 = case shown="True" w2139 {
                    tunnel: dbl[] [] -> [_ w2264]
                    tunnel: w2192 -> [_ w2277]
                    tunnel: w2193 -> [_ w2278]
                    tunnel: w2195 -> [_ w2275]
                    tunnel: w2194 -> [_ w2274]
                    tunnel: w2190 -> [_ w2262]
                    tunnel: w2138 -> [_ w2263]
                    tunnel: w2173 -> [w2259 w2269]
                    tunnel: w2172 -> [w2258 w2268]
                    tunnel: [w2259 w2266] -> w2171
                    tunnel: [w2258 w2265] -> w2170
                    frame False {
                    }
                    frame True {
                      n1010 = Divide(x=w2277, y=w2278) -> (x/y=w2276:dbl)
                      n1011 = for {
                        tunnel: w2276 -> [w2287]
                        tunnel: w2275 -> [w2297]
                        tunnel: w2274 -> [w2291]
                        shift-right: [w2282] -> w2261
                        shift-left: w2264 -> [w2283]
                        tunnel: w2262 -> [w2281] mode=indexing
                        tunnel: w2263 -> [w2280]
                        n1012 = Multiply(x=w2280, y=0.001) -> (x*y=w2301:dbl)
                        n1013 = Multiply(x=w2291, y=0.001) -> (x*y=w2288:dbl)
                        n1014 = Logarithm Base 10(1:w2301) -> (0:w2300:dbl)
                        n1015 = Multiply(x=w2300, y=-1.0) -> (x*y=w2298:dbl)
                        n1016 = Power Of 10(x=w2298) -> (10^x=w2295:dbl)
                        n1017 = Power Of 10(x=w2297) -> (10^x=w2292:dbl)
                        n1018 = Add(x=w2295, y=w2292) -> (x+y=w2296:dbl)
                        n1019 = Divide(x=w2295, y=w2296) -> (x/y=w2294:dbl)
                        n1020 = Square(x=w2294) -> (x^2=w2293:dbl)
                        n1021 = Multiply(x=w2293, y=w2292) -> (x*y=w2289:dbl)
                        n1022 = Multiply(x=w2289, y=w2288) -> (x*y=w2286:dbl)
                        n1023 = Multiply(x=w2286, y=w2287) -> (x*y=w2285:dbl)
                        n1024 = Multiply(x=w2285, y=w2281) -> (x*y=w2284:dbl)
                        n1025 = Add(x=w2284, y=w2281) -> (x+y=w2279:dbl)
                        n1026 = Insert Into Array(array=w2283, new element=w2279) -> (w2282:dbl[])  [unwired: 1 in]
                      }
                      n1027 = Unbundle(w2269) -> (w2267:string[], w2272:bool[])
                      n1028 = Replace Array Subset(array=w2272, new element=TRUE, index=12 ("Index")) -> (w2273:bool[])
                      n1029 = Bundle(w2267, w2273) -> (w2266:cluster{string[], bool[]})  [unwired: 1 in]
                      n1030 = Insert Into Array(array=w2268, index (col)=12 ("Deaktivierter Index (Spalte)"), new element=w2261) -> (w2265:dbl[][])  [unwired: 1 in]
                    }
                  }
                  n1031 = case shown="True" w2157 {
                    tunnel: "Zoom from start (Buffer corr. modul) ch1" -> [w2199 w2202]
                    tunnel: [w2198 w2202] -> w2147
                    tunnel: w2158 -> [w2198 w2204]
                    tunnel: "Zoom from end (Buffer corr. modul) ch1" -> [_ w2201]
                    tunnel: [w2199 w2202] -> w2163
                    tunnel: [w2197 w2200] -> w2164
                    tunnel: "Zoom from end (Buffer corr. modul) ch1" -> [w2197 w2200]
                    frame False {
                    }
                    frame True {
                      n1032 = Not Equal?(x=w2204, y=w2202) -> (x != y?=w2203:bool)
                      n1033 = case shown="False" w2203 {
                        tunnel: w2202 -> [_ w2206]
                        tunnel: w2201 -> [w2205 _]
                        frame False {
                          n1034 = local write "Zoom from start (Buffer corr. modul) ch1"(w2205) -> ()
                        }
                        frame True {
                          n1035 = local write "Zoom from end (Buffer corr. modul) ch1"(w2206) -> ()
                        }
                      }
                    }
                  }
                  n1036 = feedback-in #6(w2147) -> ()
                  n1037 = Array Size(array=w2174) -> (size(s)=w2179:i32)
                  n1038 = Divide(x=w2179, y=10) -> (x/y=w2180:dbl)
                  n1039 = Multiply(x=w2180, y="Bildlaufleiste 3") -> (x*y=w2182:dbl)
                  n1040 = Array Subset(array=w2174, index=w2182) -> (w2183:cluster{dbl, string}[])  [unwired: 1 in]
                  n1041 = for {
                    shift-right: [w2216] -> w2178
                    shift-left: "" -> [w2217]
                    tunnel: w2183 -> [w2215] mode=indexing
                    n1042 = Unbundle(w2215) -> (w2213:dbl, w2210:string)
                    n1043 = Divide(x=w2213, y=60.0) -> (x/y=w2211:dbl)
                    n1044 = Number To Fractional String(number=w2211, precision (6)=i16 2 ("Genauigkeit (6)")) -> (F-format string=w2209:string)  [unwired: 2 in]
                    n1045 = Concatenate Strings(w2217, w2209, "min. ,", w2210, "\r") -> (w2216:string)
                  }
                  "?" <- w2178
                  n1046 = Subtract(x=w2164, y=w2163) -> (x-y=w2159:dbl)
                  n1047 = Index Array(array=w2145, index (col)=0 ("Deaktivierter Index (Spalte)")) -> (element=w2155:dbl[])  [unwired: 1 in]
                  n1048 = Divide(x=w2163, y=100.0) -> (x/y=w2161:dbl)
                  n1049 = Divide(x=w2159, y=100.0) -> (x/y=w2160:dbl)
                  n1050 = Array Size(array=w2155) -> (size(s)=w2165:i32)
                  n1051 = Multiply(x=w2165, y=w2161) -> (x*y=w2168:dbl)
                  n1052 = Multiply(x=w2165, y=w2160) -> (x*y=w2166:dbl)
                  n1053 = Add(x=w2166, y=2.0) -> (x+y=w2167:dbl)
                  n1054 = Subtract(x=w2168, y=2.0) -> (x-y=w2169:dbl)
                  n1055 = Array Subset(array=w2145, index (row)=w2169, length (row)=w2167) -> (w2146:dbl[][])  [unwired: 2 in]
                  n1056 = Index Array(array=w2146, index (col)=0 ("disabled index (col)")) -> (element=w2187:dbl[])  [unwired: 1 in]
                  n1057 = Index Array(array=w2146, index (col)=12 ("disabled index (col)")) -> (element=w2185:dbl[])  [unwired: 1 in]
                  n1058 = stacked-sequence {
                    tunnel: w2187 -> [w2230]
                    tunnel: w2175 -> [w2224]
                    tunnel: w2185 -> [w2229]
                    tunnel: w2142 -> [w2225]
                    frame #0 {
                      n1059 = Array Max & Min(array=w2230) -> (max value=w2239:dbl, min value=w2238:dbl)  [unwired: 2 out]
                      n1060 = Divide(x="Range limit\nS2.4 3", y=2.0) -> (x/y=w2255:dbl)
                      n1061 = Divide(x="Range limit\nS2.4 3", y=2.05) -> (x/y=w2256:dbl)
                      n1062 = Add(x="Base line \nS2.4 3", y=w2255) -> (x+y=w2231:dbl)
                      n1063 = Subtract(x="Base line \nS2.4 3", y=w2255) -> (x-y=w2232:dbl)
                      n1064 = Subtract(x="Base line \nS2.4 3", y=w2256) -> (x-y=w2237:dbl)
                      n1065 = call "EventstoGraph (SubVI).vi"("Numerisch 2"=w2238, "Array 3"=w2224, "Numerisch"=w2239, "Array (Eingang)"=dbl[][] [], "Numerisch 3"=w2237) -> ("Array (Ausgang)"=w2241:dbl[][])  [unwired: 6 in]
                      n1066 = Array Max & Min(array=w2230) -> (max value=w2251:dbl, min value=w2252:dbl)  [unwired: 2 out]
                      n1067 = call "GraphLimit01.vi"("Numeric 2"=w2232, "Numeric"=w2231, "Array in"=w2229, "Array 3"=dbl[] []) -> ("Array out"=w2246:dbl[])  [unwired: 7 in]
                      n1068 = Build Array("Base line \nS2.4 3", "Base line \nS2.4 3") -> (w2248:dbl[])
                      n1069 = Build Array(w2251, w2252) -> (w2249:dbl[])
                      n1070 = Build Array(w2231, w2232) -> (w2250:dbl[])
                      n1071 = Index Array(array=w2241, index (col)=0 ("Index (Zeile)")) -> (element=w2242:dbl[])  [unwired: 1 in]
                      n1072 = Index Array(array=w2241, index (col)=1 ("Index (Zeile)")) -> (element=w2240:dbl[])  [unwired: 1 in]
                      n1073 = Bundle(w2249, w2250) -> (w2235:cluster{dbl[], dbl[]})  [unwired: 1 in]
                      n1074 = Bundle(w2249, w2248) -> (w2236:cluster{dbl[], dbl[]})  [unwired: 1 in]
                      n1075 = Bundle(w2230, "Array out"=w2246) -> (w2234:cluster{dbl[], "Array out":dbl[]})  [unwired: 1 in]
                      n1076 = Bundle("Array (Ausgang)"=w2242, "Array (Ausgang)"=w2240) -> (w2233:T16)  [unwired: 1 in]
                      n1077 = Build Array(w2236, w2235, w2234, w2233) -> (w2226:T17)
                      n1078 = case shown="True" w2225 {
                        tunnel: w2226 -> [_ w2257]
                        frame False {
                        }
                        frame True {
                          "Ion flux (buffer corr.) SISE channel 1" <- w2257
                        }
                      }
                    }
                  }
                }
              }
              n1079 = Equal?(x=w2093, y=u16 0) -> (x = y?=w2087:bool)
              n1080 = Or(x=w2081, y=w2087) -> (x .or. y?=w2086:bool)
              n1081 = Select(t=T9."Enabled" ("Disabled"), s=w2086, f=T9."Disabled and Grayed Out") -> (s? t:f=w2102:T9)
              n1082 = property on="Buffer species ch1" class="Bool (strict)"("DisabledEnum"=w2102) -> ()  [unwired: 2 in, 2 out]
              n1083 = Equal?(x=w2093, y=u16 1) -> (x = y?=w2084:bool)
              n1084 = Or(x=w2081, y=w2084) -> (x .or. y?=w2085:bool)
              n1085 = Select(t=T9."Enabled" ("Disabled"), s=w2085, f=T9."Disabled and Grayed Out") -> (s? t:f=w2098:T9)
              n1086 = property on="Buffer conc. ch1" class="Bool (strict)"("DisabledEnum"=w2098) -> ()  [unwired: 2 in, 2 out]
              n1087 = Equal?(x=w2093, y=u16 2) -> (x = y?=w2082:bool)
              n1088 = Or(x=w2081, y=w2082) -> (x .or. y?=w2083:bool)
              n1089 = Select(t=T9."Enabled" ("Disabled"), s=w2083, f=T9."Disabled and Grayed Out") -> (s? t:f=w2067:T9)
              n1090 = property on="Update graphs (buffer corr.) ch1" class="Bool (strict)"("DisabledEnum"=w2067) -> ()  [unwired: 2 in, 2 out]
            }
          }
          n1091 = Unbundle(w1819) -> (w1817:dbl[][], w1818:dbl[], w1816:cluster{dbl, string}[])
        }
      }
    }
  }
